vi "Elevator_with_Semaphore.vi"() -> ()   [LabVIEW 2018]
uses:
  Elevator Constants.ctl
  Elevator Command.ctl
  Elevator Cabin.ctl
  Elevator Automate.ctl
  Elevator Panel.ctl
  Floors Schematic.ctl
panel:
  out "milliseconds to wait":u32=10
  out "# available":i32
  out "# waiting":i32
  out "size":i32
  out "# elements in Elevator Floor Queue":i32
  out "Position:Top":i32
  out "Elevator Floor Queue":u8[](array[numeric])
  out "Elevator Command Queue":T1[](array[typedef])
  in  "Elevator Automate":T2={"Elevator Panel Array"=[FALSE, FALSE, FALSE, FALSE, FALSE, FALSE, FALSE, FALSE, FALSE, FALSE, FALSE, FALSE], "Floor Array"=[FALSE, FALSE, FALSE, FALSE, FALSE, FALSE, FALSE, FALSE, FALSE, FALSE, FALSE, FALSE], "Elevator Command"=enum."Open Doors", "Target Floor"=0, "Forced Stop"=FALSE, "Cancel Delay"=FALSE, "Elevator Status"=enum."Stand By", "Update\nTarget Floor"=FALSE, "Take a Call"=FALSE, "Add Floor\nto Queue"=FALSE}
  in  "Elevator Panel":T3
  in  "Floors Schematic":T4={"Call 1"=FALSE, "Call 2"=FALSE, "Call 3"=FALSE, "Call 4"=FALSE, "Call 5"=FALSE, "Call 6"=FALSE, "Call 7"=FALSE, "Call 8"=FALSE, "Call 9"=FALSE, "Call 10"=FALSE, "Call 11"=FALSE, "Call 12"=FALSE, "Floor Position"=[0, 0, 0, 0, 0, 0, 0, 0, 0, 0, 0, 0]}
  in  "STOP":bool
  out "Elevator Cabin":T5 scale=0.0..100.0
  # "Данная версия программы не является рабоей!"
  # "12"
  # "11"
  # "10"
  # "9"
  # "8"
  # "7"
  # "6"
  # "5"
  # "4"
  # "3"
  # "2"
  # "1"
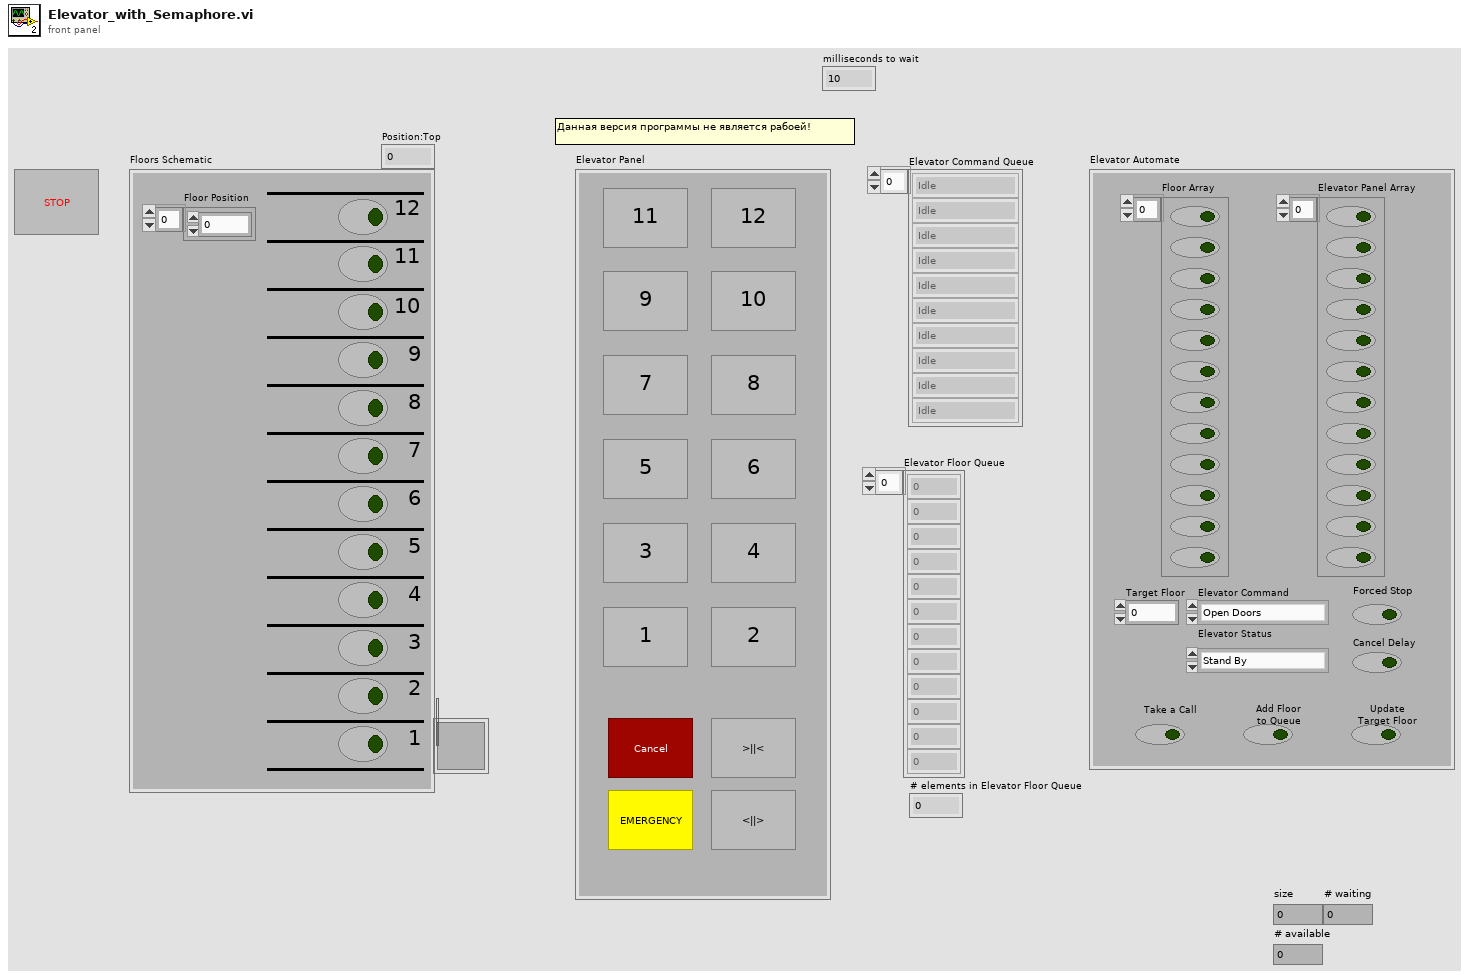
[diagram p1: front panel]
types:
  T1 = typedef "Elevator Command.ctl" = enum16{"Idle", "Short Delay", "Long Delay", "Cancel Delay", "Open Doors", "Close Doors", "Going Up", "Going Down", "Unpress Button"}
  T2 = typedef "Elevator Automate.ctl" = cluster{"Elevator Panel Array":bool[], "Floor Array":bool[], "Elevator Command":T1, "Target Floor":u8, "Forced Stop":bool, "Cancel Delay":bool, "Elevator Status":enum16{"Stand By", "Stop", "Going Up", "Going Down", "Cancel"}, "Update\nTarget Floor":bool, "Take a Call":bool, "Add Floor\nto Queue":bool}
  T3 = typedef "Elevator Panel.ctl" = cluster{"Open Doors":bool, "Close Doors":bool, "Floor 2":bool, "Floor 1":bool, "Floor 3":bool, "Floor 4":bool, "Floor 5":bool, "Floor 6":bool, "Floor 7":bool, "Floor 8":bool, "Floor 9":bool, "Floor 10":bool, "Floor 11":bool, "Floor 12":bool, "Emergency":bool, "Cancel":bool}
  T4 = typedef "Floors Schematic.ctl" = cluster{"Call 1":bool, "Call 2":bool, "Call 3":bool, "Call 4":bool, "Call 5":bool, "Call 6":bool, "Call 7":bool, "Call 8":bool, "Call 9":bool, "Call 10":bool, "Call 11":bool, "Call 12":bool, "Floor Position":i16[]}
  T5 = typedef "Elevator Cabin.ctl" = u8
  T6 = enum16{"Stand By", "Stop", "Going Up", "Going Down", "Cancel"}
  T7 = enum8{"Enabled", "Disabled", "Disabled and Grayed Out"}
  T8 = typedef "Semaphore RefNum" = refnum<k1>
  T9 = typedef "Elevator Constants.ctl" = u8
  T10 = enum16{"Stand By", "Stop", "Going Up", "Going Down"}
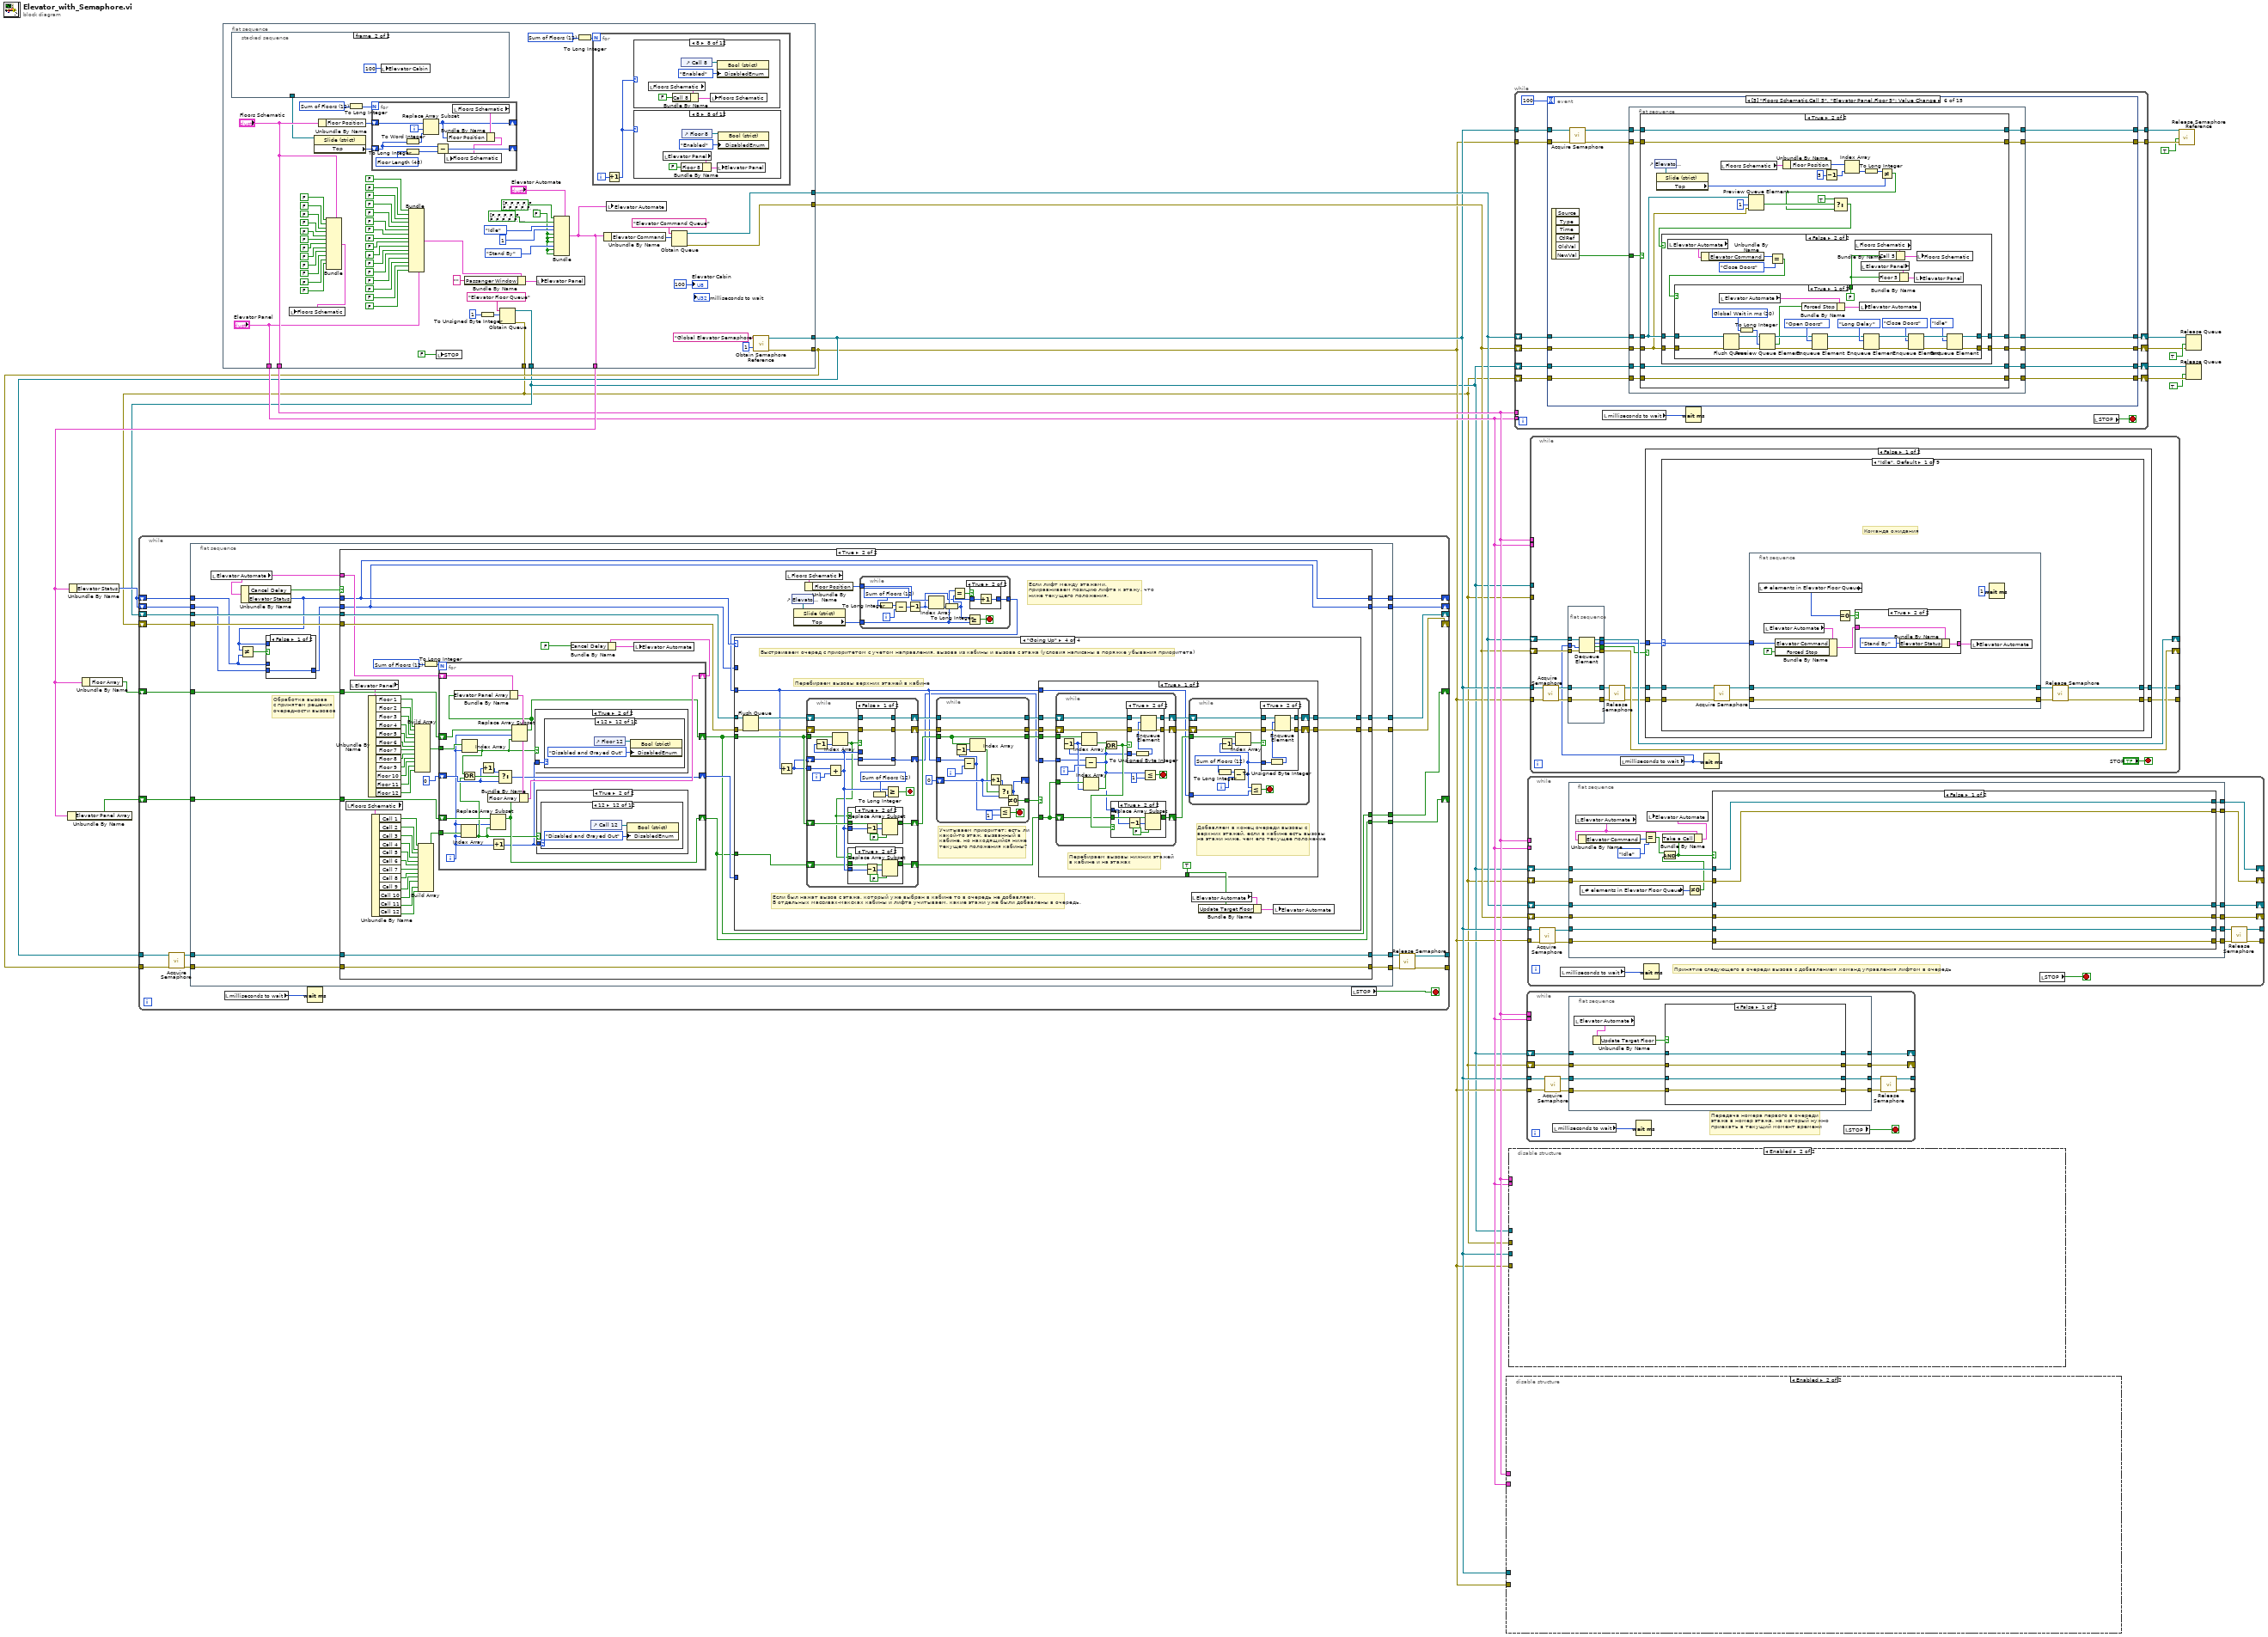
[diagram p0: block diagram]
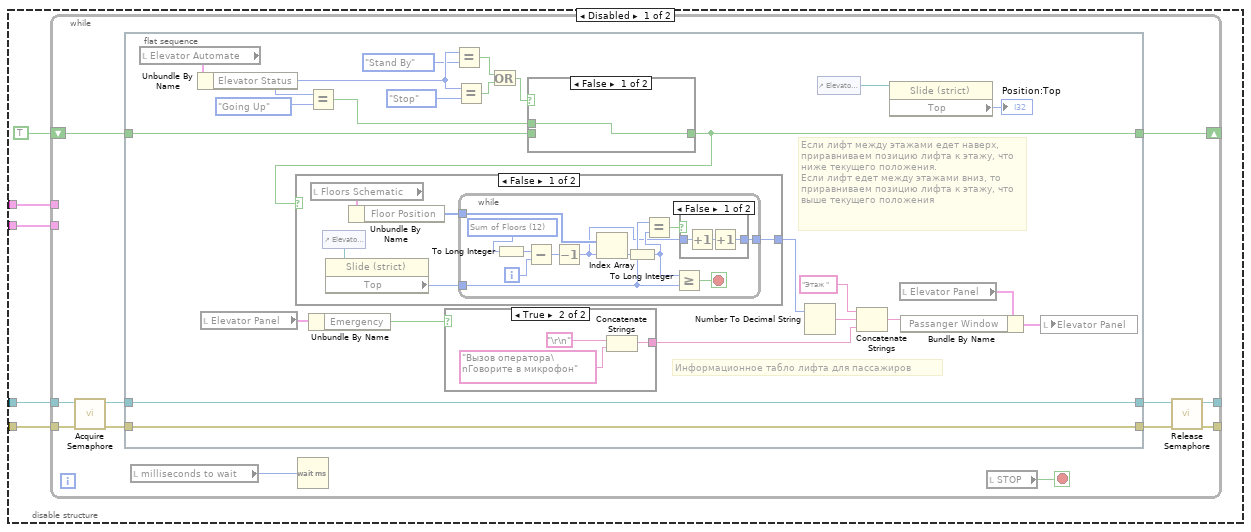
[diagram p2: hidden frame]
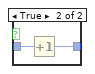
[diagram p4: hidden frame]
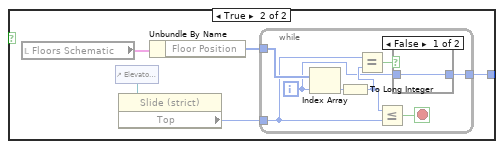
[diagram p5: hidden frame]
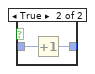
[diagram p6: hidden frame]
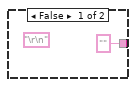
[diagram p7: hidden frame]
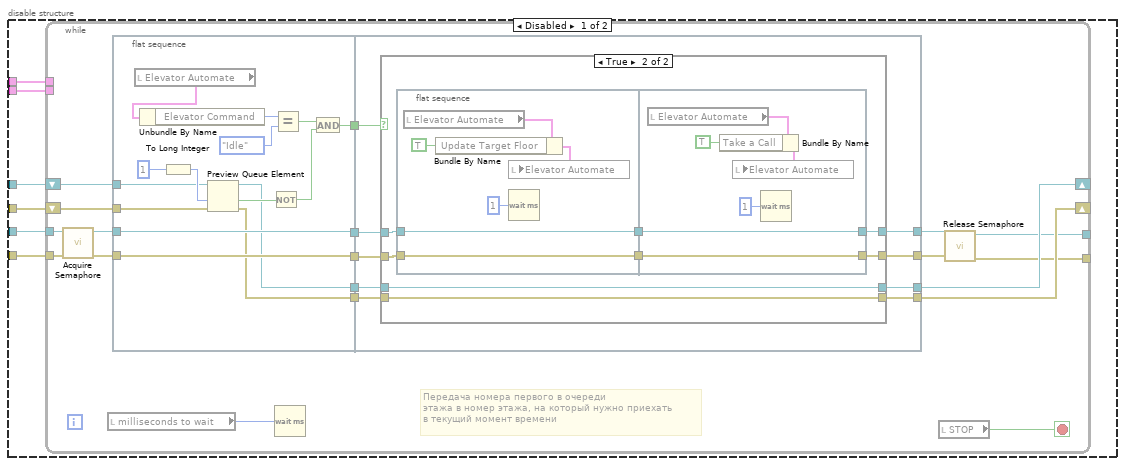
[diagram p8: hidden frame]
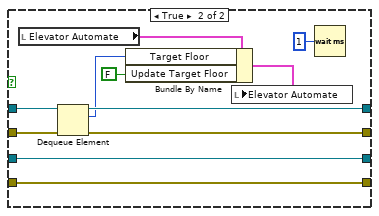
[diagram p10: hidden frame]
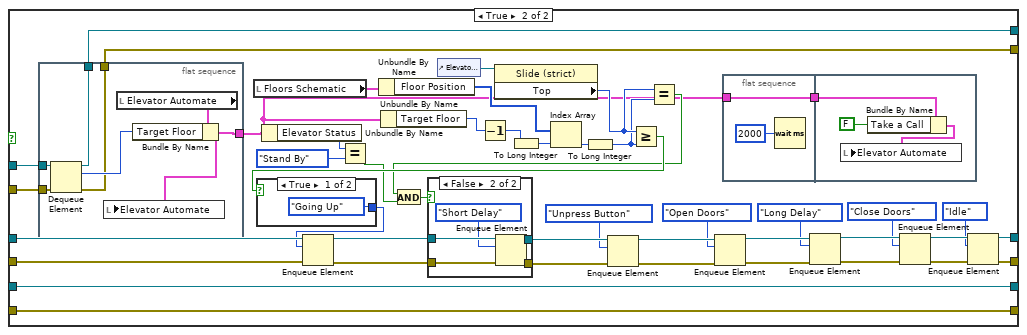
[diagram p11: hidden frame]
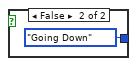
[diagram p13: hidden frame]
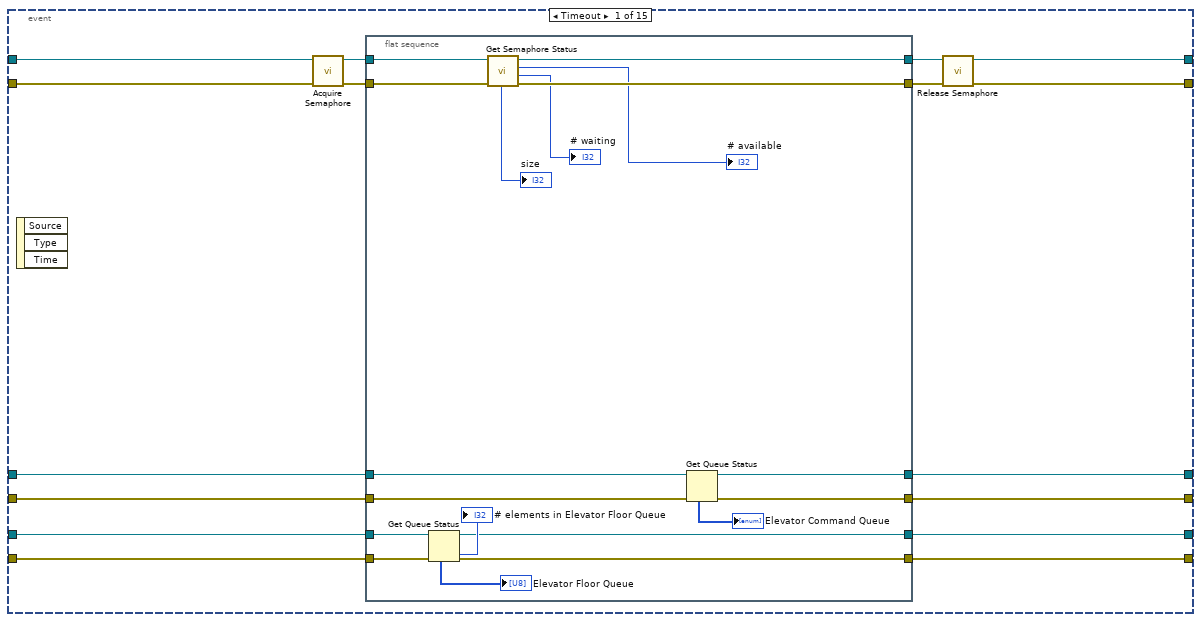
[diagram p14: hidden frame]
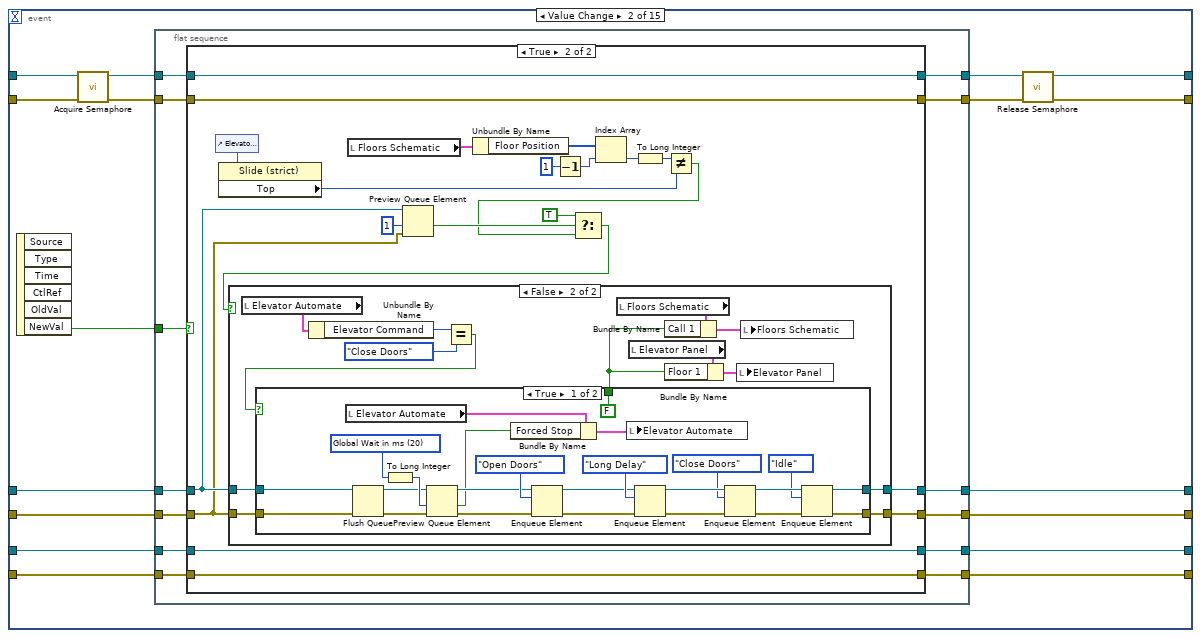
[diagram p15: hidden frame]
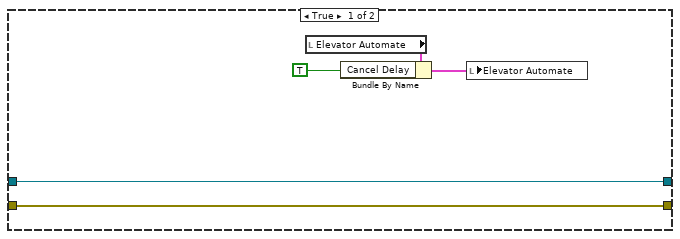
[diagram p17: hidden frame]
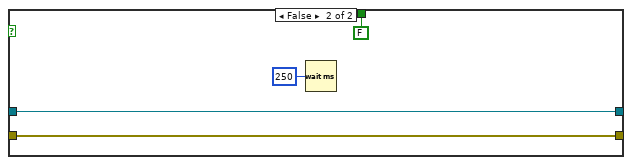
[diagram p18: hidden frame]
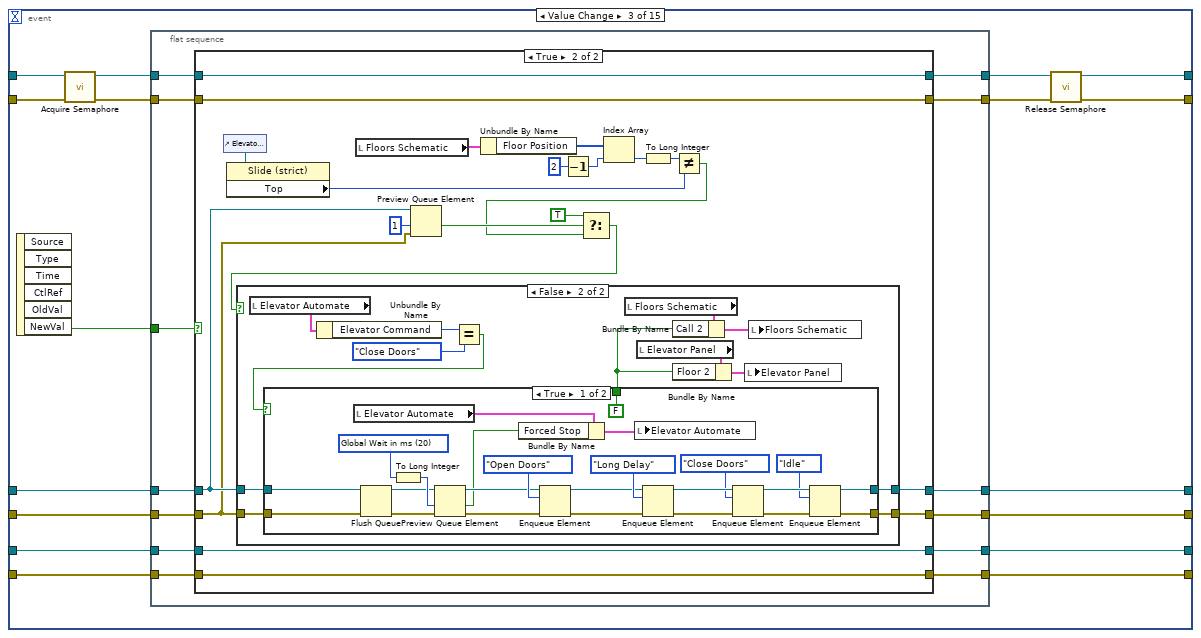
[diagram p19: hidden frame]
diagram:
  n1 = Unbundle By Name(w13) -> ("Elevator Panel Array"=w20:bool[])
  n2 = Unbundle By Name(w13) -> ("Elevator Status"=w12:T6)
  n3 = Unbundle By Name(w13) -> ("Floor Array"=w21:bool[])
  n4 = while {
    shift-right: [w38] -> _
    shift-left: w20 -> [w41]
    shift-right: [w37] -> _
    shift-left: w21 -> [w42]
    shift-right: [w35] -> _
    shift-left: w1 -> [w40]
    shift-right: [w36] -> _
    shift-left: w2 -> [w39]
    shift-right: [w34] -> _
    shift-left: w12 -> [w31]
    shift-right: [w32] -> _
    shift-left: w12 -> [w33]
    tunnel: w4 -> [w30]
    tunnel: w3 -> [w29]
    tunnel: [w24] -> _
    tunnel: [w23] -> _
    stop <- w43 stop-if-true
    n5 = call <vilib>:"Acquire Semaphore.vi"("error in (no error)"=w29, "semaphore"=w30) -> ("error out"=w28:errorcluster, "semaphore out"=w27:T8)  [unwired: 3 in, 1 out]
    n6 = flat-sequence {
      tunnel: [w59] -> w38
      tunnel: [w58] -> w37
      tunnel: [w57] -> w36
      tunnel: [w56] -> w35
      tunnel: [w55] -> w34
      tunnel: [w50] -> w32
      tunnel: w42 -> [w64]
      tunnel: w41 -> [w63]
      tunnel: w40 -> [w62]
      tunnel: w39 -> [w61]
      tunnel: w33 -> [w52]
      tunnel: w31 -> [w49]
      tunnel: w28 -> [w46]
      tunnel: w27 -> [w47]
      tunnel: [w45] -> w26
      tunnel: [w44] -> w25
      frame #0 {
        # "Обработка вызова\nс принятем решения\nочередности вызовов"
        n7 = local read "Elevator Automate"() -> (w54:T2)
        n8 = Unbundle By Name(w54) -> ("Cancel Delay"=w60:bool, "Elevator Status"=w51:T6)
        n9 = Not Equal?(x=w51, y=w52) -> (x != y?=w53:bool)
        n10 = case shown="False" w53 {
          tunnel: w51 -> [_ _]
          tunnel: w52 -> [_ w66]
          tunnel: w49 -> [w65 _]
          tunnel: [w65 w66] -> w48
          frame False {
          }
          frame True {
          }
        }
        n11 = case shown="True" w60 {
          tunnel: w64 -> [w71 w127]
          tunnel: w63 -> [w72 w126]
          tunnel: w62 -> [w73 w95]
          tunnel: w61 -> [w74 w94]
          tunnel: w51 -> [w70 w89]
          tunnel: [w74 w92] -> w57
          tunnel: [w73 w91] -> w56
          tunnel: [w72 w82] -> w59
          tunnel: [w71 w83] -> w58
          tunnel: w48 -> [w69 w81]
          tunnel: [w69 w81] -> w55
          tunnel: w54 -> [_ w90]
          tunnel: [w70 w89] -> w50
          tunnel: w47 -> [w68 w76]
          tunnel: w46 -> [w67 w75]
          tunnel: [w68 w76] -> w45
          tunnel: [w67 w75] -> w44
          frame False {
          }
          frame True {
            w97 = T9 12 items=["Floor Length"=48, "Sum of Floors"=12, "Floor Step in ms"=63, "Elevator Door Step in ms"=30, "Global Wait in ms"=20, "Event Wait in ms"=100] ("Elevator Constants")
            # "Если лифт между этажами,\nприравниваем позицию лифта к этажу, что ниже текущего положения."
            n12 = local read "Floors Schematic"() -> (w98:T4)
            n13 = local read "Elevator Panel"() -> (w99:T3)
            n14 = Unbundle By Name(w99) -> ("Floor 1"=w125:bool, "Floor 2"=w124:bool, "Floor 3"=w123:bool, "Floor 4"=w122:bool, "Floor 5"=w121:bool, "Floor 6"=w120:bool, "Floor 7"=w119:bool, "Floor 8"=w118:bool, "Floor 9"=w117:bool, "Floor 10"=w116:bool, "Floor 11"=w115:bool, "Floor 12"=w114:bool)
            n15 = Unbundle By Name(w98) -> ("Call 1"=w100:bool, "Call 2"=w112:bool, "Call 3"=w111:bool, "Call 4"=w110:bool, "Call 5"=w109:bool, "Call 6"=w108:bool, "Call 7"=w107:bool, "Call 8"=w106:bool, "Call 9"=w105:bool, "Call 10"=w104:bool, "Call 11"=w103:bool, "Call 12"=w102:bool)
            n16 = Build Array(w125, w124, w123, w122, w121, w120, w119, w118, w117, w116, w115, w114) -> (w113:bool[])
            n17 = Build Array(w100, w112, w111, w110, w109, w108, w107, w106, w105, w104, w103, w102) -> (w101:bool[])
            n18 = To Long Integer(number=w97) -> (32bit integer=w96:i32)
            n19 = for {
              N: w96 -> [_]
              tunnel: w113 -> [w998]
              tunnel: w101 -> [w997]
              shift-right: [w987] -> w82
              shift-left: w126 -> [w993]
              shift-right: [w988] -> w83
              shift-left: w127 -> [w994]
              shift-right: [w995] -> w84
              shift-left: w90 -> [w982]
              shift-right: [w990] -> w88
              shift-left: 0 -> [w989]
              i -> [w984]
              n20 = Index Array(array=w997, index=w984) -> (element=w986:bool)
              n21 = Index Array(array=w998, index=w984) -> (element=w985:bool)
              n22 = Or(x=w985, y=w986) -> (x .or. y?=w992:bool)
              n23 = Increment(x=w989) -> (x+1=w991:i32)
              n24 = Replace Array Subset(array=w993, new element=w986, index=w984) -> (w987:bool[])
              n25 = Increment(x=w984) -> (x+1=w983:i32)
              n26 = Select(t=w991, s=w992, f=w989) -> (s? t:f=w990:i32)
              n27 = Replace Array Subset(array=w994, new element=w985, index=w984) -> (w988:bool[])
              n28 = Bundle By Name(cluster=w982, "Elevator Panel Array"=w988) -> (w996:T2)
              n29 = Bundle By Name(cluster=w996, "Floor Array"=w987) -> (w995:T2)
              n30 = case shown="True" w985 {
                tunnel: w983 -> [_ w1024]
                frame False {
                }
                frame True {
                  n31 = case shown="12" w1024 {
                    frame 1, Default {
                      n32 = control-ref of="Floor 1"() -> (w1026:refnum<vi>)
                      n33 = property class="Bool (strict)"(reference=w1026, "DisabledEnum"=T7."Disabled and Grayed Out" ("Disabled")) -> ()  [unwired: 1 in, 2 out]
                    }
                    frame 2 {
                      n34 = control-ref of="Floor 2"() -> (w1028:refnum<vi>)
                      n35 = property class="Bool (strict)"(reference=w1028, "DisabledEnum"=T7."Disabled and Grayed Out" ("Disabled")) -> ()  [unwired: 1 in, 2 out]
                    }
                    frame 3 {
                      n36 = control-ref of="Floor 3"() -> (w1030:refnum<vi>)
                      n37 = property class="Bool (strict)"(reference=w1030, "DisabledEnum"=T7."Disabled and Grayed Out" ("Disabled")) -> ()  [unwired: 1 in, 2 out]
                    }
                    frame 4 {
                      n38 = control-ref of="Floor 4"() -> (w1032:refnum<vi>)
                      n39 = property class="Bool (strict)"(reference=w1032, "DisabledEnum"=T7."Disabled and Grayed Out" ("Disabled")) -> ()  [unwired: 1 in, 2 out]
                    }
                    frame 5 {
                      n40 = control-ref of="Floor 5"() -> (w1034:refnum<vi>)
                      n41 = property class="Bool (strict)"(reference=w1034, "DisabledEnum"=T7."Disabled and Grayed Out" ("Disabled")) -> ()  [unwired: 1 in, 2 out]
                    }
                    frame 6 {
                      n42 = control-ref of="Floor 6"() -> (w1036:refnum<vi>)
                      n43 = property class="Bool (strict)"(reference=w1036, "DisabledEnum"=T7."Disabled and Grayed Out" ("Disabled")) -> ()  [unwired: 1 in, 2 out]
                    }
                    frame 7 {
                      n44 = control-ref of="Floor 7"() -> (w1038:refnum<vi>)
                      n45 = property class="Bool (strict)"(reference=w1038, "DisabledEnum"=T7."Disabled and Grayed Out" ("Disabled")) -> ()  [unwired: 1 in, 2 out]
                    }
                    frame 8 {
                      n46 = control-ref of="Floor 8"() -> (w1040:refnum<vi>)
                      n47 = property class="Bool (strict)"(reference=w1040, "DisabledEnum"=T7."Disabled and Grayed Out" ("Disabled")) -> ()  [unwired: 1 in, 2 out]
                    }
                    frame 9 {
                      n48 = control-ref of="Floor 9"() -> (w1042:refnum<vi>)
                      n49 = property class="Bool (strict)"(reference=w1042, "DisabledEnum"=T7."Disabled and Grayed Out" ("Disabled")) -> ()  [unwired: 1 in, 2 out]
                    }
                    frame 10 {
                      n50 = control-ref of="Floor 10"() -> (w1044:refnum<vi>)
                      n51 = property class="Bool (strict)"(reference=w1044, "DisabledEnum"=T7."Disabled and Grayed Out" ("Disabled")) -> ()  [unwired: 1 in, 2 out]
                    }
                    frame 11 {
                      n52 = control-ref of="Floor 11"() -> (w1046:refnum<vi>)
                      n53 = property class="Bool (strict)"(reference=w1046, "DisabledEnum"=T7."Disabled and Grayed Out" ("Disabled")) -> ()  [unwired: 1 in, 2 out]
                    }
                    frame 12 {
                      n54 = control-ref of="Floor 12"() -> (w1048:refnum<vi>)
                      n55 = property class="Bool (strict)"(reference=w1048, "DisabledEnum"=T7."Disabled and Grayed Out" ("Disabled")) -> ()  [unwired: 1 in, 2 out]
                    }
                  }
                }
              }
              n56 = case shown="True" w986 {
                tunnel: w983 -> [_ w999]
                frame False {
                }
                frame True {
                  n57 = case shown="12" w999 {
                    frame 1, Default {
                      n58 = control-ref of="Call 1"() -> (w1001:refnum<vi>)
                      n59 = property class="Bool (strict)"(reference=w1001, "DisabledEnum"=T7."Disabled and Grayed Out" ("Disabled")) -> ()  [unwired: 1 in, 2 out]
                    }
                    frame 2 {
                      n60 = control-ref of="Call 2"() -> (w1003:refnum<vi>)
                      n61 = property class="Bool (strict)"(reference=w1003, "DisabledEnum"=T7."Disabled and Grayed Out" ("Disabled")) -> ()  [unwired: 1 in, 2 out]
                    }
                    frame 3 {
                      n62 = control-ref of="Call 3"() -> (w1005:refnum<vi>)
                      n63 = property class="Bool (strict)"(reference=w1005, "DisabledEnum"=T7."Disabled and Grayed Out" ("Disabled")) -> ()  [unwired: 1 in, 2 out]
                    }
                    frame 4 {
                      n64 = control-ref of="Call 4"() -> (w1007:refnum<vi>)
                      n65 = property class="Bool (strict)"(reference=w1007, "DisabledEnum"=T7."Disabled and Grayed Out" ("Disabled")) -> ()  [unwired: 1 in, 2 out]
                    }
                    frame 5 {
                      n66 = control-ref of="Call 5"() -> (w1009:refnum<vi>)
                      n67 = property class="Bool (strict)"(reference=w1009, "DisabledEnum"=T7."Disabled and Grayed Out" ("Disabled")) -> ()  [unwired: 1 in, 2 out]
                    }
                    frame 6 {
                      n68 = control-ref of="Call 6"() -> (w1011:refnum<vi>)
                      n69 = property class="Bool (strict)"(reference=w1011, "DisabledEnum"=T7."Disabled and Grayed Out" ("Disabled")) -> ()  [unwired: 1 in, 2 out]
                    }
                    frame 7 {
                      n70 = control-ref of="Call 7"() -> (w1013:refnum<vi>)
                      n71 = property class="Bool (strict)"(reference=w1013, "DisabledEnum"=T7."Disabled and Grayed Out" ("Disabled")) -> ()  [unwired: 1 in, 2 out]
                    }
                    frame 8 {
                      n72 = control-ref of="Call 8"() -> (w1015:refnum<vi>)
                      n73 = property class="Bool (strict)"(reference=w1015, "DisabledEnum"=T7."Disabled and Grayed Out" ("Disabled")) -> ()  [unwired: 1 in, 2 out]
                    }
                    frame 9 {
                      n74 = control-ref of="Call 9"() -> (w1017:refnum<vi>)
                      n75 = property class="Bool (strict)"(reference=w1017, "DisabledEnum"=T7."Disabled and Grayed Out" ("Disabled")) -> ()  [unwired: 1 in, 2 out]
                    }
                    frame 10 {
                      n76 = control-ref of="Call 10"() -> (w1019:refnum<vi>)
                      n77 = property class="Bool (strict)"(reference=w1019, "DisabledEnum"=T7."Disabled and Grayed Out" ("Disabled")) -> ()  [unwired: 1 in, 2 out]
                    }
                    frame 11 {
                      n78 = control-ref of="Call 11"() -> (w1021:refnum<vi>)
                      n79 = property class="Bool (strict)"(reference=w1021, "DisabledEnum"=T7."Disabled and Grayed Out" ("Disabled")) -> ()  [unwired: 1 in, 2 out]
                    }
                    frame 12 {
                      n80 = control-ref of="Call 12"() -> (w1023:refnum<vi>)
                      n81 = property class="Bool (strict)"(reference=w1023, "DisabledEnum"=T7."Disabled and Grayed Out" ("Disabled")) -> ()  [unwired: 1 in, 2 out]
                    }
                  }
                }
              }
            }
            n82 = Bundle By Name(cluster=w84, "Cancel Delay"=FALSE ("Add Floor to Queue")) -> (w85:T2)
            n83 = local write "Elevator Automate"(w85) -> ()
            n84 = local read "Floors Schematic"() -> (w79:T4)
            n85 = control-ref of="Elevator Cabin"() -> (w80:refnum<vi>)
            n86 = property class="Slide (strict)"(reference=w80) -> ("Top"=w77:i32)  [unwired: 1 in, 2 out]
            n87 = Unbundle By Name(w79) -> ("Floor Position"=w78:i16[])
            n88 = while {
              tunnel: w78 -> [w137]
              tunnel: w77 -> [w135]
              tunnel: [w134] -> w87
              i -> [w132]
              stop <- w133 stop-if-true
              w130 = T9 12 items=["Floor Length"=48, "Sum of Floors"=12, "Floor Step in ms"=63, "Elevator Door Step in ms"=30, "Global Wait in ms"=20, "Event Wait in ms"=100] ("Elevator Constants")
              n89 = To Long Integer(number=w130) -> (32bit integer=w131:i32)
              n90 = Subtract(x=w131, y=w132) -> (x-y=w129:i32)
              n91 = Decrement(x=w129) -> (x-1=w128:i32)
              n92 = Index Array(array=w137, index=w128) -> (element=w138:i16)
              n93 = To Long Integer(number=w138) -> (32bit integer=w136:i32)
              n94 = Equal?(x=w135, y=w136) -> (x = y?=w139:bool)
              n95 = Greater Or Equal?(x=w136, y=w135) -> (x >= y?=w133:bool)
              n96 = case shown="True" w139 {
                tunnel: w128 -> [w140 w142]
                tunnel: [w140 w141] -> w134
                frame False {
                }
                frame True {
                  n97 = Increment(x=w142) -> (x+1=w141:i32)
                }
              }
            }
            n98 = case shown="\"Going Up\"" w89 {
              tunnel: w94 -> [w161 w281 w651 w827]
              tunnel: w95 -> [w160 w282 w652 w828]
              tunnel: w83 -> [w148 w286 w638 w830]
              tunnel: w82 -> [w146 w284 w639 w829]
              tunnel: w87 -> [w147 w285 w637 w811]
              tunnel: [w150 w288 w654 w832] -> w92
              tunnel: [w149 w287 w653 w831] -> w91
              tunnel: w81 -> [_ w283 _ _]
              tunnel: w88 -> [w143 _ _ _]
              frame "Stand By", Default {
                # "Если было одновременно несколько\nвызовов, то повторно обрабатываем\nочередь с учетом направления\nдвижения лифта"
                # "Перебираем вызовы верхних этажей в кабине"
                # "Перебираем вызовы на нижних этажах"
                # "Перебираем вызовы на верхних этажах"
                # "Перебираем вызовы нижних этажей в кабине"
                # "Выбираем приоритетный вызов"
                n99 = while {
                  tunnel: w148 -> [w177]
                  shift-right: [w174] -> w155
                  shift-left: w161 -> [w176]
                  shift-right: [w175] -> w154
                  shift-left: w160 -> [w178]
                  tunnel: w147 -> [w166]
                  tunnel: [w169] -> w153
                  i -> [w165]
                  stop <- w173 stop-if-true
                  w171 = T9 12 items=["Floor Length"=48, "Sum of Floors"=12, "Floor Step in ms"=63, "Elevator Door Step in ms"=30, "Global Wait in ms"=20, "Event Wait in ms"=100] ("Elevator Constants")
                  n100 = Add(x=w166, y=w165) -> (x+y=w167:i32)
                  n101 = Decrement(x=w167) -> (x-1=w168:i32)
                  n102 = Index Array(array=w177, index=w168) -> (element=w169:bool)
                  n103 = To Long Integer(number=w171) -> (32bit integer=w172:i32)
                  n104 = case shown="True" w169 {
                    tunnel: w176 -> [w180 w186]
                    tunnel: w178 -> [w179 w185]
                    tunnel: [w179 w184] -> w175
                    tunnel: [w180 w183] -> w174
                    tunnel: w167 -> [_ w182]
                    frame False {
                    }
                    frame True {
                      n105 = To Unsigned Byte Integer(number=w182) -> (unsigned 8bit integer=w181:u8)
                      n106 = Enqueue Element(queue=w186, element=w181, error in (no error)=w185) -> (queue out=w183:refnum<queue>, error out=w184:errorcluster)  [unwired: 1 in, 1 out]
                    }
                  }
                  n107 = Greater Or Equal?(x=w167, y=w172) -> (x >= y?=w170:bool)
                  n108 = Or(x=w169, y=w170) -> (x .or. y?=w173:bool)
                }
                n109 = Greater?(x=w143, y=1) -> (0:w145:bool)
                n110 = case shown="True" w145 {
                  frame True {
                    n111 = local read "Elevator Automate"() -> (w164:T2)
                    n112 = Bundle By Name(cluster=w164, "Cancel Delay"=TRUE ("Add Floor to Queue")) -> (w162:T2)
                    n113 = local write "Elevator Automate"(w162) -> ()
                  }
                  frame False {
                  }
                }
                n114 = case shown="False" w153 {
                  selector: w153 -> [w250 _]
                  tunnel: w154 -> [w248 w257]
                  tunnel: w155 -> [w249 w256]
                  tunnel: w147 -> [_ w255]
                  tunnel: w148 -> [_ w254]
                  tunnel: [w250 w253] -> w152
                  tunnel: [w249 w252] -> w157
                  tunnel: [w248 w251] -> w156
                  frame True {
                  }
                  frame False {
                    n115 = while {
                      tunnel: w254 -> [w269]
                      shift-right: [w266] -> w252
                      shift-left: w256 -> [w268]
                      shift-right: [w267] -> w251
                      shift-left: w257 -> [w270]
                      tunnel: w255 -> [w261]
                      tunnel: [w263] -> w253
                      i -> [w260]
                      stop <- w265 stop-if-true
                      n116 = Subtract(x=w261, y=w260) -> (x-y=w258:i32)
                      n117 = Decrement(x=w258) -> (x-1=w259:i32)
                      n118 = Index Array(array=w269, index=w259) -> (element=w263:bool)
                      n119 = case shown="True" w263 {
                        tunnel: w268 -> [w272 w278]
                        tunnel: w270 -> [w271 w277]
                        tunnel: [w271 w276] -> w267
                        tunnel: [w272 w275] -> w266
                        tunnel: w258 -> [_ w274]
                        frame False {
                        }
                        frame True {
                          n120 = To Unsigned Byte Integer(number=w274) -> (unsigned 8bit integer=w273:u8)
                          n121 = Enqueue Element(queue=w278, element=w273, error in (no error)=w277) -> (queue out=w275:refnum<queue>, error out=w276:errorcluster)  [unwired: 1 in, 1 out]
                        }
                      }
                      n122 = Less Or Equal?(x=w258, y=1) -> (x <= y?=w264:bool)
                      n123 = Or(x=w263, y=w264) -> (x .or. y?=w265:bool)
                    }
                  }
                }
                n124 = case shown="False" w152 {
                  selector: w152 -> [w218 _]
                  tunnel: w156 -> [w216 w225]
                  tunnel: w157 -> [w217 w224]
                  tunnel: w147 -> [_ w223]
                  tunnel: w146 -> [_ w222]
                  tunnel: [w218 w221] -> w151
                  tunnel: [w217 w220] -> w159
                  tunnel: [w216 w219] -> w158
                  frame True {
                  }
                  frame False {
                    n125 = while {
                      tunnel: w222 -> [w238]
                      shift-right: [w235] -> w220
                      shift-left: w224 -> [w237]
                      shift-right: [w236] -> w219
                      shift-left: w225 -> [w239]
                      tunnel: w223 -> [w229]
                      tunnel: [w230] -> w221
                      i -> [w228]
                      stop <- w234 stop-if-true
                      w232 = T9 12 items=["Floor Length"=48, "Sum of Floors"=12, "Floor Step in ms"=63, "Elevator Door Step in ms"=30, "Global Wait in ms"=20, "Event Wait in ms"=100] ("Elevator Constants")
                      n126 = Add(x=w229, y=w228) -> (x+y=w227:i32)
                      n127 = Decrement(x=w227) -> (x-1=w226:i32)
                      n128 = Index Array(array=w238, index=w226) -> (element=w230:bool)
                      n129 = To Long Integer(number=w232) -> (32bit integer=w233:i32)
                      n130 = case shown="True" w230 {
                        tunnel: w237 -> [w241 w247]
                        tunnel: w239 -> [w240 w246]
                        tunnel: [w240 w245] -> w236
                        tunnel: [w241 w244] -> w235
                        tunnel: w227 -> [_ w243]
                        frame False {
                        }
                        frame True {
                          n131 = To Unsigned Byte Integer(number=w243) -> (unsigned 8bit integer=w242:u8)
                          n132 = Enqueue Element(queue=w247, element=w242, error in (no error)=w246) -> (queue out=w244:refnum<queue>, error out=w245:errorcluster)  [unwired: 1 in, 1 out]
                        }
                      }
                      n133 = Greater Or Equal?(x=w227, y=w233) -> (x >= y?=w231:bool)
                      n134 = Or(x=w230, y=w231) -> (x .or. y?=w234:bool)
                    }
                  }
                }
                n135 = case shown="False" w151 {
                  tunnel: w158 -> [w187 w194]
                  tunnel: w159 -> [w188 w193]
                  tunnel: w146 -> [_ w192]
                  tunnel: [w188 w191] -> w150
                  tunnel: [w187 w190] -> w149
                  tunnel: w147 -> [_ w189]
                  frame True {
                  }
                  frame False {
                    n136 = while {
                      tunnel: w192 -> [w206]
                      shift-right: [w203] -> w191
                      shift-left: w193 -> [w205]
                      shift-right: [w204] -> w190
                      shift-left: w194 -> [w207]
                      tunnel: [w200] -> _
                      tunnel: w189 -> [w196]
                      i -> [w197]
                      stop <- w202 stop-if-true
                      n137 = Subtract(x=w196, y=w197) -> (x-y=w195:i32)
                      n138 = Decrement(x=w195) -> (x-1=w198:i32)
                      n139 = Index Array(array=w206, index=w198) -> (element=w200:bool)
                      n140 = case shown="True" w200 {
                        tunnel: w205 -> [w209 w215]
                        tunnel: w207 -> [w208 w214]
                        tunnel: [w208 w213] -> w204
                        tunnel: [w209 w212] -> w203
                        tunnel: w195 -> [_ w211]
                        frame False {
                        }
                        frame True {
                          n141 = To Unsigned Byte Integer(number=w211) -> (unsigned 8bit integer=w210:u8)
                          n142 = Enqueue Element(queue=w215, element=w210, error in (no error)=w214) -> (queue out=w212:refnum<queue>, error out=w213:errorcluster)  [unwired: 1 in, 1 out]
                        }
                      }
                      n143 = Less Or Equal?(x=w195, y=1) -> (x <= y?=w201:bool)
                      n144 = Or(x=w200, y=w201) -> (x .or. y?=w202:bool)
                    }
                  }
                }
              }
              frame "Stop" {
                # "Выстраиваем очеред с приоритетом с учетом направления, вызова из кабины и вызова с этажа (условия написаны в поряжке убывания приоритета)"
                n145 = Flush Queue(queue=w281, error in (no error)=w282) -> (queue out=w280:refnum<queue>, error out=w279:errorcluster)  [unwired: 1 out]
                n146 = case shown="\"Going Down\"" w283 {
                  tunnel: w280 -> [w311 w481]
                  tunnel: w279 -> [w310 w480]
                  tunnel: [w309 w479] -> w288
                  tunnel: [w308 w478] -> w287
                  tunnel: w286 -> [w306 w476]
                  tunnel: w285 -> [w290 w461]
                  tunnel: w284 -> [w302 w473]
                  frame "Going Up", Default {
                    # "Учитываем приоритет: есть ли\nкакой-то этаж, вызванный в кабине, но находящийся ниже\nтекущего положения кабины?"
                    # "Учитываем, на каком этаже\nсейчас находится лифт и убираем его из массивов-масок кабины и лифта"
                    # "Если был нажат вызов с этажа дома, который уже выбран в кабине то в очередь не добавляем.\nВ отдельных массивах-максках кабины и лифта учитываем, какие этажи уже были добавлены в очередь."
                    # "Перебираем вызовы верхних этажей в кабине"
                    n147 = Decrement(x=w290) -> (x-1=w301:i32)
                    n148 = Increment(x=w290) -> (x+1=w291:i32)
                    n149 = Replace Array Subset(array=w306, new element=FALSE ("new element/subarray"), index=w301) -> (w305:bool[])
                    n150 = Replace Array Subset(array=w302, new element=FALSE ("new element/subarray"), index=w301) -> (w303:bool[])
                    n151 = while {
                      tunnel: w305 -> [w429]
                      shift-right: [w436] -> w294
                      shift-left: w311 -> [w438]
                      shift-right: [w437] -> w297
                      shift-left: w310 -> [w439]
                      tunnel: w291 -> [w431]
                      shift-right: [w428] -> w299
                      shift-left: w305 -> [w427]
                      shift-right: [w425] -> w300
                      shift-left: w303 -> [w423]
                      shift-right: [w422] -> w289
                      shift-left: w291 -> [w421]
                      i -> [w433]
                      stop <- w432 stop-if-true
                      w430 = T9 12 items=["Floor Length"=48, "Sum of Floors"=12, "Floor Step in ms"=63, "Elevator Door Step in ms"=30, "Global Wait in ms"=20, "Event Wait in ms"=100] ("Elevator Constants")
                      n152 = Add(x=w431, y=w433) -> (x+y=w426:i32)
                      n153 = Decrement(x=w426) -> (x-1=w434:i32)
                      n154 = Index Array(array=w429, index=w434) -> (element=w424:bool)
                      n155 = case shown="True" w424 {
                        tunnel: w426 -> [_ w447]
                        tunnel: [w446 w449] -> w428
                        tunnel: w427 -> [w446 w448]
                        frame False {
                        }
                        frame True {
                          n156 = Decrement(x=w447) -> (x-1=w451:i32)
                          n157 = Replace Array Subset(array=w448, new element=FALSE ("new element/subarray"), index=w451) -> (w449:bool[])
                        }
                      }
                      n158 = case shown="True" w424 {
                        tunnel: [w440 w443] -> w425
                        tunnel: w423 -> [w440 w442]
                        tunnel: w426 -> [_ w441]
                        frame False {
                        }
                        frame True {
                          n159 = Decrement(x=w441) -> (x-1=w445:i32)
                          n160 = Replace Array Subset(array=w442, new element=FALSE ("new element/subarray"), index=w445) -> (w443:bool[])
                        }
                      }
                      n161 = case shown="True" w424 {
                        tunnel: w438 -> [w454 w460]
                        tunnel: w439 -> [w453 w459]
                        tunnel: [w453 w458] -> w437
                        tunnel: [w454 w457] -> w436
                        tunnel: w426 -> [_ w455]
                        tunnel: [w452 w455] -> w422
                        tunnel: w421 -> [w452 _]
                        frame False {
                        }
                        frame True {
                          n162 = To Unsigned Byte Integer(number=w455) -> (unsigned 8bit integer=w456:u8)
                          n163 = Enqueue Element(queue=w460, element=w456, error in (no error)=w459) -> (queue out=w457:refnum<queue>, error out=w458:errorcluster)  [unwired: 1 in, 1 out]
                        }
                      }
                      n164 = To Long Integer(number=w430) -> (32bit integer=w435:i32)
                      n165 = Greater Or Equal?(x=w426, y=w435) -> (x >= y?=w432:bool)
                    }
                    n166 = while {
                      tunnel: w299 -> [w415]
                      tunnel: [w415] -> w298
                      tunnel: w297 -> [w420]
                      tunnel: [w420] -> w296
                      tunnel: [w419] -> w295
                      tunnel: w294 -> [w419]
                      tunnel: w290 -> [w417]
                      shift-right: [w411] -> _
                      shift-left: 0 -> [w412]
                      tunnel: [w410] -> w292
                      i -> [w416]
                      stop <- w408 stop-if-true
                      n167 = Decrement(x=w417) -> (x-1=w418:i32)
                      n168 = Subtract(x=w418, y=w416) -> (x-y=w407:i32)
                      n169 = Decrement(x=w407) -> (x-1=w414:i32)
                      n170 = Index Array(array=w415, index=w414) -> (element=w406:bool)
                      n171 = Increment(x=w412) -> (x+1=w413:i32)
                      n172 = Less Or Equal?(x=w407, y=1) -> (x <= y?=w408:bool)
                      n173 = Select(t=w413, s=w406, f=w412) -> (s? t:f=w411:i32)
                      n174 = Not Equal To 0?(x=w411) -> (x != 0?=w410:bool)
                    }
                    n175 = case shown="False" w292 {
                      tunnel: [w320 w377] -> w309
                      tunnel: [w319 w376] -> w308
                      tunnel: w300 -> [w317 w381]
                      tunnel: w298 -> [w316 w380]
                      tunnel: w296 -> [w315 w379]
                      tunnel: w295 -> [w314 w378]
                      tunnel: w289 -> [w312 _]
                      tunnel: w290 -> [w313 _]
                      frame True {
                        # "Перебираем вызовы нижних этажей, начиная с самого высокого этажа, вызванного в кабине"
                        # "Если есть такой этаж, то добавляем в конец очереди вызовы верхних этажей дома"
                        n176 = while {
                          tunnel: w316 -> [w360]
                          shift-right: [w357] -> w322
                          shift-left: w314 -> [w359]
                          shift-right: [w358] -> w321
                          shift-left: w315 -> [w361]
                          tunnel: w312 -> [w350]
                          tunnel: w317 -> [w354]
                          shift-right: [w347] -> w318
                          shift-left: w317 -> [w348]
                          i -> [w352]
                          stop <- w355 stop-if-true
                          n177 = Decrement(x=w350) -> (x-1=w345:i32)
                          n178 = Subtract(x=w345, y=w352) -> (x-y=w344:i32)
                          n179 = Decrement(x=w344) -> (x-1=w351:i32)
                          n180 = Index Array(array=w360, index=w351) -> (element=w346:bool)
                          n181 = Index Array(array=w354, index=w351) -> (element=w353:bool)
                          n182 = Or(x=w346, y=w353) -> (x .or. y?=w349:bool)
                          n183 = case shown="True" w349 {
                            tunnel: w344 -> [_ w366]
                            tunnel: [w362 w364] -> w347
                            tunnel: w348 -> [w362 w363]
                            frame False {
                            }
                            frame True {
                              n184 = Decrement(x=w366) -> (x-1=w367:i32)
                              n185 = Replace Array Subset(array=w363, new element=FALSE ("new element/subarray"), index=w367) -> (w364:bool[])
                            }
                          }
                          n186 = case shown="True" w349 {
                            tunnel: w359 -> [w369 w375]
                            tunnel: w361 -> [w368 w374]
                            tunnel: [w368 w373] -> w358
                            tunnel: [w369 w372] -> w357
                            tunnel: w344 -> [_ w370]
                            frame False {
                            }
                            frame True {
                              n187 = To Unsigned Byte Integer(number=w370) -> (unsigned 8bit integer=w371:u8)
                              n188 = Enqueue Element(queue=w375, element=w371, error in (no error)=w374) -> (queue out=w372:refnum<queue>, error out=w373:errorcluster)  [unwired: 1 in, 1 out]
                            }
                          }
                          n189 = Less Or Equal?(x=w344, y=1) -> (x <= y?=w355:bool)
                        }
                        n190 = while {
                          tunnel: w318 -> [w334]
                          shift-right: [w331] -> w320
                          shift-left: w322 -> [w333]
                          shift-right: [w332] -> w319
                          shift-left: w321 -> [w335]
                          tunnel: w313 -> [w324]
                          i -> [w329]
                          stop <- w323 stop-if-true
                          w326 = T9 12 items=["Floor Length"=48, "Sum of Floors"=12, "Floor Step in ms"=63, "Elevator Door Step in ms"=30, "Global Wait in ms"=20, "Event Wait in ms"=100] ("Elevator Constants")
                          n191 = To Long Integer(number=w326) -> (32bit integer=w325:i32)
                          n192 = Subtract(x=w325, y=w329) -> (x-y=w328:i32)
                          n193 = Decrement(x=w328) -> (x-1=w327:i32)
                          n194 = Index Array(array=w334, index=w327) -> (element=w330:bool)
                          n195 = Less Or Equal?(x=w328, y=w324) -> (x <= y?=w323:bool)
                          n196 = case shown="True" w330 {
                            tunnel: w333 -> [w337 w343]
                            tunnel: w335 -> [w336 w342]
                            tunnel: [w336 w341] -> w332
                            tunnel: [w337 w340] -> w331
                            tunnel: w328 -> [_ w339]
                            frame False {
                            }
                            frame True {
                              n197 = To Unsigned Byte Integer(number=w339) -> (unsigned 8bit integer=w338:u8)
                              n198 = Enqueue Element(queue=w343, element=w338, error in (no error)=w342) -> (queue out=w340:refnum<queue>, error out=w341:errorcluster)  [unwired: 1 in, 1 out]
                            }
                          }
                        }
                      }
                      frame False {
                        # "Перебираем вызовы на нижних этажа дома, начиная с самого верхнего"
                        n199 = while {
                          tunnel: w380 -> [w396]
                          shift-right: [w393] -> w377
                          shift-left: w378 -> [w395]
                          shift-right: [w394] -> w376
                          shift-left: w379 -> [w397]
                          tunnel: w381 -> [w390]
                          i -> [w388]
                          stop <- w391 stop-if-true
                          w383 = T9 12 items=["Floor Length"=48, "Sum of Floors"=12, "Floor Step in ms"=63, "Elevator Door Step in ms"=30, "Global Wait in ms"=20, "Event Wait in ms"=100] ("Elevator Constants")
                          n200 = To Long Integer(number=w383) -> (32bit integer=w382:i32)
                          n201 = Subtract(x=w382, y=w388) -> (x-y=w384:i32)
                          n202 = Decrement(x=w384) -> (x-1=w387:i32)
                          n203 = Index Array(array=w396, index=w387) -> (element=w385:bool)
                          n204 = Index Array(array=w390, index=w387) -> (element=w389:bool)
                          n205 = Or(x=w385, y=w389) -> (x .or. y?=w386:bool)
                          n206 = case shown="True" w386 {
                            tunnel: w395 -> [w399 w405]
                            tunnel: w397 -> [w398 w404]
                            tunnel: [w398 w403] -> w394
                            tunnel: [w399 w402] -> w393
                            tunnel: w384 -> [_ w400]
                            frame False {
                            }
                            frame True {
                              n207 = To Unsigned Byte Integer(number=w400) -> (unsigned 8bit integer=w401:u8)
                              n208 = Enqueue Element(queue=w405, element=w401, error in (no error)=w404) -> (queue out=w402:refnum<queue>, error out=w403:errorcluster)  [unwired: 1 in, 1 out]
                            }
                          }
                          n209 = Less Or Equal?(x=w384, y=1) -> (x <= y?=w391:bool)
                        }
                      }
                    }
                  }
                  frame "Going Down" {
                    # "Учитываем приоритет: есть ли\nкакой-то этаж, вызванный в кабине, но находящийся выше\nтекущего положения кабины?"
                    # "Учитываем, на каком этаже\nсейчас находится лифт и убираем его из массивов-масок кабины и лифта"
                    # "Если был нажат вызов с этажа дома, который уже выбран в кабине то в очередь не добавляем.\nВ отдельных массивах-максках кабины и лифта учитываем, какие этажи уже были добавлены в очередь."
                    # "Перебираем вызовы нижних этажей в кабине"
                    n210 = Decrement(x=w461) -> (x-1=w472:i32)
                    n211 = Replace Array Subset(array=w476, new element=FALSE ("new element/subarray"), index=w472) -> (w475:bool[])
                    n212 = Replace Array Subset(array=w473, new element=FALSE ("new element/subarray"), index=w472) -> (w464:bool[])
                    n213 = while {
                      tunnel: w475 -> [w609]
                      shift-right: [w613] -> w467
                      shift-left: w481 -> [w615]
                      shift-right: [w614] -> w470
                      shift-left: w480 -> [w616]
                      tunnel: w461 -> [w610]
                      shift-right: [w608] -> w463
                      shift-left: w475 -> [w607]
                      shift-right: [w606] -> w462
                      shift-left: w464 -> [w605]
                      tunnel: w464 -> [w601]
                      i -> [w612]
                      stop <- w611 stop-if-true
                      n214 = Subtract(x=w610, y=w612) -> (x-y=w600:i32)
                      n215 = Decrement(x=w600) -> (x-1=w598:i32)
                      n216 = Index Array(array=w601, index=w598) -> (element=w599:bool)
                      n217 = Index Array(array=w609, index=w598) -> (element=w603:bool)
                      n218 = case shown="True" w603 {
                        tunnel: w600 -> [_ w624]
                        tunnel: [w623 w626] -> w608
                        tunnel: w607 -> [w623 w625]
                        frame False {
                        }
                        frame True {
                          n219 = Decrement(x=w624) -> (x-1=w628:i32)
                          n220 = Replace Array Subset(array=w625, new element=FALSE ("new element/subarray"), index=w628) -> (w626:bool[])
                        }
                      }
                      n221 = case shown="True" w603 {
                        tunnel: [w617 w620] -> w606
                        tunnel: w605 -> [w617 w619]
                        tunnel: w600 -> [_ w618]
                        frame False {
                        }
                        frame True {
                          n222 = Decrement(x=w618) -> (x-1=w622:i32)
                          n223 = Replace Array Subset(array=w619, new element=FALSE ("new element/subarray"), index=w622) -> (w620:bool[])
                        }
                      }
                      n224 = Or(x=w603, y=w599) -> (x .or. y?=w602:bool)
                      n225 = case shown="False" w602 {
                        tunnel: w615 -> [w630 w636]
                        tunnel: w616 -> [w629 w635]
                        tunnel: [w629 w634] -> w614
                        tunnel: [w630 w633] -> w613
                        tunnel: w600 -> [_ w631]
                        frame False {
                        }
                        frame True {
                          n226 = To Unsigned Byte Integer(number=w631) -> (unsigned 8bit integer=w632:u8)
                          n227 = Enqueue Element(queue=w636, element=w632, error in (no error)=w635) -> (queue out=w633:refnum<queue>, error out=w634:errorcluster)  [unwired: 1 in, 1 out]
                        }
                      }
                      n228 = Less Or Equal?(x=w600, y=1) -> (x <= y?=w611:bool)
                    }
                    n229 = while {
                      tunnel: w463 -> [w592]
                      tunnel: [w592] -> w471
                      tunnel: w470 -> [w597]
                      tunnel: [w597] -> w469
                      tunnel: [w596] -> w468
                      tunnel: w467 -> [w596]
                      tunnel: w461 -> [w594]
                      shift-right: [w588] -> _
                      shift-left: 0 -> [w589]
                      tunnel: [w587] -> w465
                      i -> [w593]
                      stop <- w586 stop-if-true
                      w584 = T9 12 items=["Floor Length"=48, "Sum of Floors"=12, "Floor Step in ms"=63, "Elevator Door Step in ms"=30, "Global Wait in ms"=20, "Event Wait in ms"=100] ("Elevator Constants")
                      n230 = Increment(x=w594) -> (x+1=w595:i32)
                      n231 = Add(x=w595, y=w593) -> (x+y=w585:i32)
                      n232 = Decrement(x=w585) -> (x-1=w591:i32)
                      n233 = Index Array(array=w592, index=w591) -> (element=w582:bool)
                      n234 = To Long Integer(number=w584) -> (32bit integer=w583:i32)
                      n235 = Increment(x=w589) -> (x+1=w590:i32)
                      n236 = Select(t=w590, s=w582, f=w589) -> (s? t:f=w588:i32)
                      n237 = Greater Or Equal?(x=w585, y=w583) -> (x >= y?=w586:bool)
                      n238 = Not Equal To 0?(x=w588) -> (x != 0?=w587:bool)
                    }
                    n239 = case shown="True" w465 {
                      tunnel: [w490 w554] -> w479
                      tunnel: [w489 w553] -> w478
                      tunnel: w463 -> [w482 _]
                      tunnel: w471 -> [w488 w557]
                      tunnel: w469 -> [w487 w556]
                      tunnel: w468 -> [w486 w555]
                      tunnel: w461 -> [w485 _]
                      tunnel: w462 -> [w484 w552]
                      frame True {
                        # "Если есть такой этаж, то добавляем в конец очереди сначала вызовы верхних этажей кабины, потом вызовы верхних этажей дома"
                        n240 = while {
                          tunnel: w488 -> [w530]
                          shift-right: [w527] -> w492
                          shift-left: w486 -> [w529]
                          shift-right: [w528] -> w491
                          shift-left: w487 -> [w531]
                          tunnel: w485 -> [w523]
                          shift-right: [w521] -> _
                          shift-left: w482 -> [w522]
                          shift-right: [w517] -> w483
                          shift-left: w484 -> [w518]
                          i -> [w525]
                          stop <- w526 stop-if-true
                          w516 = T9 12 items=["Floor Length"=48, "Sum of Floors"=12, "Floor Step in ms"=63, "Elevator Door Step in ms"=30, "Global Wait in ms"=20, "Event Wait in ms"=100] ("Elevator Constants")
                          n241 = Increment(x=w523) -> (x+1=w520:i32)
                          n242 = Add(x=w520, y=w525) -> (x+y=w519:i32)
                          n243 = Decrement(x=w519) -> (x-1=w524:i32)
                          n244 = Index Array(array=w530, index=w524) -> (element=w514:bool)
                          n245 = case shown="True" w514 {
                            tunnel: w519 -> [_ w542]
                            tunnel: [w538 w540] -> w521
                            tunnel: w522 -> [w538 w539]
                            frame False {
                            }
                            frame True {
                              n246 = Decrement(x=w542) -> (x-1=w543:i32)
                              n247 = Replace Array Subset(array=w539, new element=FALSE ("new element/subarray"), index=w543) -> (w540:bool[])
                            }
                          }
                          n248 = case shown="True" w514 {
                            tunnel: [w532 w535] -> w517
                            tunnel: w518 -> [w532 w534]
                            tunnel: w519 -> [_ w533]
                            frame False {
                            }
                            frame True {
                              n249 = Decrement(x=w533) -> (x-1=w537:i32)
                              n250 = Replace Array Subset(array=w534, new element=FALSE ("new element/subarray"), index=w537) -> (w535:bool[])
                            }
                          }
                          n251 = To Long Integer(number=w516) -> (32bit integer=w515:i32)
                          n252 = case shown="True" w514 {
                            tunnel: w529 -> [w545 w551]
                            tunnel: w531 -> [w544 w550]
                            tunnel: [w544 w549] -> w528
                            tunnel: [w545 w548] -> w527
                            tunnel: w519 -> [_ w546]
                            frame False {
                            }
                            frame True {
                              n253 = To Unsigned Byte Integer(number=w546) -> (unsigned 8bit integer=w547:u8)
                              n254 = Enqueue Element(queue=w551, element=w547, error in (no error)=w550) -> (queue out=w548:refnum<queue>, error out=w549:errorcluster)  [unwired: 1 in, 1 out]
                            }
                          }
                          n255 = Greater Or Equal?(x=w519, y=w515) -> (x >= y?=w526:bool)
                        }
                        n256 = while {
                          tunnel: w483 -> [w504]
                          shift-right: [w501] -> w490
                          shift-left: w492 -> [w503]
                          shift-right: [w502] -> w489
                          shift-left: w491 -> [w505]
                          tunnel: w485 -> [w494]
                          i -> [w499]
                          stop <- w493 stop-if-true
                          w496 = T9 12 items=["Floor Length"=48, "Sum of Floors"=12, "Floor Step in ms"=63, "Elevator Door Step in ms"=30, "Global Wait in ms"=20, "Event Wait in ms"=100] ("Elevator Constants")
                          n257 = To Long Integer(number=w496) -> (32bit integer=w495:i32)
                          n258 = Subtract(x=w495, y=w499) -> (x-y=w498:i32)
                          n259 = Decrement(x=w498) -> (x-1=w497:i32)
                          n260 = Index Array(array=w504, index=w497) -> (element=w500:bool)
                          n261 = Less Or Equal?(x=w498, y=w494) -> (x <= y?=w493:bool)
                          n262 = case shown="True" w500 {
                            tunnel: w503 -> [w507 w513]
                            tunnel: w505 -> [w506 w512]
                            tunnel: [w506 w511] -> w502
                            tunnel: [w507 w510] -> w501
                            tunnel: w498 -> [_ w509]
                            frame False {
                            }
                            frame True {
                              n263 = To Unsigned Byte Integer(number=w509) -> (unsigned 8bit integer=w508:u8)
                              n264 = Enqueue Element(queue=w513, element=w508, error in (no error)=w512) -> (queue out=w510:refnum<queue>, error out=w511:errorcluster)  [unwired: 1 in, 1 out]
                            }
                          }
                        }
                      }
                      frame False {
                        n265 = while {
                          tunnel: w557 -> [w572]
                          shift-right: [w569] -> w554
                          shift-left: w555 -> [w571]
                          shift-right: [w570] -> w553
                          shift-left: w556 -> [w573]
                          tunnel: w552 -> [w566]
                          i -> [w564]
                          stop <- w567 stop-if-true
                          w559 = T9 12 items=["Floor Length"=48, "Sum of Floors"=12, "Floor Step in ms"=63, "Elevator Door Step in ms"=30, "Global Wait in ms"=20, "Event Wait in ms"=100] ("Elevator Constants")
                          n266 = To Long Integer(number=w559) -> (32bit integer=w558:i32)
                          n267 = Subtract(x=w558, y=w564) -> (x-y=w560:i32)
                          n268 = Decrement(x=w560) -> (x-1=w563:i32)
                          n269 = Index Array(array=w572, index=w563) -> (element=w561:bool)
                          n270 = Index Array(array=w566, index=w563) -> (element=w565:bool)
                          n271 = Or(x=w561, y=w565) -> (x .or. y?=w562:bool)
                          n272 = case shown="True" w562 {
                            tunnel: w571 -> [w575 w581]
                            tunnel: w573 -> [w574 w580]
                            tunnel: [w574 w579] -> w570
                            tunnel: [w575 w578] -> w569
                            tunnel: w560 -> [_ w576]
                            frame False {
                            }
                            frame True {
                              n273 = To Unsigned Byte Integer(number=w576) -> (unsigned 8bit integer=w577:u8)
                              n274 = Enqueue Element(queue=w581, element=w577, error in (no error)=w580) -> (queue out=w578:refnum<queue>, error out=w579:errorcluster)  [unwired: 1 in, 1 out]
                            }
                          }
                          n275 = Less Or Equal?(x=w560, y=1) -> (x <= y?=w567:bool)
                        }
                      }
                    }
                  }
                }
              }
              frame "Going Down" {
                # "Учитываем приоритет: есть ли\nкакой-то этаж, вызванный в кабине, но находящийся выше\nтекущего положения кабины?"
                # "Если был нажат вызов с этажа дома, который уже выбран в кабине то в очередь не добавляем.\nВ отдельных массивах-максках кабины и лифта учитываем, какие этажи уже были добавлены в очередь."
                # "Перебираем вызовы нижних этажей в кабине"
                # "Выстраиваем очеред с приоритетом с учетом направления, вызова из кабины и вызова с этажа (условия написаны в поряжке убывания приоритета)"
                n276 = Flush Queue(queue=w651, error in (no error)=w652) -> (queue out=w650:refnum<queue>, error out=w649:errorcluster)  [unwired: 1 out]
                n277 = while {
                  tunnel: w638 -> [w782]
                  shift-right: [w786] -> w644
                  shift-left: w650 -> [w788]
                  shift-right: [w787] -> w647
                  shift-left: w649 -> [w789]
                  tunnel: w637 -> [w783]
                  shift-right: [w781] -> w641
                  shift-left: w638 -> [w780]
                  shift-right: [w779] -> w640
                  shift-left: w639 -> [w778]
                  tunnel: w639 -> [w775]
                  i -> [w785]
                  stop <- w784 stop-if-true
                  n278 = Subtract(x=w783, y=w785) -> (x-y=w774:i32)
                  n279 = Decrement(x=w774) -> (x-1=w772:i32)
                  n280 = Index Array(array=w775, index=w772) -> (element=w773:bool)
                  n281 = Index Array(array=w782, index=w772) -> (element=w776:bool)
                  n282 = Or(x=w776, y=w773) -> (x .or. y?=w771:bool)
                  n283 = case shown="True" w771 {
                    tunnel: w774 -> [_ w797]
                    tunnel: [w796 w799] -> w781
                    tunnel: w780 -> [w796 w798]
                    frame False {
                    }
                    frame True {
                      n284 = Decrement(x=w797) -> (x-1=w801:i32)
                      n285 = Replace Array Subset(array=w798, new element=FALSE ("new element/subarray"), index=w801) -> (w799:bool[])
                    }
                  }
                  n286 = case shown="True" w771 {
                    tunnel: [w790 w793] -> w779
                    tunnel: w778 -> [w790 w792]
                    tunnel: w774 -> [_ w791]
                    frame False {
                    }
                    frame True {
                      n287 = Decrement(x=w791) -> (x-1=w795:i32)
                      n288 = Replace Array Subset(array=w792, new element=FALSE ("new element/subarray"), index=w795) -> (w793:bool[])
                    }
                  }
                  n289 = case shown="False" w771 {
                    tunnel: w788 -> [w803 w809]
                    tunnel: w789 -> [w802 w808]
                    tunnel: [w802 w807] -> w787
                    tunnel: [w803 w806] -> w786
                    tunnel: w774 -> [_ w804]
                    frame False {
                    }
                    frame True {
                      n290 = To Unsigned Byte Integer(number=w804) -> (unsigned 8bit integer=w805:u8)
                      n291 = Enqueue Element(queue=w809, element=w805, error in (no error)=w808) -> (queue out=w806:refnum<queue>, error out=w807:errorcluster)  [unwired: 1 in, 1 out]
                    }
                  }
                  n292 = Less Or Equal?(x=w774, y=1) -> (x <= y?=w784:bool)
                }
                n293 = while {
                  tunnel: w641 -> [w765]
                  tunnel: [w765] -> w648
                  tunnel: w647 -> [w770]
                  tunnel: [w770] -> w646
                  tunnel: [w769] -> w645
                  tunnel: w644 -> [w769]
                  tunnel: w637 -> [w767]
                  shift-right: [w761] -> _
                  shift-left: 0 -> [w762]
                  tunnel: [w760] -> w642
                  i -> [w766]
                  stop <- w759 stop-if-true
                  w757 = T9 12 items=["Floor Length"=48, "Sum of Floors"=12, "Floor Step in ms"=63, "Elevator Door Step in ms"=30, "Global Wait in ms"=20, "Event Wait in ms"=100] ("Elevator Constants")
                  n294 = Increment(x=w767) -> (x+1=w768:i32)
                  n295 = Add(x=w768, y=w766) -> (x+y=w758:i32)
                  n296 = Decrement(x=w758) -> (x-1=w764:i32)
                  n297 = Index Array(array=w765, index=w764) -> (element=w755:bool)
                  n298 = To Long Integer(number=w757) -> (32bit integer=w756:i32)
                  n299 = Increment(x=w762) -> (x+1=w763:i32)
                  n300 = Select(t=w763, s=w755, f=w762) -> (s? t:f=w761:i32)
                  n301 = Greater Or Equal?(x=w758, y=w756) -> (x >= y?=w759:bool)
                  n302 = Not Equal To 0?(x=w761) -> (x != 0?=w760:bool)
                }
                n303 = case shown="True" w642 {
                  tunnel: [w663 w727] -> w654
                  tunnel: [w662 w726] -> w653
                  tunnel: w641 -> [w655 _]
                  tunnel: w648 -> [w661 w730]
                  tunnel: w646 -> [w660 w729]
                  tunnel: w645 -> [w659 w728]
                  tunnel: w637 -> [w658 _]
                  tunnel: w640 -> [w657 w725]
                  frame True {
                    # "Если есть такой этаж, то добавляем в конец очереди сначала вызовы верхних этажей кабины от меньшего к большему, потом вызовы верхних этажей дома"
                    n304 = while {
                      tunnel: w661 -> [w703]
                      shift-right: [w700] -> w665
                      shift-left: w659 -> [w702]
                      shift-right: [w701] -> w664
                      shift-left: w660 -> [w704]
                      tunnel: w658 -> [w696]
                      shift-right: [w694] -> _
                      shift-left: w655 -> [w695]
                      shift-right: [w690] -> w656
                      shift-left: w657 -> [w691]
                      i -> [w698]
                      stop <- w699 stop-if-true
                      w689 = T9 12 items=["Floor Length"=48, "Sum of Floors"=12, "Floor Step in ms"=63, "Elevator Door Step in ms"=30, "Global Wait in ms"=20, "Event Wait in ms"=100] ("Elevator Constants")
                      n305 = Increment(x=w696) -> (x+1=w693:i32)
                      n306 = Add(x=w693, y=w698) -> (x+y=w692:i32)
                      n307 = Decrement(x=w692) -> (x-1=w697:i32)
                      n308 = Index Array(array=w703, index=w697) -> (element=w687:bool)
                      n309 = case shown="True" w687 {
                        tunnel: w692 -> [_ w715]
                        tunnel: [w711 w713] -> w694
                        tunnel: w695 -> [w711 w712]
                        frame False {
                        }
                        frame True {
                          n310 = Decrement(x=w715) -> (x-1=w716:i32)
                          n311 = Replace Array Subset(array=w712, new element=FALSE ("new element/subarray"), index=w716) -> (w713:bool[])
                        }
                      }
                      n312 = case shown="True" w687 {
                        tunnel: [w705 w708] -> w690
                        tunnel: w691 -> [w705 w707]
                        tunnel: w692 -> [_ w706]
                        frame False {
                        }
                        frame True {
                          n313 = Decrement(x=w706) -> (x-1=w710:i32)
                          n314 = Replace Array Subset(array=w707, new element=FALSE ("new element/subarray"), index=w710) -> (w708:bool[])
                        }
                      }
                      n315 = To Long Integer(number=w689) -> (32bit integer=w688:i32)
                      n316 = case shown="True" w687 {
                        tunnel: w702 -> [w718 w724]
                        tunnel: w704 -> [w717 w723]
                        tunnel: [w717 w722] -> w701
                        tunnel: [w718 w721] -> w700
                        tunnel: w692 -> [_ w719]
                        frame False {
                        }
                        frame True {
                          n317 = To Unsigned Byte Integer(number=w719) -> (unsigned 8bit integer=w720:u8)
                          n318 = Enqueue Element(queue=w724, element=w720, error in (no error)=w723) -> (queue out=w721:refnum<queue>, error out=w722:errorcluster)  [unwired: 1 in, 1 out]
                        }
                      }
                      n319 = Greater Or Equal?(x=w692, y=w688) -> (x >= y?=w699:bool)
                    }
                    n320 = while {
                      tunnel: w656 -> [w677]
                      shift-right: [w674] -> w663
                      shift-left: w665 -> [w676]
                      shift-right: [w675] -> w662
                      shift-left: w664 -> [w678]
                      tunnel: w658 -> [w667]
                      i -> [w672]
                      stop <- w666 stop-if-true
                      w669 = T9 12 items=["Floor Length"=48, "Sum of Floors"=12, "Floor Step in ms"=63, "Elevator Door Step in ms"=30, "Global Wait in ms"=20, "Event Wait in ms"=100] ("Elevator Constants")
                      n321 = To Long Integer(number=w669) -> (32bit integer=w668:i32)
                      n322 = Subtract(x=w668, y=w672) -> (x-y=w671:i32)
                      n323 = Decrement(x=w671) -> (x-1=w670:i32)
                      n324 = Index Array(array=w677, index=w670) -> (element=w673:bool)
                      n325 = Less Or Equal?(x=w671, y=w667) -> (x <= y?=w666:bool)
                      n326 = case shown="True" w673 {
                        tunnel: w676 -> [w680 w686]
                        tunnel: w678 -> [w679 w685]
                        tunnel: [w679 w684] -> w675
                        tunnel: [w680 w683] -> w674
                        tunnel: w671 -> [_ w682]
                        frame False {
                        }
                        frame True {
                          n327 = To Unsigned Byte Integer(number=w682) -> (unsigned 8bit integer=w681:u8)
                          n328 = Enqueue Element(queue=w686, element=w681, error in (no error)=w685) -> (queue out=w683:refnum<queue>, error out=w684:errorcluster)  [unwired: 1 in, 1 out]
                        }
                      }
                    }
                  }
                  frame False {
                    n329 = while {
                      tunnel: w730 -> [w745]
                      shift-right: [w742] -> w727
                      shift-left: w728 -> [w744]
                      shift-right: [w743] -> w726
                      shift-left: w729 -> [w746]
                      tunnel: w725 -> [w739]
                      i -> [w737]
                      stop <- w740 stop-if-true
                      w732 = T9 12 items=["Floor Length"=48, "Sum of Floors"=12, "Floor Step in ms"=63, "Elevator Door Step in ms"=30, "Global Wait in ms"=20, "Event Wait in ms"=100] ("Elevator Constants")
                      n330 = To Long Integer(number=w732) -> (32bit integer=w731:i32)
                      n331 = Subtract(x=w731, y=w737) -> (x-y=w733:i32)
                      n332 = Decrement(x=w733) -> (x-1=w736:i32)
                      n333 = Index Array(array=w745, index=w736) -> (element=w734:bool)
                      n334 = Index Array(array=w739, index=w736) -> (element=w738:bool)
                      n335 = Or(x=w734, y=w738) -> (x .or. y?=w735:bool)
                      n336 = case shown="True" w735 {
                        tunnel: w744 -> [w748 w754]
                        tunnel: w746 -> [w747 w753]
                        tunnel: [w747 w752] -> w743
                        tunnel: [w748 w751] -> w742
                        tunnel: w733 -> [_ w749]
                        frame False {
                        }
                        frame True {
                          n337 = To Unsigned Byte Integer(number=w749) -> (unsigned 8bit integer=w750:u8)
                          n338 = Enqueue Element(queue=w754, element=w750, error in (no error)=w753) -> (queue out=w751:refnum<queue>, error out=w752:errorcluster)  [unwired: 1 in, 1 out]
                        }
                      }
                      n339 = Less Or Equal?(x=w733, y=1) -> (x <= y?=w740:bool)
                    }
                  }
                }
              }
              frame "Going Up" {
                # "Учитываем приоритет: есть ли\nкакой-то этаж, вызванный в кабине, но находящийся ниже\nтекущего положения кабины?"
                # "Если был нажат вызов с этажа, который уже выбран в кабине то в очередь не добавляем.\nВ отдельных массивах-максках кабины и лифта учитываем, какие этажи уже были добавлены в очередь."
                # "Перебираем вызовы верхних этажей в кабине"
                # "Выстраиваем очеред с приоритетом с учетом направления, вызова из кабины и вызова с этажа (условия написаны в поряжке убывания приоритета)"
                n340 = Flush Queue(queue=w827, error in (no error)=w828) -> (queue out=w826:refnum<queue>, error out=w825:errorcluster)  [unwired: 1 out]
                n341 = Increment(x=w811) -> (x+1=w812:i32)
                n342 = while {
                  tunnel: w830 -> [w950]
                  shift-right: [w957] -> w818
                  shift-left: w826 -> [w959]
                  shift-right: [w958] -> w821
                  shift-left: w825 -> [w960]
                  tunnel: w812 -> [w952]
                  shift-right: [w949] -> w823
                  shift-left: w830 -> [w948]
                  shift-right: [w946] -> w824
                  shift-left: w829 -> [w944]
                  shift-right: [w943] -> w810
                  shift-left: w812 -> [w942]
                  i -> [w954]
                  stop <- w953 stop-if-true
                  w951 = T9 12 items=["Floor Length"=48, "Sum of Floors"=12, "Floor Step in ms"=63, "Elevator Door Step in ms"=30, "Global Wait in ms"=20, "Event Wait in ms"=100] ("Elevator Constants")
                  n343 = Add(x=w952, y=w954) -> (x+y=w947:i32)
                  n344 = Decrement(x=w947) -> (x-1=w955:i32)
                  n345 = Index Array(array=w950, index=w955) -> (element=w945:bool)
                  n346 = case shown="True" w945 {
                    tunnel: w947 -> [_ w968]
                    tunnel: [w967 w970] -> w949
                    tunnel: w948 -> [w967 w969]
                    frame False {
                    }
                    frame True {
                      n347 = Decrement(x=w968) -> (x-1=w972:i32)
                      n348 = Replace Array Subset(array=w969, new element=FALSE ("new element/subarray"), index=w972) -> (w970:bool[])
                    }
                  }
                  n349 = case shown="True" w945 {
                    tunnel: [w961 w964] -> w946
                    tunnel: w944 -> [w961 w963]
                    tunnel: w947 -> [_ w962]
                    frame False {
                    }
                    frame True {
                      n350 = Decrement(x=w962) -> (x-1=w966:i32)
                      n351 = Replace Array Subset(array=w963, new element=FALSE ("new element/subarray"), index=w966) -> (w964:bool[])
                    }
                  }
                  n352 = case shown="False" w945 {
                    tunnel: w959 -> [w975 w981]
                    tunnel: w960 -> [w974 w980]
                    tunnel: [w974 w979] -> w958
                    tunnel: [w975 w978] -> w957
                    tunnel: w947 -> [_ w976]
                    tunnel: [w973 w976] -> w943
                    tunnel: w942 -> [w973 _]
                    frame False {
                    }
                    frame True {
                      n353 = To Unsigned Byte Integer(number=w976) -> (unsigned 8bit integer=w977:u8)
                      n354 = Enqueue Element(queue=w981, element=w977, error in (no error)=w980) -> (queue out=w978:refnum<queue>, error out=w979:errorcluster)  [unwired: 1 in, 1 out]
                    }
                  }
                  n355 = To Long Integer(number=w951) -> (32bit integer=w956:i32)
                  n356 = Greater Or Equal?(x=w947, y=w956) -> (x >= y?=w953:bool)
                }
                n357 = while {
                  tunnel: w823 -> [w938]
                  tunnel: [w938] -> w822
                  tunnel: w821 -> [w941]
                  tunnel: [w941] -> w820
                  tunnel: [w940] -> w819
                  tunnel: w818 -> [w940]
                  tunnel: w811 -> [w928]
                  shift-right: [w934] -> _
                  shift-left: 0 -> [w935]
                  tunnel: [w933] -> w816
                  i -> [w939]
                  stop <- w931 stop-if-true
                  n358 = Subtract(x=w928, y=w939) -> (x-y=w930:i32)
                  n359 = Decrement(x=w930) -> (x-1=w937:i32)
                  n360 = Index Array(array=w938, index=w937) -> (element=w929:bool)
                  n361 = Increment(x=w935) -> (x+1=w936:i32)
                  n362 = Less Or Equal?(x=w930, y=1) -> (x <= y?=w931:bool)
                  n363 = Select(t=w936, s=w929, f=w935) -> (s? t:f=w934:i32)
                  n364 = Not Equal To 0?(x=w934) -> (x != 0?=w933:bool)
                }
                n365 = case shown="True" w816 {
                  tunnel: [w842 w899] -> w832
                  tunnel: [w841 w898] -> w831
                  tunnel: w824 -> [w839 w903]
                  tunnel: w822 -> [w838 w902]
                  tunnel: w820 -> [w837 w901]
                  tunnel: w819 -> [w836 w900]
                  tunnel: w810 -> [w835 _]
                  tunnel: [TRUE ("Update Target Floor") TRUE ("Update Target Floor")] -> w813
                  tunnel: w811 -> [w833 _]
                  frame True {
                    # "Перебираем вызовы нижних этажей в кабине и на этажах"
                    # "Добавляем в конец очереди вызовы с верхних этажей, если в кабине есть вызовы на этажи ниже, чем его текущее положение"
                    n366 = while {
                      tunnel: w838 -> [w881]
                      shift-right: [w878] -> w844
                      shift-left: w836 -> [w880]
                      shift-right: [w879] -> w843
                      shift-left: w837 -> [w882]
                      tunnel: w835 -> [w866]
                      tunnel: w839 -> [w875]
                      shift-right: [w869] -> w840
                      shift-left: w839 -> [w870]
                      i -> [w873]
                      stop <- w876 stop-if-true
                      n367 = Subtract(x=w866, y=w873) -> (x-y=w867:i32)
                      n368 = Decrement(x=w867) -> (x-1=w872:i32)
                      n369 = Index Array(array=w881, index=w872) -> (element=w868:bool)
                      n370 = Index Array(array=w875, index=w872) -> (element=w874:bool)
                      n371 = Or(x=w868, y=w874) -> (x .or. y?=w871:bool)
                      n372 = case shown="True" w871 {
                        tunnel: w867 -> [_ w884]
                        tunnel: [w883 w886] -> w869
                        tunnel: w870 -> [w883 w885]
                        frame False {
                        }
                        frame True {
                          n373 = Decrement(x=w884) -> (x-1=w888:i32)
                          n374 = Replace Array Subset(array=w885, new element=FALSE ("new element/subarray"), index=w888) -> (w886:bool[])
                        }
                      }
                      n375 = case shown="True" w871 {
                        tunnel: w880 -> [w890 w896]
                        tunnel: w882 -> [w889 w895]
                        tunnel: [w889 w894] -> w879
                        tunnel: [w890 w893] -> w878
                        tunnel: w867 -> [_ w891]
                        frame False {
                        }
                        frame True {
                          n376 = To Unsigned Byte Integer(number=w891) -> (unsigned 8bit integer=w892:u8)
                          n377 = Enqueue Element(queue=w896, element=w892, error in (no error)=w895) -> (queue out=w893:refnum<queue>, error out=w894:errorcluster)  [unwired: 1 in, 1 out]
                        }
                      }
                      n378 = Less Or Equal?(x=w867, y=1) -> (x <= y?=w876:bool)
                    }
                    n379 = while {
                      tunnel: w840 -> [w856]
                      shift-right: [w853] -> w842
                      shift-left: w844 -> [w855]
                      shift-right: [w854] -> w841
                      shift-left: w843 -> [w857]
                      tunnel: w833 -> [w846]
                      i -> [w851]
                      stop <- w845 stop-if-true
                      w848 = T9 12 items=["Floor Length"=48, "Sum of Floors"=12, "Floor Step in ms"=63, "Elevator Door Step in ms"=30, "Global Wait in ms"=20, "Event Wait in ms"=100] ("Elevator Constants")
                      n380 = To Long Integer(number=w848) -> (32bit integer=w847:i32)
                      n381 = Subtract(x=w847, y=w851) -> (x-y=w850:i32)
                      n382 = Decrement(x=w850) -> (x-1=w849:i32)
                      n383 = Index Array(array=w856, index=w849) -> (element=w852:bool)
                      n384 = Less Or Equal?(x=w850, y=w846) -> (x <= y?=w845:bool)
                      n385 = case shown="True" w852 {
                        tunnel: w855 -> [w859 w865]
                        tunnel: w857 -> [w858 w864]
                        tunnel: [w858 w863] -> w854
                        tunnel: [w859 w862] -> w853
                        tunnel: w850 -> [_ w861]
                        frame False {
                        }
                        frame True {
                          n386 = To Unsigned Byte Integer(number=w861) -> (unsigned 8bit integer=w860:u8)
                          n387 = Enqueue Element(queue=w865, element=w860, error in (no error)=w864) -> (queue out=w862:refnum<queue>, error out=w863:errorcluster)  [unwired: 1 in, 1 out]
                        }
                      }
                    }
                  }
                  frame False {
                    # "Перебираем вызовы  на этажах"
                    n388 = while {
                      tunnel: w902 -> [w918]
                      shift-right: [w915] -> w899
                      shift-left: w900 -> [w917]
                      shift-right: [w916] -> w898
                      shift-left: w901 -> [w919]
                      tunnel: w903 -> [w912]
                      i -> [w910]
                      stop <- w913 stop-if-true
                      w905 = T9 12 items=["Floor Length"=48, "Sum of Floors"=12, "Floor Step in ms"=63, "Elevator Door Step in ms"=30, "Global Wait in ms"=20, "Event Wait in ms"=100] ("Elevator Constants")
                      n389 = To Long Integer(number=w905) -> (32bit integer=w904:i32)
                      n390 = Subtract(x=w904, y=w910) -> (x-y=w906:i32)
                      n391 = Decrement(x=w906) -> (x-1=w909:i32)
                      n392 = Index Array(array=w918, index=w909) -> (element=w907:bool)
                      n393 = Index Array(array=w912, index=w909) -> (element=w911:bool)
                      n394 = Or(x=w907, y=w911) -> (x .or. y?=w908:bool)
                      n395 = case shown="True" w908 {
                        tunnel: w917 -> [w921 w927]
                        tunnel: w919 -> [w920 w926]
                        tunnel: [w920 w925] -> w916
                        tunnel: [w921 w924] -> w915
                        tunnel: w906 -> [_ w922]
                        frame False {
                        }
                        frame True {
                          n396 = To Unsigned Byte Integer(number=w922) -> (unsigned 8bit integer=w923:u8)
                          n397 = Enqueue Element(queue=w927, element=w923, error in (no error)=w926) -> (queue out=w924:refnum<queue>, error out=w925:errorcluster)  [unwired: 1 in, 1 out]
                        }
                      }
                      n398 = Less Or Equal?(x=w906, y=1) -> (x <= y?=w913:bool)
                    }
                  }
                }
                n399 = local read "Elevator Automate"() -> (w815:T2)
                n400 = Bundle By Name(cluster=w815, "Update Target Floor"=w813) -> (w814:T2)
                n401 = local write "Elevator Automate"(w814) -> ()
              }
            }
          }
        }
      }
    }
    n402 = local read "milliseconds to wait"() -> (w22:u32)
    n403 = Wait (ms)(milliseconds to wait=w22) -> ()  [unwired: 1 out]
    n404 = local read "STOP"() -> (w43:bool)
    n405 = call <vilib>:"Release Semaphore.vi"("error in (no error)"=w25, "semaphore"=w26) -> ("error out"=w23:errorcluster, "semaphore out"=w24:T8)  [unwired: 4 in]
  }
  n406 = flat-sequence {
    tunnel: ["Floors Schematic"] -> w11
    tunnel: ["Elevator Panel"] -> w10
    tunnel: [w1066] -> w9
    tunnel: [w1065] -> w8
    tunnel: [w1062] -> w13
    tunnel: [w1069] -> w2
    tunnel: [w1068] -> w1
    tunnel: [w1052] -> w4
    tunnel: [w1051] -> w3
    frame #0 {
      w1059 = T9 12 items=["Floor Length"=48, "Sum of Floors"=12, "Floor Step in ms"=63, "Elevator Door Step in ms"=30, "Global Wait in ms"=20, "Event Wait in ms"=100] ("Elevator Constants")
      w1061 = T9 12 items=["Floor Length"=48, "Sum of Floors"=12, "Floor Step in ms"=63, "Elevator Door Step in ms"=30, "Global Wait in ms"=20, "Event Wait in ms"=100] ("Elevator Constants")
      w1056 = FALSE ("GoTo Idle")
      n407 = stacked-sequence {
        tunnel: [w1242 _] -> w1081
        frame #0 {
          n408 = control-ref of="Call 1"() -> (w1237:refnum<vi>)
          n409 = property class="Bool (strict)"(reference=w1237) -> ("Left"=w1239:i32, "Top"=w1241:i32)  [unwired: 1 in, 2 out]
          n410 = control-ref of="Elevator Cabin"() -> (w1243:refnum<vi>)
          n411 = Add(x=w1241, y=1) -> (x+y=w1236:i32)
          n412 = Add(x=w1239, y=100) -> (x+y=w1235:i32)
          n413 = property class="Slide (strict)"(reference=w1243, "Left"=w1235, "Top"=w1236) -> (reference out=w1242:refnum<vi>)  [unwired: 1 in, 1 out]
        }
        frame #1 {
          n414 = local write "Elevator Cabin"(T5 100 ("Elevator Cabin")) -> ()
        }
      }
      n415 = property class="Slide (strict)"(reference=w1081) -> ("Top"=w1080:i32)  [unwired: 1 in, 2 out]
      n416 = Unbundle By Name("Floors Schematic") -> ("Floor Position"=w1098:i16[])
      n417 = Bundle(cluster="Floors Schematic", "Call 1"=FALSE, "Call 2"=FALSE, "Call 3"=FALSE, "Call 4"=FALSE, "Call 5"=FALSE, "Call 6"=FALSE, "Call 7"=FALSE, "Call 8"=FALSE, "Call 9"=FALSE, "Call 10"=FALSE, "Call 11"=FALSE, "Call 12"=FALSE) -> (w1070:T4)  [unwired: 1 in]
      n418 = local write "Floors Schematic"(w1070) -> ()
      n419 = To Long Integer(number=w1059) -> (32bit integer=w1058:i32)
      n420 = for {
        N: w1058 -> [_]
        shift-right: [w1252] -> _
        shift-left: w1080 -> [w1247]
        shift-right: [w1249] -> _
        shift-left: w1098 -> [w1251]
        i -> [w1254]
        w1245 = T9 48 items=["Floor Length"=48, "Sum of Floors"=12, "Milliseconds Per Step"=63] ("Elevator Constants")
        n421 = To Long Integer(number=w1245) -> (32bit integer=w1246:i32)
        n422 = To Word Integer(number=w1247) -> (16bit integer=w1253:i16)
        n423 = Replace Array Subset(array=w1251, new element=w1253, index=w1254) -> (w1249:i16[])
        n424 = Subtract(x=w1247, y=w1246) -> (x-y=w1252:i32)
        n425 = local read "Floors Schematic"() -> (w1250:T4)
        n426 = Bundle By Name(cluster=w1250, "Floor Position"=w1249) -> (w1248:T4)
        n427 = local write "Floors Schematic"(w1248) -> ()
      }
      n428 = Bundle(cluster="Elevator Panel", "Open Doors"=FALSE, "Close Doors"=FALSE, "Floor 2"=FALSE, "Floor 1"=FALSE, "Floor 3"=FALSE, "Floor 4"=FALSE, "Floor 5"=FALSE, "Floor 6"=FALSE, "Floor 7"=FALSE, "Floor 8"=FALSE, "Floor 9"=FALSE, "Floor 10"=FALSE, "Floor 11"=FALSE, "Floor 12"=FALSE, "Emergency"=FALSE, "Cancel"=FALSE) -> (w1055:T3)
      n429 = local write "STOP"(FALSE ("STOP")) -> ()
      n430 = Bundle By Name(cluster=w1055, "Passanger Window"="") -> (w1053:T3)
      n431 = To Unsigned Byte Integer(number=1) -> (unsigned 8bit integer=w1064:u8)
      n432 = Obtain Queue(name (unnamed)="Elevator Floor Queue", element data type=w1064) -> (queue out=w1069:refnum<queue>, error out=w1068:errorcluster)  [unwired: 3 in, 1 out]
      n433 = local write "Elevator Panel"(w1053) -> ()
      n434 = Bundle(cluster="Elevator Automate", "Elevator Panel Array"=bool[] [FALSE, FALSE, FALSE, FALSE, FALSE, FALSE, FALSE, FALSE, FALSE, FALSE, FALSE, FALSE], "Floor Array"=bool[] [FALSE, FALSE, FALSE, FALSE, FALSE, FALSE, FALSE, FALSE, FALSE, FALSE, FALSE, FALSE], "Elevator Command"=Elevator_Command."Idle", "Target Floor"=u8 1, "Forced Stop"=w1056, "Cancel Delay"=w1056, "Elevator Status"=w1056, "Update\nTarget Floor"=T10."Stand By" ("Elevator Status"), "Take a Call"=w1056, "Add Floor\nto Queue"=w1056) -> (w1062:T2)
      n435 = To Long Integer(number=w1061) -> (32bit integer=w1060:i32)
      n436 = for {
        N: w1060 -> [_]
        i -> [w1114]
        n437 = Increment(x=w1114) -> (x+1=w1113:i32)
        n438 = case shown="8" w1113 {
          frame 1, Default {
            n439 = local read "Floors Schematic"() -> (w1177:T4)
            n440 = Bundle By Name(cluster=w1177, "Call 1"=FALSE ("Call 12")) -> (w1175:T4)
            n441 = control-ref of="Call 1"() -> (w1179:refnum<vi>)
            n442 = local write "Floors Schematic"(w1175) -> ()
            n443 = property class="Bool (strict)"(reference=w1179, "DisabledEnum"=T7."Enabled" ("Disabled")) -> ()  [unwired: 1 in, 2 out]
          }
          frame 2 {
            n444 = local read "Floors Schematic"() -> (w1182:T4)
            n445 = Bundle By Name(cluster=w1182, "Call 2"=FALSE ("Call 12")) -> (w1180:T4)
            n446 = control-ref of="Call 2"() -> (w1184:refnum<vi>)
            n447 = local write "Floors Schematic"(w1180) -> ()
            n448 = property class="Bool (strict)"(reference=w1184, "DisabledEnum"=T7."Enabled" ("Disabled")) -> ()  [unwired: 1 in, 2 out]
          }
          frame 3 {
            n449 = local read "Floors Schematic"() -> (w1187:T4)
            n450 = Bundle By Name(cluster=w1187, "Call 3"=FALSE ("Call 12")) -> (w1185:T4)
            n451 = control-ref of="Call 3"() -> (w1189:refnum<vi>)
            n452 = local write "Floors Schematic"(w1185) -> ()
            n453 = property class="Bool (strict)"(reference=w1189, "DisabledEnum"=T7."Enabled" ("Disabled")) -> ()  [unwired: 1 in, 2 out]
          }
          frame 4 {
            n454 = local read "Floors Schematic"() -> (w1192:T4)
            n455 = Bundle By Name(cluster=w1192, "Call 4"=FALSE ("Call 12")) -> (w1190:T4)
            n456 = control-ref of="Call 4"() -> (w1194:refnum<vi>)
            n457 = local write "Floors Schematic"(w1190) -> ()
            n458 = property class="Bool (strict)"(reference=w1194, "DisabledEnum"=T7."Enabled" ("Disabled")) -> ()  [unwired: 1 in, 2 out]
          }
          frame 5 {
            n459 = local read "Floors Schematic"() -> (w1197:T4)
            n460 = Bundle By Name(cluster=w1197, "Call 5"=FALSE ("Call 12")) -> (w1195:T4)
            n461 = control-ref of="Call 5"() -> (w1199:refnum<vi>)
            n462 = local write "Floors Schematic"(w1195) -> ()
            n463 = property class="Bool (strict)"(reference=w1199, "DisabledEnum"=T7."Enabled" ("Disabled")) -> ()  [unwired: 1 in, 2 out]
          }
          frame 6 {
            n464 = local read "Floors Schematic"() -> (w1202:T4)
            n465 = Bundle By Name(cluster=w1202, "Call 6"=FALSE ("Call 12")) -> (w1200:T4)
            n466 = control-ref of="Call 6"() -> (w1204:refnum<vi>)
            n467 = local write "Floors Schematic"(w1200) -> ()
            n468 = property class="Bool (strict)"(reference=w1204, "DisabledEnum"=T7."Enabled" ("Disabled")) -> ()  [unwired: 1 in, 2 out]
          }
          frame 7 {
            n469 = local read "Floors Schematic"() -> (w1207:T4)
            n470 = Bundle By Name(cluster=w1207, "Call 7"=FALSE ("Call 12")) -> (w1205:T4)
            n471 = control-ref of="Call 7"() -> (w1209:refnum<vi>)
            n472 = local write "Floors Schematic"(w1205) -> ()
            n473 = property class="Bool (strict)"(reference=w1209, "DisabledEnum"=T7."Enabled" ("Disabled")) -> ()  [unwired: 1 in, 2 out]
          }
          frame 8 {
            n474 = local read "Floors Schematic"() -> (w1212:T4)
            n475 = Bundle By Name(cluster=w1212, "Call 8"=FALSE ("Call 12")) -> (w1210:T4)
            n476 = control-ref of="Call 8"() -> (w1214:refnum<vi>)
            n477 = local write "Floors Schematic"(w1210) -> ()
            n478 = property class="Bool (strict)"(reference=w1214, "DisabledEnum"=T7."Enabled" ("Disabled")) -> ()  [unwired: 1 in, 2 out]
          }
          frame 9 {
            n479 = local read "Floors Schematic"() -> (w1217:T4)
            n480 = Bundle By Name(cluster=w1217, "Call 9"=FALSE ("Call 12")) -> (w1215:T4)
            n481 = control-ref of="Call 9"() -> (w1219:refnum<vi>)
            n482 = local write "Floors Schematic"(w1215) -> ()
            n483 = property class="Bool (strict)"(reference=w1219, "DisabledEnum"=T7."Enabled" ("Disabled")) -> ()  [unwired: 1 in, 2 out]
          }
          frame 10 {
            n484 = local read "Floors Schematic"() -> (w1222:T4)
            n485 = Bundle By Name(cluster=w1222, "Call 10"=FALSE ("Call 12")) -> (w1220:T4)
            n486 = control-ref of="Call 10"() -> (w1224:refnum<vi>)
            n487 = local write "Floors Schematic"(w1220) -> ()
            n488 = property class="Bool (strict)"(reference=w1224, "DisabledEnum"=T7."Enabled" ("Disabled")) -> ()  [unwired: 1 in, 2 out]
          }
          frame 11 {
            n489 = local read "Floors Schematic"() -> (w1227:T4)
            n490 = Bundle By Name(cluster=w1227, "Call 11"=FALSE ("Call 12")) -> (w1225:T4)
            n491 = control-ref of="Call 11"() -> (w1229:refnum<vi>)
            n492 = local write "Floors Schematic"(w1225) -> ()
            n493 = property class="Bool (strict)"(reference=w1229, "DisabledEnum"=T7."Enabled" ("Disabled")) -> ()  [unwired: 1 in, 2 out]
          }
          frame 12 {
            n494 = local read "Floors Schematic"() -> (w1232:T4)
            n495 = Bundle By Name(cluster=w1232, "Call 12"=FALSE) -> (w1230:T4)
            n496 = control-ref of="Call 12"() -> (w1234:refnum<vi>)
            n497 = local write "Floors Schematic"(w1230) -> ()
            n498 = property class="Bool (strict)"(reference=w1234, "DisabledEnum"=T7."Enabled" ("Disabled")) -> ()  [unwired: 1 in, 2 out]
          }
        }
        n499 = case shown="8" w1113 {
          frame 1, Default {
            n500 = local read "Elevator Panel"() -> (w1117:T3)
            n501 = Bundle By Name(cluster=w1117, "Floor 1"=FALSE ("Call 12")) -> (w1115:T3)
            n502 = control-ref of="Floor 1"() -> (w1119:refnum<vi>)
            n503 = local write "Elevator Panel"(w1115) -> ()
            n504 = property class="Bool (strict)"(reference=w1119, "DisabledEnum"=T7."Enabled" ("Disabled")) -> ()  [unwired: 1 in, 2 out]
          }
          frame 2 {
            n505 = local read "Elevator Panel"() -> (w1122:T3)
            n506 = Bundle By Name(cluster=w1122, "Floor 2"=FALSE ("Call 12")) -> (w1120:T3)
            n507 = control-ref of="Floor 2"() -> (w1124:refnum<vi>)
            n508 = local write "Elevator Panel"(w1120) -> ()
            n509 = property class="Bool (strict)"(reference=w1124, "DisabledEnum"=T7."Enabled" ("Disabled")) -> ()  [unwired: 1 in, 2 out]
          }
          frame 3 {
            n510 = local read "Elevator Panel"() -> (w1127:T3)
            n511 = Bundle By Name(cluster=w1127, "Floor 3"=FALSE ("Call 12")) -> (w1125:T3)
            n512 = control-ref of="Floor 3"() -> (w1129:refnum<vi>)
            n513 = local write "Elevator Panel"(w1125) -> ()
            n514 = property class="Bool (strict)"(reference=w1129, "DisabledEnum"=T7."Enabled" ("Disabled")) -> ()  [unwired: 1 in, 2 out]
          }
          frame 4 {
            n515 = local read "Elevator Panel"() -> (w1132:T3)
            n516 = Bundle By Name(cluster=w1132, "Floor 4"=FALSE ("Call 12")) -> (w1130:T3)
            n517 = control-ref of="Floor 4"() -> (w1134:refnum<vi>)
            n518 = local write "Elevator Panel"(w1130) -> ()
            n519 = property class="Bool (strict)"(reference=w1134, "DisabledEnum"=T7."Enabled" ("Disabled")) -> ()  [unwired: 1 in, 2 out]
          }
          frame 5 {
            n520 = local read "Elevator Panel"() -> (w1137:T3)
            n521 = Bundle By Name(cluster=w1137, "Floor 5"=FALSE ("Call 12")) -> (w1135:T3)
            n522 = control-ref of="Floor 5"() -> (w1139:refnum<vi>)
            n523 = local write "Elevator Panel"(w1135) -> ()
            n524 = property class="Bool (strict)"(reference=w1139, "DisabledEnum"=T7."Enabled" ("Disabled")) -> ()  [unwired: 1 in, 2 out]
          }
          frame 6 {
            n525 = local read "Elevator Panel"() -> (w1142:T3)
            n526 = Bundle By Name(cluster=w1142, "Floor 6"=FALSE ("Call 12")) -> (w1140:T3)
            n527 = control-ref of="Floor 6"() -> (w1144:refnum<vi>)
            n528 = local write "Elevator Panel"(w1140) -> ()
            n529 = property class="Bool (strict)"(reference=w1144, "DisabledEnum"=T7."Enabled" ("Disabled")) -> ()  [unwired: 1 in, 2 out]
          }
          frame 7 {
            n530 = local read "Elevator Panel"() -> (w1147:T3)
            n531 = Bundle By Name(cluster=w1147, "Floor 7"=FALSE ("Call 12")) -> (w1145:T3)
            n532 = control-ref of="Floor 7"() -> (w1149:refnum<vi>)
            n533 = local write "Elevator Panel"(w1145) -> ()
            n534 = property class="Bool (strict)"(reference=w1149, "DisabledEnum"=T7."Enabled" ("Disabled")) -> ()  [unwired: 1 in, 2 out]
          }
          frame 8 {
            n535 = local read "Elevator Panel"() -> (w1152:T3)
            n536 = Bundle By Name(cluster=w1152, "Floor 8"=FALSE ("Call 12")) -> (w1150:T3)
            n537 = control-ref of="Floor 8"() -> (w1154:refnum<vi>)
            n538 = local write "Elevator Panel"(w1150) -> ()
            n539 = property class="Bool (strict)"(reference=w1154, "DisabledEnum"=T7."Enabled" ("Disabled")) -> ()  [unwired: 1 in, 2 out]
          }
          frame 9 {
            n540 = local read "Elevator Panel"() -> (w1157:T3)
            n541 = Bundle By Name(cluster=w1157, "Floor 9"=FALSE ("Call 12")) -> (w1155:T3)
            n542 = control-ref of="Floor 9"() -> (w1159:refnum<vi>)
            n543 = local write "Elevator Panel"(w1155) -> ()
            n544 = property class="Bool (strict)"(reference=w1159, "DisabledEnum"=T7."Enabled" ("Disabled")) -> ()  [unwired: 1 in, 2 out]
          }
          frame 10 {
            n545 = local read "Elevator Panel"() -> (w1162:T3)
            n546 = Bundle By Name(cluster=w1162, "Floor 10"=FALSE ("Call 12")) -> (w1160:T3)
            n547 = control-ref of="Floor 10"() -> (w1164:refnum<vi>)
            n548 = local write "Elevator Panel"(w1160) -> ()
            n549 = property class="Bool (strict)"(reference=w1164, "DisabledEnum"=T7."Enabled" ("Disabled")) -> ()  [unwired: 1 in, 2 out]
          }
          frame 11 {
            n550 = local read "Elevator Panel"() -> (w1167:T3)
            n551 = Bundle By Name(cluster=w1167, "Floor 11"=FALSE ("Call 12")) -> (w1165:T3)
            n552 = control-ref of="Floor 11"() -> (w1169:refnum<vi>)
            n553 = local write "Elevator Panel"(w1165) -> ()
            n554 = property class="Bool (strict)"(reference=w1169, "DisabledEnum"=T7."Enabled" ("Disabled")) -> ()  [unwired: 1 in, 2 out]
          }
          frame 12 {
            n555 = local read "Elevator Panel"() -> (w1172:T3)
            n556 = Bundle By Name(cluster=w1172, "Floor 12"=FALSE ("Call 12")) -> (w1171:T3)
            n557 = control-ref of="Floor 12"() -> (w1174:refnum<vi>)
            n558 = local write "Elevator Panel"(w1171) -> ()
            n559 = property class="Bool (strict)"(reference=w1174, "DisabledEnum"=T7."Enabled" ("Disabled")) -> ()  [unwired: 1 in, 2 out]
          }
        }
      }
      n560 = Unbundle By Name(w1062) -> ("Elevator Command"=w1074:T1)
      n561 = local write "Elevator Automate"(w1062) -> ()
      n562 = Obtain Queue(name (unnamed)="Elevator Command Queue", element data type=w1074) -> (queue out=w1066:refnum<queue>, error out=w1065:errorcluster)  [unwired: 3 in, 1 out]
      n563 = call <vilib>:"Obtain Semaphore Reference.vi"("size (1)"=1, "name (unnamed)"="Global Elevator Semaphore") -> ("error out"=w1051:errorcluster, "semaphore"=w1052:T8)  [unwired: 3 in, 1 out]
      "Elevator Cabin" <- T5 100 ("Elevator Cabin")
    }
  }
  n564 = disable-structure shown="Enabled" {
    disable-tunnel: w11 -> [w1259 _]
    disable-tunnel: w10 -> [w1258 _]
    disable-tunnel: w4 -> [w1257 _]
    disable-tunnel: w3 -> [w1256 _]
    frame Disabled {
      n565 = while {
        tunnel: w1259 -> [_]
        tunnel: w1258 -> [_]
        shift-right: [w1270] -> _
        shift-left: TRUE -> [w1269]
        tunnel: w1257 -> [w1268]
        tunnel: w1256 -> [w1267]
        tunnel: [w1266] -> _
        tunnel: [w1265] -> _
        stop <- w1271 stop-if-true
        n566 = call <vilib>:"Acquire Semaphore.vi"("error in (no error)"=w1267, "semaphore"=w1268) -> ("error out"=w1262:errorcluster, "semaphore out"=w1264:T8)  [unwired: 3 in, 1 out]
        n567 = flat-sequence {
          tunnel: [w1295] -> w1270
          tunnel: w1269 -> [w1294]
          tunnel: w1264 -> [w1275]
          tunnel: [w1275] -> w1263
          tunnel: w1262 -> [w1274]
          tunnel: [w1274] -> w1261
          frame #0 {
            # "Если лифт между этажами едет наверх,\nприравниваем позицию лифта к этажу, что ниже текущего положения.\nЕсли лифт едет между этажами вниз, то приравниваем позицию лифта к этажу, что выше текущего положения"
            # "Информационное табло лифта для пассажиров"
            n568 = local read "Elevator Automate"() -> (w1284:T2)
            n569 = Unbundle By Name(w1284) -> ("Elevator Status"=w1282:T6)
            n570 = local read "Elevator Panel"() -> (w1288:T3)
            n571 = Equal?(x=w1282, y=T10."Going Up") -> (x = y?=w1276:bool)
            n572 = Unbundle By Name(w1288) -> ("Emergency"=w1287:bool)
            n573 = case shown="True" w1287 {
              tunnel: ["" ("string") w1339] -> w1289
              frame False {
                (unwired) "\r\n"
              }
              frame True {
                n574 = Concatenate Strings("\r\n", "Вызов оператора\nГоворите в микрофон" ("string")) -> (w1339:string)
              }
            }
            n575 = Equal?(x=w1282, y=T10."Stand By") -> (x = y?=w1279:bool)
            n576 = Equal?(x=w1282, y=T10."Stop") -> (x = y?=w1278:bool)
            n577 = Or(x=w1279, y=w1278) -> (x .or. y?=w1277:bool)
            n578 = case shown="False" w1277 {
              tunnel: w1276 -> [w1296 _]
              tunnel: [w1296 w1297] -> w1295
              tunnel: w1294 -> [_ w1297]
              frame False {
              }
              frame True {
              }
            }
            n579 = case shown="False" w1295 {
              tunnel: [w1298 w1320] -> w1285
              frame False {
                n580 = local read "Floors Schematic"() -> (w1301:T4)
                n581 = control-ref of="Elevator Cabin"() -> (w1302:refnum<vi>)
                n582 = property class="Slide (strict)"(reference=w1302) -> ("Top"=w1299:i32)  [unwired: 1 in, 2 out]
                n583 = Unbundle By Name(w1301) -> ("Floor Position"=w1300:i16[])
                n584 = while {
                  tunnel: w1300 -> [w1312]
                  tunnel: w1299 -> [w1310]
                  tunnel: [w1309] -> w1298
                  i -> [w1307]
                  stop <- w1308 stop-if-true
                  w1305 = T9 12 items=["Floor Length"=48, "Sum of Floors"=12, "Floor Step in ms"=63, "Elevator Door Step in ms"=30, "Global Wait in ms"=20, "Event Wait in ms"=100] ("Elevator Constants")
                  n585 = To Long Integer(number=w1305) -> (32bit integer=w1306:i32)
                  n586 = Subtract(x=w1306, y=w1307) -> (x-y=w1304:i32)
                  n587 = Decrement(x=w1304) -> (x-1=w1303:i32)
                  n588 = Index Array(array=w1312, index=w1303) -> (element=w1313:i16)
                  n589 = To Long Integer(number=w1313) -> (32bit integer=w1311:i32)
                  n590 = Equal?(x=w1310, y=w1311) -> (x = y?=w1314:bool)
                  n591 = Greater Or Equal?(x=w1311, y=w1310) -> (x >= y?=w1308:bool)
                  n592 = case shown="False" w1314 {
                    tunnel: w1303 -> [w1317 w1319]
                    tunnel: [w1315 w1318] -> w1309
                    frame False {
                      n593 = Increment(x=w1317) -> (x+1=w1316:i32)
                      n594 = Increment(x=w1316) -> (x+1=w1315:i32)
                    }
                    frame True {
                      n595 = Increment(x=w1319) -> (x+1=w1318:i32)
                    }
                  }
                }
              }
              frame True {
                n596 = local read "Floors Schematic"() -> (w1323:T4)
                n597 = control-ref of="Elevator Cabin"() -> (w1324:refnum<vi>)
                n598 = property class="Slide (strict)"(reference=w1324) -> ("Top"=w1321:i32)  [unwired: 1 in, 2 out]
                n599 = Unbundle By Name(w1323) -> ("Floor Position"=w1322:i16[])
                n600 = while {
                  tunnel: w1322 -> [w1330]
                  tunnel: w1321 -> [w1328]
                  tunnel: [w1327] -> w1320
                  i -> [w1325]
                  stop <- w1326 stop-if-true
                  n601 = Index Array(array=w1330, index=w1325) -> (element=w1331:i16)
                  n602 = To Long Integer(number=w1331) -> (32bit integer=w1329:i32)
                  n603 = Equal?(x=w1328, y=w1329) -> (x = y?=w1332:bool)
                  n604 = Less Or Equal?(x=w1329, y=w1328) -> (x <= y?=w1326:bool)
                  n605 = case shown="False" w1332 {
                    tunnel: w1325 -> [w1333 w1335]
                    tunnel: [w1333 w1334] -> w1327
                    frame False {
                    }
                    frame True {
                      n606 = Increment(x=w1335) -> (x+1=w1334:i32)
                    }
                  }
                }
              }
            }
            n607 = Number To Decimal String(number=w1285) -> (decimal integer string=w1290:string)  [unwired: 1 in]
            n608 = control-ref of="Elevator Cabin"() -> (w1273:refnum<vi>)
            n609 = Concatenate Strings("Этаж " ("string"), w1290, w1289) -> (w1291:string)
            n610 = property class="Slide (strict)"(reference=w1273) -> ("Top"=→"Position:Top":i32)  [unwired: 1 in, 2 out]
            n611 = local read "Elevator Panel"() -> (w1293:T3)
            n612 = Bundle By Name(cluster=w1293, "Passanger Window"=w1291) -> (w1292:T3)
            n613 = local write "Elevator Panel"(w1292) -> ()
          }
        }
        n614 = local read "milliseconds to wait"() -> (w1260:u32)
        n615 = Wait (ms)(milliseconds to wait=w1260) -> ()  [unwired: 1 out]
        n616 = local read "STOP"() -> (w1271:bool)
        n617 = call <vilib>:"Release Semaphore.vi"("error in (no error)"=w1261, "semaphore"=w1263) -> ("error out"=w1265:errorcluster, "semaphore out"=w1266:T8)  [unwired: 4 in]
      }
    }
    frame Enabled {
    }
  }
  n618 = disable-structure shown="Enabled" {
    disable-tunnel: w11 -> [w1345 _]
    disable-tunnel: w10 -> [w1344 _]
    disable-tunnel: w2 -> [w1343 _]
    disable-tunnel: w1 -> [w1342 _]
    disable-tunnel: w4 -> [w1341 _]
    disable-tunnel: w3 -> [w1340 _]
    frame Disabled {
      n619 = while {
        shift-right: [w1363] -> _
        shift-left: w1343 -> [w1352]
        shift-right: [w1362] -> _
        shift-left: w1342 -> [w1351]
        tunnel: w1345 -> [_]
        tunnel: w1344 -> [_]
        tunnel: w1341 -> [w1356]
        tunnel: w1340 -> [w1355]
        tunnel: [w1348] -> _
        tunnel: [w1347] -> _
        stop <- w1364 stop-if-true
        # "Передача номера первого в очереди\nэтажа в номер этажа, на который нужно приехать\nв текущий момент времени"
        n620 = call <vilib>:"Acquire Semaphore.vi"("error in (no error)"=w1355, "semaphore"=w1356) -> ("error out"=w1353:errorcluster, "semaphore out"=w1354:T8)  [unwired: 3 in, 1 out]
        n621 = local read "milliseconds to wait"() -> (w1346:u32)
        n622 = flat-sequence {
          tunnel: [w1366] -> w1361
          tunnel: [w1365] -> w1360
          tunnel: [w1371] -> w1359
          tunnel: [w1369] -> w1358
          tunnel: [w1370] -> w1357
          tunnel: w1354 -> [w1370]
          tunnel: w1353 -> [w1369]
          tunnel: w1352 -> [w1368]
          tunnel: w1351 -> [w1367]
          tunnel: [w1381] -> w1363
          tunnel: [w1380] -> w1362
          tunnel: w1361 -> [w1388]
          tunnel: w1360 -> [w1387]
          tunnel: w1359 -> [w1386]
          tunnel: w1358 -> [w1385]
          tunnel: w1357 -> [w1384]
          tunnel: [w1383] -> w1350
          tunnel: [w1382] -> w1349
          frame #0 {
            n623 = local read "Elevator Automate"() -> (w1377:T2)
            n624 = Unbundle By Name(w1377) -> ("Elevator Command"=w1379:T1)
            n625 = To Long Integer(number=1) -> (32bit integer=w1374:i32)
            n626 = Preview Queue Element(queue=w1368, timeout in ms (-1)=w1374, error in (no error)=w1367) -> (queue out=w1366:refnum<queue>, timed out?=w1375:bool, error out=w1365:errorcluster)  [unwired: 1 out]
            n627 = Not(x=w1375) -> (.not. x?=w1376:bool)
            n628 = Equal?(x=w1379, y=Elevator_Command."Idle" ("element")) -> (x = y?=w1378:bool)
            n629 = And(x=w1378, y=w1376) -> (x .and. y?=w1371:bool)
          }
          frame #1 {
            n630 = case shown="True" w1386 {
              tunnel: w1388 -> [w1392 w1400]
              tunnel: w1387 -> [w1391 w1399]
              tunnel: [w1392 w1400] -> w1381
              tunnel: [w1391 w1399] -> w1380
              tunnel: w1385 -> [w1389 w1396]
              tunnel: w1384 -> [w1390 w1395]
              tunnel: [w1390 w1394] -> w1383
              tunnel: [w1389 w1393] -> w1382
              frame False {
              }
              frame True {
                n631 = flat-sequence {
                  tunnel: [w1402] -> w1398
                  tunnel: [w1401] -> w1397
                  tunnel: w1395 -> [w1402]
                  tunnel: w1396 -> [w1401]
                  tunnel: w1398 -> [w1408]
                  tunnel: w1397 -> [w1407]
                  tunnel: [w1408] -> w1394
                  tunnel: [w1407] -> w1393
                  frame #0 {
                    n632 = local read "Elevator Automate"() -> (w1405:T2)
                    n633 = Bundle By Name(cluster=w1405, "Update Target Floor"=TRUE) -> (w1404:T2)
                    n634 = local write "Elevator Automate"(w1404) -> ()
                    n635 = Wait (ms)(milliseconds to wait=u32 1) -> ()  [unwired: 1 out]
                  }
                  frame #1 {
                    n636 = local read "Elevator Automate"() -> (w1412:T2)
                    n637 = Bundle By Name(cluster=w1412, "Take a Call"=TRUE ("Update Target Floor")) -> (w1411:T2)
                    n638 = local write "Elevator Automate"(w1411) -> ()
                    n639 = Wait (ms)(milliseconds to wait=u32 1) -> ()  [unwired: 1 out]
                  }
                }
              }
            }
          }
        }
        n640 = Wait (ms)(milliseconds to wait=w1346) -> ()  [unwired: 1 out]
        n641 = local read "STOP"() -> (w1364:bool)
        n642 = call <vilib>:"Release Semaphore.vi"("error in (no error)"=w1349, "semaphore"=w1350) -> ("error out"=w1347:errorcluster, "semaphore out"=w1348:T8)  [unwired: 4 in]
      }
    }
    frame Enabled {
    }
  }
  n643 = while {
    shift-right: [w1423] -> w18
    shift-left: w2 -> [w1425]
    shift-right: [w1422] -> w19
    shift-left: w1 -> [w1424]
    shift-right: [w1418] -> w14
    shift-left: w8 -> [w1420]
    shift-right: [w1419] -> w15
    shift-left: w9 -> [w1421]
    tunnel: w11 -> [_]
    tunnel: w10 -> [_]
    tunnel: w4 -> [w1417]
    tunnel: w3 -> [w1416]
    tunnel: [w1415] -> w7
    tunnel: [w1414] -> w6
    stop <- w1427 stop-if-true
    n644 = event shown="[5] \"Floors Schematic.Call 5\", \"Elevator Panel.Floor 5\": Value Change" {
      selector: _ -> [_ _ _ _ _ _ _ _ _ _ _ _ _ _ _]
      dyn-events: _ -> [_ _ _ _ _ _ _ _ _ _ _ _ _ _ _]
      timeout: 100 -> [_ _ _ _ _ _ _ _ _ _ _ _ _ _ _]
      tunnel: w1425 -> [w1439 w1478 w1581 w1682 w1785 w1886 w1987 w2088 w2189 w2290 w2391 w2492 w2593 w2689 w2787]
      tunnel: w1424 -> [w1438 w1477 w1580 w1681 w1784 w1885 w1986 w2087 w2188 w2289 w2390 w2491 w2592 w2688 w2786]
      tunnel: [w1437 w1476 w1579 w1680 w1783 w1884 w1985 w2086 w2187 w2288 w2389 w2490 w2591 w2689 w2787] -> w1423
      tunnel: [w1436 w1475 w1578 w1679 w1782 w1883 w1984 w2085 w2186 w2287 w2388 w2489 w2590 w2688 w2786] -> w1422
      tunnel: w1421 -> [w1443 w1472 w1575 w1676 w1779 w1880 w1981 w2082 w2183 w2284 w2385 w2486 w2587 w2693 w2791]
      tunnel: w1420 -> [w1442 w1470 w1573 w1674 w1777 w1878 w1979 w2080 w2181 w2282 w2383 w2484 w2585 w2691 w2790]
      tunnel: [w1441 w1473 w1576 w1677 w1780 w1881 w1982 w2083 w2184 w2285 w2386 w2487 w2588 w2692 w2789] -> w1419
      tunnel: [w1440 w1471 w1574 w1675 w1778 w1879 w1980 w2081 w2182 w2283 w2384 w2485 w2586 w2690 w2788] -> w1418
      tunnel: w1417 -> [w1433 w1469 w1572 w1672 w1776 w1877 w1978 w2078 w2179 w2281 w2382 w2482 w2584 w2686 w2784]
      tunnel: w1416 -> [w1432 w1468 w1571 w1673 w1775 w1876 w1977 w2079 w2180 w2280 w2381 w2483 w2583 w2687 w2785]
      tunnel: [w1429 w1463 w1566 w1669 w1770 w1873 w1974 w2075 w2176 w2277 w2378 w2479 w2581 w2681 w2778] -> w1415
      tunnel: [w1428 w1462 w1565 w1668 w1769 w1872 w1973 w2074 w2175 w2276 w2377 w2478 w2579 w2680 w2781] -> w1414
      event Timeout {
        n645 = event-data() -> ()  [unwired: 1 in, 3 out]
        n646 = call <vilib>:"Acquire Semaphore.vi"("error in (no error)"=w1432, "semaphore"=w1433) -> ("error out"=w1434:errorcluster, "semaphore out"=w1435:T8)  [unwired: 3 in, 1 out]
        n647 = flat-sequence {
          tunnel: w1443 -> [w1458]
          tunnel: w1442 -> [w1457]
          tunnel: [w1456] -> w1441
          tunnel: [w1455] -> w1440
          tunnel: w1439 -> [w1454]
          tunnel: w1438 -> [w1453]
          tunnel: [w1452] -> w1437
          tunnel: [w1451] -> w1436
          tunnel: w1435 -> [w1450]
          tunnel: w1434 -> [w1449]
          tunnel: [w1448] -> w1431
          tunnel: [w1447] -> w1430
          frame #0 {
            n648 = Get Queue Status(queue=w1454, error in (no error)=w1453) -> (queue out=w1452:refnum<queue>, error out=w1451:errorcluster, # elements in queue=→"# elements in Elevator Floor Queue":i32, elements=→"Elevator Floor Queue":u8[])  [unwired: 1 in, 4 out]
            n649 = call <vilib>:"Get Semaphore Status.vi"("error in (no error)"=w1449, "semaphore"=w1450) -> ("error out"=w1447:errorcluster, "# waiting"=→"# waiting":i32, "# available"=→"# available":i32, "semaphore out"=w1448:T8, "size"=→"size":i32)  [unwired: 4 in, 1 out]
            n650 = Get Queue Status(queue=w1458, error in (no error)=w1457) -> (queue out=w1456:refnum<queue>, error out=w1455:errorcluster, elements=→"Elevator Command Queue":T1[])  [unwired: 1 in, 5 out]
          }
        }
        n651 = call <vilib>:"Release Semaphore.vi"("error in (no error)"=w1430, "semaphore"=w1431) -> ("error out"=w1428:errorcluster, "semaphore out"=w1429:T8)  [unwired: 4 in]
      }
      event Value Change {
        n652 = event-data() -> ("NewVal"=w1474:bool)  [unwired: 1 in, 5 out]
        n653 = call <vilib>:"Acquire Semaphore.vi"("error in (no error)"=w1468, "semaphore"=w1469) -> ("error out"=w1466:errorcluster, "semaphore out"=w1467:T8)  [unwired: 3 in, 1 out]
        n654 = flat-sequence {
          tunnel: w1478 -> [w1491]
          tunnel: w1477 -> [w1490]
          tunnel: [w1489] -> w1476
          tunnel: [w1488] -> w1475
          tunnel: w1474 -> [w1487]
          tunnel: [w1486] -> w1473
          tunnel: w1472 -> [w1485]
          tunnel: [w1484] -> w1471
          tunnel: w1470 -> [w1483]
          tunnel: w1467 -> [w1482]
          tunnel: w1466 -> [w1480]
          tunnel: [w1481] -> w1465
          tunnel: [w1479] -> w1464
          frame #0 {
            n655 = case shown="True" w1487 {
              tunnel: w1491 -> [w1497 w1518]
              tunnel: w1490 -> [w1496 w1517]
              tunnel: [w1497 w1518] -> w1489
              tunnel: [w1496 w1517] -> w1488
              tunnel: [w1495 w1516] -> w1486
              tunnel: w1485 -> [w1495 w1507]
              tunnel: [w1494 w1515] -> w1484
              tunnel: w1483 -> [w1494 w1506]
              tunnel: w1482 -> [w1493 w1499]
              tunnel: [w1493 w1499] -> w1481
              tunnel: w1480 -> [w1492 w1498]
              tunnel: [w1492 w1498] -> w1479
              frame False {
              }
              frame True {
                n656 = control-ref of="Elevator Cabin"() -> (w1514:refnum<vi>)
                n657 = property class="Slide (strict)"(reference=w1514) -> ("Top"=w1513:i32)  [unwired: 1 in, 2 out]
                n658 = local read "Floors Schematic"() -> (w1511:T4)
                n659 = Preview Queue Element(queue=w1507, timeout in ms (-1)=1, error in (no error)=w1506) -> (timed out?=w1505:bool)  [unwired: 3 out]
                n660 = Unbundle By Name(w1511) -> ("Floor Position"=w1512:i16[])
                n661 = Decrement(x=1 ("32bit integer")) -> (x-1=w1501:i32)
                n662 = Index Array(array=w1512, index=w1501) -> (element=w1509:i16)
                n663 = To Long Integer(number=w1509) -> (32bit integer=w1510:i32)
                n664 = Not Equal?(x=w1510, y=w1513) -> (x != y?=w1504:bool)
                n665 = Select(t=TRUE, s=w1505, f=w1504) -> (s? t:f=w1502:bool)
                n666 = case shown="False" w1502 {
                  tunnel: w1507 -> [w1520 w1532]
                  tunnel: w1506 -> [w1519 w1531]
                  tunnel: [w1520 w1530] -> w1516
                  tunnel: [w1519 w1529] -> w1515
                  frame True {
                    n667 = local read "Elevator Automate"() -> (w1522:T2)
                    n668 = Bundle By Name(cluster=w1522, "Cancel Delay"=TRUE ("Add to Queue")) -> (w1523:T2)
                    n669 = local write "Elevator Automate"(w1523) -> ()
                  }
                  frame False {
                    n670 = local read "Elevator Automate"() -> (w1536:T2)
                    n671 = Unbundle By Name(w1536) -> ("Elevator Command"=w1535:T1)
                    n672 = Equal?(x=w1535, y=Elevator_Command."Close Doors") -> (x = y?=w1533:bool)
                    n673 = case shown="True" w1533 {
                      tunnel: w1532 -> [w1549 w1564]
                      tunnel: w1531 -> [w1548 w1563]
                      tunnel: [w1547 w1564] -> w1530
                      tunnel: [w1546 w1563] -> w1529
                      tunnel: [FALSE ("Call 12") FALSE ("Call 12")] -> w1524
                      frame True {
                        w1559 = T9 20 items=["Floor Length"=48, "Sum of Floors"=12, "Floor Step in ms"=63, "Elevator Door Step in ms"=30, "Global Wait in ms"=20, "Event Wait in ms"=100] ("Elevator Constants")
                        n674 = local read "Elevator Automate"() -> (w1558:T2)
                        n675 = Flush Queue(queue=w1549, error in (no error)=w1548) -> (queue out=w1545:refnum<queue>, error out=w1544:errorcluster)  [unwired: 1 out]
                        n676 = To Long Integer(number=w1559) -> (32bit integer=w1560:i32)
                        n677 = Preview Queue Element(queue=w1545, timeout in ms (-1)=w1560, error in (no error)=w1544) -> (queue out=w1539:refnum<queue>, timed out?=w1538:bool, error out=w1540:errorcluster)  [unwired: 1 out]
                        n678 = Bundle By Name(cluster=w1558, "Forced Stop"=w1538) -> (w1557:T2)
                        n679 = Enqueue Element(queue=w1539, element=Elevator_Command."Open Doors", error in (no error)=w1540) -> (queue out=w1542:refnum<queue>, error out=w1541:errorcluster)  [unwired: 1 in, 1 out]
                        n680 = local write "Elevator Automate"(w1557) -> ()
                        n681 = Enqueue Element(queue=w1542, element=Elevator_Command."Long Delay", error in (no error)=w1541) -> (queue out=w1556:refnum<queue>, error out=w1555:errorcluster)  [unwired: 1 in, 1 out]
                        n682 = Enqueue Element(queue=w1556, element=Elevator_Command."Close Doors", error in (no error)=w1555) -> (queue out=w1554:refnum<queue>, error out=w1553:errorcluster)  [unwired: 1 in, 1 out]
                        n683 = Enqueue Element(queue=w1554, element=Elevator_Command."Idle", error in (no error)=w1553) -> (queue out=w1547:refnum<queue>, error out=w1546:errorcluster)  [unwired: 1 in, 1 out]
                      }
                      frame False {
                        n684 = Wait (ms)(milliseconds to wait=u32 250) -> ()  [unwired: 1 out]
                      }
                    }
                    n685 = local read "Floors Schematic"() -> (w1528:T4)
                    n686 = local read "Elevator Panel"() -> (w1526:T3)
                    n687 = Bundle By Name(cluster=w1528, "Call 1"=w1524) -> (w1527:T4)
                    n688 = Bundle By Name(cluster=w1526, "Floor 1"=w1524) -> (w1525:T3)
                    n689 = local write "Elevator Panel"(w1525) -> ()
                    n690 = local write "Floors Schematic"(w1527) -> ()
                  }
                }
              }
            }
          }
        }
        n691 = call <vilib>:"Release Semaphore.vi"("error in (no error)"=w1464, "semaphore"=w1465) -> ("error out"=w1462:errorcluster, "semaphore out"=w1463:T8)  [unwired: 4 in]
      }
      event Value Change {
        n692 = event-data() -> ("NewVal"=w1577:bool)  [unwired: 1 in, 5 out]
        n693 = call <vilib>:"Acquire Semaphore.vi"("error in (no error)"=w1571, "semaphore"=w1572) -> ("error out"=w1569:errorcluster, "semaphore out"=w1570:T8)  [unwired: 3 in, 1 out]
        n694 = flat-sequence {
          tunnel: w1581 -> [w1594]
          tunnel: w1580 -> [w1593]
          tunnel: [w1592] -> w1579
          tunnel: [w1591] -> w1578
          tunnel: w1577 -> [w1590]
          tunnel: [w1589] -> w1576
          tunnel: w1575 -> [w1588]
          tunnel: [w1587] -> w1574
          tunnel: w1573 -> [w1586]
          tunnel: w1570 -> [w1585]
          tunnel: w1569 -> [w1583]
          tunnel: [w1584] -> w1568
          tunnel: [w1582] -> w1567
          frame #0 {
            n695 = case shown="True" w1590 {
              tunnel: w1594 -> [w1600 w1621]
              tunnel: w1593 -> [w1599 w1620]
              tunnel: [w1600 w1621] -> w1592
              tunnel: [w1599 w1620] -> w1591
              tunnel: [w1598 w1619] -> w1589
              tunnel: w1588 -> [w1598 w1610]
              tunnel: [w1597 w1618] -> w1587
              tunnel: w1586 -> [w1597 w1609]
              tunnel: w1585 -> [w1596 w1602]
              tunnel: [w1596 w1602] -> w1584
              tunnel: w1583 -> [w1595 w1601]
              tunnel: [w1595 w1601] -> w1582
              frame False {
              }
              frame True {
                n696 = control-ref of="Elevator Cabin"() -> (w1617:refnum<vi>)
                n697 = property class="Slide (strict)"(reference=w1617) -> ("Top"=w1616:i32)  [unwired: 1 in, 2 out]
                n698 = local read "Floors Schematic"() -> (w1614:T4)
                n699 = Preview Queue Element(queue=w1610, timeout in ms (-1)=1, error in (no error)=w1609) -> (timed out?=w1608:bool)  [unwired: 3 out]
                n700 = Unbundle By Name(w1614) -> ("Floor Position"=w1615:i16[])
                n701 = Decrement(x=2 ("32bit integer")) -> (x-1=w1604:i32)
                n702 = Index Array(array=w1615, index=w1604) -> (element=w1612:i16)
                n703 = To Long Integer(number=w1612) -> (32bit integer=w1613:i32)
                n704 = Not Equal?(x=w1613, y=w1616) -> (x != y?=w1607:bool)
                n705 = Select(t=TRUE, s=w1608, f=w1607) -> (s? t:f=w1605:bool)
                n706 = case shown="False" w1605 {
                  tunnel: w1610 -> [w1623 w1635]
                  tunnel: w1609 -> [w1622 w1634]
                  tunnel: [w1623 w1633] -> w1619
                  tunnel: [w1622 w1632] -> w1618
                  frame True {
                    n707 = local read "Elevator Automate"() -> (w1625:T2)
                    n708 = Bundle By Name(cluster=w1625, "Cancel Delay"=TRUE ("Add to Queue")) -> (w1626:T2)
                    n709 = local write "Elevator Automate"(w1626) -> ()
                  }
                  frame False {
                    n710 = local read "Elevator Automate"() -> (w1639:T2)
                    n711 = Unbundle By Name(w1639) -> ("Elevator Command"=w1638:T1)
                    n712 = Equal?(x=w1638, y=Elevator_Command."Close Doors") -> (x = y?=w1636:bool)
                    n713 = case shown="True" w1636 {
                      tunnel: w1635 -> [w1652 w1667]
                      tunnel: w1634 -> [w1651 w1666]
                      tunnel: [w1650 w1667] -> w1633
                      tunnel: [w1649 w1666] -> w1632
                      tunnel: [FALSE ("Call 12") FALSE ("Call 12")] -> w1627
                      frame True {
                        w1662 = T9 20 items=["Floor Length"=48, "Sum of Floors"=12, "Floor Step in ms"=63, "Elevator Door Step in ms"=30, "Global Wait in ms"=20, "Event Wait in ms"=100] ("Elevator Constants")
                        n714 = local read "Elevator Automate"() -> (w1661:T2)
                        n715 = Flush Queue(queue=w1652, error in (no error)=w1651) -> (queue out=w1648:refnum<queue>, error out=w1647:errorcluster)  [unwired: 1 out]
                        n716 = To Long Integer(number=w1662) -> (32bit integer=w1663:i32)
                        n717 = Preview Queue Element(queue=w1648, timeout in ms (-1)=w1663, error in (no error)=w1647) -> (queue out=w1642:refnum<queue>, timed out?=w1641:bool, error out=w1643:errorcluster)  [unwired: 1 out]
                        n718 = Bundle By Name(cluster=w1661, "Forced Stop"=w1641) -> (w1660:T2)
                        n719 = Enqueue Element(queue=w1642, element=Elevator_Command."Open Doors", error in (no error)=w1643) -> (queue out=w1645:refnum<queue>, error out=w1644:errorcluster)  [unwired: 1 in, 1 out]
                        n720 = local write "Elevator Automate"(w1660) -> ()
                        n721 = Enqueue Element(queue=w1645, element=Elevator_Command."Long Delay", error in (no error)=w1644) -> (queue out=w1659:refnum<queue>, error out=w1658:errorcluster)  [unwired: 1 in, 1 out]
                        n722 = Enqueue Element(queue=w1659, element=Elevator_Command."Close Doors", error in (no error)=w1658) -> (queue out=w1657:refnum<queue>, error out=w1656:errorcluster)  [unwired: 1 in, 1 out]
                        n723 = Enqueue Element(queue=w1657, element=Elevator_Command."Idle", error in (no error)=w1656) -> (queue out=w1650:refnum<queue>, error out=w1649:errorcluster)  [unwired: 1 in, 1 out]
                      }
                      frame False {
                        n724 = Wait (ms)(milliseconds to wait=u32 250) -> ()  [unwired: 1 out]
                      }
                    }
                    n725 = local read "Floors Schematic"() -> (w1631:T4)
                    n726 = local read "Elevator Panel"() -> (w1629:T3)
                    n727 = Bundle By Name(cluster=w1631, "Call 2"=w1627) -> (w1630:T4)
                    n728 = Bundle By Name(cluster=w1629, "Floor 2"=w1627) -> (w1628:T3)
                    n729 = local write "Elevator Panel"(w1628) -> ()
                    n730 = local write "Floors Schematic"(w1630) -> ()
                  }
                }
              }
            }
          }
        }
        n731 = call <vilib>:"Release Semaphore.vi"("error in (no error)"=w1567, "semaphore"=w1568) -> ("error out"=w1565:errorcluster, "semaphore out"=w1566:T8)  [unwired: 4 in]
      }
      event Value Change {
        n732 = event-data() -> ("NewVal"=w1678:bool)  [unwired: 1 in, 5 out]
        n733 = call <vilib>:"Acquire Semaphore.vi"("error in (no error)"=w1673, "semaphore"=w1672) -> ("error out"=w1670:errorcluster, "semaphore out"=w1671:T8)  [unwired: 3 in, 1 out]
        n734 = flat-sequence {
          tunnel: w1682 -> [w1695]
          tunnel: w1681 -> [w1694]
          tunnel: [w1693] -> w1680
          tunnel: [w1692] -> w1679
          tunnel: w1678 -> [w1691]
          tunnel: [w1690] -> w1677
          tunnel: w1676 -> [w1689]
          tunnel: [w1688] -> w1675
          tunnel: w1674 -> [w1687]
          tunnel: w1671 -> [w1686]
          tunnel: w1670 -> [w1684]
          tunnel: [w1685] -> w1669
          tunnel: [w1683] -> w1668
          frame #0 {
            n735 = case shown="True" w1691 {
              tunnel: w1695 -> [w1701 w1722]
              tunnel: w1694 -> [w1700 w1721]
              tunnel: [w1701 w1722] -> w1693
              tunnel: [w1700 w1721] -> w1692
              tunnel: [w1699 w1720] -> w1690
              tunnel: w1689 -> [w1699 w1711]
              tunnel: [w1698 w1719] -> w1688
              tunnel: w1687 -> [w1698 w1710]
              tunnel: w1686 -> [w1697 w1703]
              tunnel: [w1697 w1703] -> w1685
              tunnel: w1684 -> [w1696 w1702]
              tunnel: [w1696 w1702] -> w1683
              frame False {
              }
              frame True {
                n736 = control-ref of="Elevator Cabin"() -> (w1718:refnum<vi>)
                n737 = property class="Slide (strict)"(reference=w1718) -> ("Top"=w1717:i32)  [unwired: 1 in, 2 out]
                n738 = local read "Floors Schematic"() -> (w1715:T4)
                n739 = Preview Queue Element(queue=w1711, timeout in ms (-1)=1, error in (no error)=w1710) -> (timed out?=w1709:bool)  [unwired: 3 out]
                n740 = Unbundle By Name(w1715) -> ("Floor Position"=w1716:i16[])
                n741 = Decrement(x=3 ("32bit integer")) -> (x-1=w1705:i32)
                n742 = Index Array(array=w1716, index=w1705) -> (element=w1713:i16)
                n743 = To Long Integer(number=w1713) -> (32bit integer=w1714:i32)
                n744 = Not Equal?(x=w1714, y=w1717) -> (x != y?=w1708:bool)
                n745 = Select(t=TRUE, s=w1709, f=w1708) -> (s? t:f=w1706:bool)
                n746 = case shown="False" w1706 {
                  tunnel: w1711 -> [w1724 w1736]
                  tunnel: w1710 -> [w1723 w1735]
                  tunnel: [w1724 w1734] -> w1720
                  tunnel: [w1723 w1733] -> w1719
                  frame True {
                    n747 = local read "Elevator Automate"() -> (w1726:T2)
                    n748 = Bundle By Name(cluster=w1726, "Cancel Delay"=TRUE ("Add to Queue")) -> (w1727:T2)
                    n749 = local write "Elevator Automate"(w1727) -> ()
                  }
                  frame False {
                    n750 = local read "Elevator Automate"() -> (w1740:T2)
                    n751 = Unbundle By Name(w1740) -> ("Elevator Command"=w1739:T1)
                    n752 = Equal?(x=w1739, y=Elevator_Command."Close Doors") -> (x = y?=w1737:bool)
                    n753 = case shown="True" w1737 {
                      tunnel: w1736 -> [w1753 w1768]
                      tunnel: w1735 -> [w1752 w1767]
                      tunnel: [w1751 w1768] -> w1734
                      tunnel: [w1750 w1767] -> w1733
                      tunnel: [FALSE ("Call 12") FALSE ("Call 12")] -> w1728
                      frame True {
                        w1763 = T9 20 items=["Floor Length"=48, "Sum of Floors"=12, "Floor Step in ms"=63, "Elevator Door Step in ms"=30, "Global Wait in ms"=20, "Event Wait in ms"=100] ("Elevator Constants")
                        n754 = local read "Elevator Automate"() -> (w1762:T2)
                        n755 = Flush Queue(queue=w1753, error in (no error)=w1752) -> (queue out=w1749:refnum<queue>, error out=w1748:errorcluster)  [unwired: 1 out]
                        n756 = To Long Integer(number=w1763) -> (32bit integer=w1764:i32)
                        n757 = Preview Queue Element(queue=w1749, timeout in ms (-1)=w1764, error in (no error)=w1748) -> (queue out=w1743:refnum<queue>, timed out?=w1742:bool, error out=w1744:errorcluster)  [unwired: 1 out]
                        n758 = Bundle By Name(cluster=w1762, "Forced Stop"=w1742) -> (w1761:T2)
                        n759 = Enqueue Element(queue=w1743, element=Elevator_Command."Open Doors", error in (no error)=w1744) -> (queue out=w1746:refnum<queue>, error out=w1745:errorcluster)  [unwired: 1 in, 1 out]
                        n760 = local write "Elevator Automate"(w1761) -> ()
                        n761 = Enqueue Element(queue=w1746, element=Elevator_Command."Long Delay", error in (no error)=w1745) -> (queue out=w1760:refnum<queue>, error out=w1759:errorcluster)  [unwired: 1 in, 1 out]
                        n762 = Enqueue Element(queue=w1760, element=Elevator_Command."Close Doors", error in (no error)=w1759) -> (queue out=w1758:refnum<queue>, error out=w1757:errorcluster)  [unwired: 1 in, 1 out]
                        n763 = Enqueue Element(queue=w1758, element=Elevator_Command."Idle", error in (no error)=w1757) -> (queue out=w1751:refnum<queue>, error out=w1750:errorcluster)  [unwired: 1 in, 1 out]
                      }
                      frame False {
                        n764 = Wait (ms)(milliseconds to wait=u32 250) -> ()  [unwired: 1 out]
                      }
                    }
                    n765 = local read "Floors Schematic"() -> (w1732:T4)
                    n766 = local read "Elevator Panel"() -> (w1730:T3)
                    n767 = Bundle By Name(cluster=w1732, "Call 3"=w1728) -> (w1731:T4)
                    n768 = Bundle By Name(cluster=w1730, "Floor 3"=w1728) -> (w1729:T3)
                    n769 = local write "Elevator Panel"(w1729) -> ()
                    n770 = local write "Floors Schematic"(w1731) -> ()
                  }
                }
              }
            }
          }
        }
      }
      event Value Change {
        n771 = event-data() -> ("NewVal"=w1781:bool)  [unwired: 1 in, 5 out]
        n772 = call <vilib>:"Acquire Semaphore.vi"("error in (no error)"=w1775, "semaphore"=w1776) -> ("error out"=w1773:errorcluster, "semaphore out"=w1774:T8)  [unwired: 3 in, 1 out]
        n773 = flat-sequence {
          tunnel: w1785 -> [w1798]
          tunnel: w1784 -> [w1797]
          tunnel: [w1796] -> w1783
          tunnel: [w1795] -> w1782
          tunnel: w1781 -> [w1794]
          tunnel: [w1793] -> w1780
          tunnel: w1779 -> [w1792]
          tunnel: [w1791] -> w1778
          tunnel: w1777 -> [w1790]
          tunnel: w1774 -> [w1789]
          tunnel: w1773 -> [w1787]
          tunnel: [w1788] -> w1772
          tunnel: [w1786] -> w1771
          frame #0 {
            n774 = case shown="True" w1794 {
              tunnel: w1798 -> [w1804 w1825]
              tunnel: w1797 -> [w1803 w1824]
              tunnel: [w1804 w1825] -> w1796
              tunnel: [w1803 w1824] -> w1795
              tunnel: [w1802 w1823] -> w1793
              tunnel: w1792 -> [w1802 w1814]
              tunnel: [w1801 w1822] -> w1791
              tunnel: w1790 -> [w1801 w1813]
              tunnel: w1789 -> [w1800 w1806]
              tunnel: [w1800 w1806] -> w1788
              tunnel: w1787 -> [w1799 w1805]
              tunnel: [w1799 w1805] -> w1786
              frame False {
              }
              frame True {
                n775 = control-ref of="Elevator Cabin"() -> (w1821:refnum<vi>)
                n776 = property class="Slide (strict)"(reference=w1821) -> ("Top"=w1820:i32)  [unwired: 1 in, 2 out]
                n777 = local read "Floors Schematic"() -> (w1818:T4)
                n778 = Preview Queue Element(queue=w1814, timeout in ms (-1)=1, error in (no error)=w1813) -> (timed out?=w1812:bool)  [unwired: 3 out]
                n779 = Unbundle By Name(w1818) -> ("Floor Position"=w1819:i16[])
                n780 = Decrement(x=4 ("32bit integer")) -> (x-1=w1808:i32)
                n781 = Index Array(array=w1819, index=w1808) -> (element=w1816:i16)
                n782 = To Long Integer(number=w1816) -> (32bit integer=w1817:i32)
                n783 = Not Equal?(x=w1817, y=w1820) -> (x != y?=w1811:bool)
                n784 = Select(t=TRUE, s=w1812, f=w1811) -> (s? t:f=w1809:bool)
                n785 = case shown="False" w1809 {
                  tunnel: w1814 -> [w1827 w1839]
                  tunnel: w1813 -> [w1826 w1838]
                  tunnel: [w1827 w1837] -> w1823
                  tunnel: [w1826 w1836] -> w1822
                  frame True {
                    n786 = local read "Elevator Automate"() -> (w1829:T2)
                    n787 = Bundle By Name(cluster=w1829, "Cancel Delay"=TRUE ("Add to Queue")) -> (w1830:T2)
                    n788 = local write "Elevator Automate"(w1830) -> ()
                  }
                  frame False {
                    n789 = local read "Elevator Automate"() -> (w1843:T2)
                    n790 = Unbundle By Name(w1843) -> ("Elevator Command"=w1842:T1)
                    n791 = Equal?(x=w1842, y=Elevator_Command."Close Doors") -> (x = y?=w1840:bool)
                    n792 = case shown="True" w1840 {
                      tunnel: w1839 -> [w1856 w1871]
                      tunnel: w1838 -> [w1855 w1870]
                      tunnel: [w1854 w1871] -> w1837
                      tunnel: [w1853 w1870] -> w1836
                      tunnel: [FALSE ("Call 12") FALSE ("Call 12")] -> w1831
                      frame True {
                        w1866 = T9 20 items=["Floor Length"=48, "Sum of Floors"=12, "Floor Step in ms"=63, "Elevator Door Step in ms"=30, "Global Wait in ms"=20, "Event Wait in ms"=100] ("Elevator Constants")
                        n793 = local read "Elevator Automate"() -> (w1865:T2)
                        n794 = Flush Queue(queue=w1856, error in (no error)=w1855) -> (queue out=w1852:refnum<queue>, error out=w1851:errorcluster)  [unwired: 1 out]
                        n795 = To Long Integer(number=w1866) -> (32bit integer=w1867:i32)
                        n796 = Preview Queue Element(queue=w1852, timeout in ms (-1)=w1867, error in (no error)=w1851) -> (queue out=w1846:refnum<queue>, timed out?=w1845:bool, error out=w1847:errorcluster)  [unwired: 1 out]
                        n797 = Bundle By Name(cluster=w1865, "Forced Stop"=w1845) -> (w1864:T2)
                        n798 = Enqueue Element(queue=w1846, element=Elevator_Command."Open Doors", error in (no error)=w1847) -> (queue out=w1849:refnum<queue>, error out=w1848:errorcluster)  [unwired: 1 in, 1 out]
                        n799 = local write "Elevator Automate"(w1864) -> ()
                        n800 = Enqueue Element(queue=w1849, element=Elevator_Command."Long Delay", error in (no error)=w1848) -> (queue out=w1863:refnum<queue>, error out=w1862:errorcluster)  [unwired: 1 in, 1 out]
                        n801 = Enqueue Element(queue=w1863, element=Elevator_Command."Close Doors", error in (no error)=w1862) -> (queue out=w1861:refnum<queue>, error out=w1860:errorcluster)  [unwired: 1 in, 1 out]
                        n802 = Enqueue Element(queue=w1861, element=Elevator_Command."Idle", error in (no error)=w1860) -> (queue out=w1854:refnum<queue>, error out=w1853:errorcluster)  [unwired: 1 in, 1 out]
                      }
                      frame False {
                        n803 = Wait (ms)(milliseconds to wait=u32 250) -> ()  [unwired: 1 out]
                      }
                    }
                    n804 = local read "Floors Schematic"() -> (w1835:T4)
                    n805 = local read "Elevator Panel"() -> (w1833:T3)
                    n806 = Bundle By Name(cluster=w1835, "Call 4"=w1831) -> (w1834:T4)
                    n807 = Bundle By Name(cluster=w1833, "Floor 4"=w1831) -> (w1832:T3)
                    n808 = local write "Elevator Panel"(w1832) -> ()
                    n809 = local write "Floors Schematic"(w1834) -> ()
                  }
                }
              }
            }
          }
        }
        n810 = call <vilib>:"Release Semaphore.vi"("error in (no error)"=w1771, "semaphore"=w1772) -> ("error out"=w1769:errorcluster, "semaphore out"=w1770:T8)  [unwired: 4 in]
      }
      event Value Change {
        n811 = event-data() -> ("NewVal"=w1882:bool)  [unwired: 1 in, 5 out]
        n812 = call <vilib>:"Acquire Semaphore.vi"("error in (no error)"=w1876, "semaphore"=w1877) -> ("error out"=w1874:errorcluster, "semaphore out"=w1875:T8)  [unwired: 3 in, 1 out]
        n813 = flat-sequence {
          tunnel: w1886 -> [w1899]
          tunnel: w1885 -> [w1898]
          tunnel: [w1897] -> w1884
          tunnel: [w1896] -> w1883
          tunnel: w1882 -> [w1895]
          tunnel: [w1894] -> w1881
          tunnel: w1880 -> [w1893]
          tunnel: [w1892] -> w1879
          tunnel: w1878 -> [w1891]
          tunnel: w1875 -> [w1890]
          tunnel: w1874 -> [w1888]
          tunnel: [w1889] -> w1873
          tunnel: [w1887] -> w1872
          frame #0 {
            n814 = case shown="True" w1895 {
              tunnel: w1899 -> [w1905 w1926]
              tunnel: w1898 -> [w1904 w1925]
              tunnel: [w1905 w1926] -> w1897
              tunnel: [w1904 w1925] -> w1896
              tunnel: [w1903 w1924] -> w1894
              tunnel: w1893 -> [w1903 w1915]
              tunnel: [w1902 w1923] -> w1892
              tunnel: w1891 -> [w1902 w1914]
              tunnel: w1890 -> [w1901 w1907]
              tunnel: [w1901 w1907] -> w1889
              tunnel: w1888 -> [w1900 w1906]
              tunnel: [w1900 w1906] -> w1887
              frame False {
              }
              frame True {
                n815 = control-ref of="Elevator Cabin"() -> (w1922:refnum<vi>)
                n816 = property class="Slide (strict)"(reference=w1922) -> ("Top"=w1921:i32)  [unwired: 1 in, 2 out]
                n817 = local read "Floors Schematic"() -> (w1919:T4)
                n818 = Preview Queue Element(queue=w1915, timeout in ms (-1)=1, error in (no error)=w1914) -> (timed out?=w1913:bool)  [unwired: 3 out]
                n819 = Unbundle By Name(w1919) -> ("Floor Position"=w1920:i16[])
                n820 = Decrement(x=5 ("32bit integer")) -> (x-1=w1909:i32)
                n821 = Index Array(array=w1920, index=w1909) -> (element=w1917:i16)
                n822 = To Long Integer(number=w1917) -> (32bit integer=w1918:i32)
                n823 = Not Equal?(x=w1918, y=w1921) -> (x != y?=w1912:bool)
                n824 = Select(t=TRUE, s=w1913, f=w1912) -> (s? t:f=w1910:bool)
                n825 = case shown="False" w1910 {
                  tunnel: w1915 -> [w1928 w1940]
                  tunnel: w1914 -> [w1927 w1939]
                  tunnel: [w1928 w1938] -> w1924
                  tunnel: [w1927 w1937] -> w1923
                  frame True {
                    n826 = local read "Elevator Automate"() -> (w1930:T2)
                    n827 = Bundle By Name(cluster=w1930, "Cancel Delay"=TRUE ("Add to Queue")) -> (w1931:T2)
                    n828 = local write "Elevator Automate"(w1931) -> ()
                  }
                  frame False {
                    n829 = local read "Elevator Automate"() -> (w1944:T2)
                    n830 = Unbundle By Name(w1944) -> ("Elevator Command"=w1943:T1)
                    n831 = Equal?(x=w1943, y=Elevator_Command."Close Doors") -> (x = y?=w1941:bool)
                    n832 = case shown="True" w1941 {
                      tunnel: w1940 -> [w1957 w1972]
                      tunnel: w1939 -> [w1956 w1971]
                      tunnel: [w1955 w1972] -> w1938
                      tunnel: [w1954 w1971] -> w1937
                      tunnel: [FALSE ("Call 12") FALSE ("Call 12")] -> w1932
                      frame True {
                        w1967 = T9 20 items=["Floor Length"=48, "Sum of Floors"=12, "Floor Step in ms"=63, "Elevator Door Step in ms"=30, "Global Wait in ms"=20, "Event Wait in ms"=100] ("Elevator Constants")
                        n833 = local read "Elevator Automate"() -> (w1966:T2)
                        n834 = Flush Queue(queue=w1957, error in (no error)=w1956) -> (queue out=w1953:refnum<queue>, error out=w1952:errorcluster)  [unwired: 1 out]
                        n835 = To Long Integer(number=w1967) -> (32bit integer=w1968:i32)
                        n836 = Preview Queue Element(queue=w1953, timeout in ms (-1)=w1968, error in (no error)=w1952) -> (queue out=w1947:refnum<queue>, timed out?=w1946:bool, error out=w1948:errorcluster)  [unwired: 1 out]
                        n837 = Bundle By Name(cluster=w1966, "Forced Stop"=w1946) -> (w1965:T2)
                        n838 = Enqueue Element(queue=w1947, element=Elevator_Command."Open Doors", error in (no error)=w1948) -> (queue out=w1950:refnum<queue>, error out=w1949:errorcluster)  [unwired: 1 in, 1 out]
                        n839 = local write "Elevator Automate"(w1965) -> ()
                        n840 = Enqueue Element(queue=w1950, element=Elevator_Command."Long Delay", error in (no error)=w1949) -> (queue out=w1964:refnum<queue>, error out=w1963:errorcluster)  [unwired: 1 in, 1 out]
                        n841 = Enqueue Element(queue=w1964, element=Elevator_Command."Close Doors", error in (no error)=w1963) -> (queue out=w1962:refnum<queue>, error out=w1961:errorcluster)  [unwired: 1 in, 1 out]
                        n842 = Enqueue Element(queue=w1962, element=Elevator_Command."Idle", error in (no error)=w1961) -> (queue out=w1955:refnum<queue>, error out=w1954:errorcluster)  [unwired: 1 in, 1 out]
                      }
                      frame False {
                        n843 = Wait (ms)(milliseconds to wait=u32 250) -> ()  [unwired: 1 out]
                      }
                    }
                    n844 = local read "Floors Schematic"() -> (w1936:T4)
                    n845 = local read "Elevator Panel"() -> (w1934:T3)
                    n846 = Bundle By Name(cluster=w1936, "Call 5"=w1932) -> (w1935:T4)
                    n847 = Bundle By Name(cluster=w1934, "Floor 5"=w1932) -> (w1933:T3)
                    n848 = local write "Elevator Panel"(w1933) -> ()
                    n849 = local write "Floors Schematic"(w1935) -> ()
                  }
                }
              }
            }
          }
        }
      }
      event Value Change {
        n850 = event-data() -> ("NewVal"=w1983:bool)  [unwired: 1 in, 5 out]
        n851 = call <vilib>:"Acquire Semaphore.vi"("error in (no error)"=w1977, "semaphore"=w1978) -> ("error out"=w1975:errorcluster, "semaphore out"=w1976:T8)  [unwired: 3 in, 1 out]
        n852 = flat-sequence {
          tunnel: w1987 -> [w2000]
          tunnel: w1986 -> [w1999]
          tunnel: [w1998] -> w1985
          tunnel: [w1997] -> w1984
          tunnel: w1983 -> [w1996]
          tunnel: [w1995] -> w1982
          tunnel: w1981 -> [w1994]
          tunnel: [w1993] -> w1980
          tunnel: w1979 -> [w1992]
          tunnel: w1976 -> [w1991]
          tunnel: w1975 -> [w1989]
          tunnel: [w1990] -> w1974
          tunnel: [w1988] -> w1973
          frame #0 {
            n853 = case shown="True" w1996 {
              tunnel: w2000 -> [w2006 w2027]
              tunnel: w1999 -> [w2005 w2026]
              tunnel: [w2006 w2027] -> w1998
              tunnel: [w2005 w2026] -> w1997
              tunnel: [w2004 w2025] -> w1995
              tunnel: w1994 -> [w2004 w2016]
              tunnel: [w2003 w2024] -> w1993
              tunnel: w1992 -> [w2003 w2015]
              tunnel: w1991 -> [w2002 w2008]
              tunnel: [w2002 w2008] -> w1990
              tunnel: w1989 -> [w2001 w2007]
              tunnel: [w2001 w2007] -> w1988
              frame False {
              }
              frame True {
                n854 = control-ref of="Elevator Cabin"() -> (w2023:refnum<vi>)
                n855 = property class="Slide (strict)"(reference=w2023) -> ("Top"=w2022:i32)  [unwired: 1 in, 2 out]
                n856 = local read "Floors Schematic"() -> (w2020:T4)
                n857 = Preview Queue Element(queue=w2016, timeout in ms (-1)=1, error in (no error)=w2015) -> (timed out?=w2014:bool)  [unwired: 3 out]
                n858 = Unbundle By Name(w2020) -> ("Floor Position"=w2021:i16[])
                n859 = Decrement(x=6 ("32bit integer")) -> (x-1=w2010:i32)
                n860 = Index Array(array=w2021, index=w2010) -> (element=w2018:i16)
                n861 = To Long Integer(number=w2018) -> (32bit integer=w2019:i32)
                n862 = Not Equal?(x=w2019, y=w2022) -> (x != y?=w2013:bool)
                n863 = Select(t=TRUE, s=w2014, f=w2013) -> (s? t:f=w2011:bool)
                n864 = case shown="False" w2011 {
                  tunnel: w2016 -> [w2029 w2041]
                  tunnel: w2015 -> [w2028 w2040]
                  tunnel: [w2029 w2039] -> w2025
                  tunnel: [w2028 w2038] -> w2024
                  frame True {
                    n865 = local read "Elevator Automate"() -> (w2031:T2)
                    n866 = Bundle By Name(cluster=w2031, "Cancel Delay"=TRUE ("Add to Queue")) -> (w2032:T2)
                    n867 = local write "Elevator Automate"(w2032) -> ()
                  }
                  frame False {
                    n868 = local read "Elevator Automate"() -> (w2045:T2)
                    n869 = Unbundle By Name(w2045) -> ("Elevator Command"=w2044:T1)
                    n870 = Equal?(x=w2044, y=Elevator_Command."Close Doors") -> (x = y?=w2042:bool)
                    n871 = case shown="True" w2042 {
                      tunnel: w2041 -> [w2058 w2073]
                      tunnel: w2040 -> [w2057 w2072]
                      tunnel: [w2056 w2073] -> w2039
                      tunnel: [w2055 w2072] -> w2038
                      tunnel: [FALSE ("Call 12") FALSE ("Call 12")] -> w2033
                      frame True {
                        w2068 = T9 20 items=["Floor Length"=48, "Sum of Floors"=12, "Floor Step in ms"=63, "Elevator Door Step in ms"=30, "Global Wait in ms"=20, "Event Wait in ms"=100] ("Elevator Constants")
                        n872 = local read "Elevator Automate"() -> (w2067:T2)
                        n873 = Flush Queue(queue=w2058, error in (no error)=w2057) -> (queue out=w2054:refnum<queue>, error out=w2053:errorcluster)  [unwired: 1 out]
                        n874 = To Long Integer(number=w2068) -> (32bit integer=w2069:i32)
                        n875 = Preview Queue Element(queue=w2054, timeout in ms (-1)=w2069, error in (no error)=w2053) -> (queue out=w2048:refnum<queue>, timed out?=w2047:bool, error out=w2049:errorcluster)  [unwired: 1 out]
                        n876 = Bundle By Name(cluster=w2067, "Forced Stop"=w2047) -> (w2066:T2)
                        n877 = Enqueue Element(queue=w2048, element=Elevator_Command."Open Doors", error in (no error)=w2049) -> (queue out=w2051:refnum<queue>, error out=w2050:errorcluster)  [unwired: 1 in, 1 out]
                        n878 = local write "Elevator Automate"(w2066) -> ()
                        n879 = Enqueue Element(queue=w2051, element=Elevator_Command."Long Delay", error in (no error)=w2050) -> (queue out=w2065:refnum<queue>, error out=w2064:errorcluster)  [unwired: 1 in, 1 out]
                        n880 = Enqueue Element(queue=w2065, element=Elevator_Command."Close Doors", error in (no error)=w2064) -> (queue out=w2063:refnum<queue>, error out=w2062:errorcluster)  [unwired: 1 in, 1 out]
                        n881 = Enqueue Element(queue=w2063, element=Elevator_Command."Idle", error in (no error)=w2062) -> (queue out=w2056:refnum<queue>, error out=w2055:errorcluster)  [unwired: 1 in, 1 out]
                      }
                      frame False {
                        n882 = Wait (ms)(milliseconds to wait=u32 250) -> ()  [unwired: 1 out]
                      }
                    }
                    n883 = local read "Floors Schematic"() -> (w2037:T4)
                    n884 = local read "Elevator Panel"() -> (w2035:T3)
                    n885 = Bundle By Name(cluster=w2037, "Call 6"=w2033) -> (w2036:T4)
                    n886 = Bundle By Name(cluster=w2035, "Floor 6"=w2033) -> (w2034:T3)
                    n887 = local write "Elevator Panel"(w2034) -> ()
                    n888 = local write "Floors Schematic"(w2036) -> ()
                  }
                }
              }
            }
          }
        }
      }
      event Value Change {
        n889 = event-data() -> ("NewVal"=w2084:bool)  [unwired: 1 in, 5 out]
        n890 = call <vilib>:"Acquire Semaphore.vi"("error in (no error)"=w2079, "semaphore"=w2078) -> ("error out"=w2076:errorcluster, "semaphore out"=w2077:T8)  [unwired: 3 in, 1 out]
        n891 = flat-sequence {
          tunnel: w2088 -> [w2101]
          tunnel: w2087 -> [w2100]
          tunnel: [w2099] -> w2086
          tunnel: [w2098] -> w2085
          tunnel: w2084 -> [w2097]
          tunnel: [w2096] -> w2083
          tunnel: w2082 -> [w2095]
          tunnel: [w2094] -> w2081
          tunnel: w2080 -> [w2093]
          tunnel: w2077 -> [w2092]
          tunnel: w2076 -> [w2091]
          tunnel: [w2090] -> w2075
          tunnel: [w2089] -> w2074
          frame #0 {
            n892 = case shown="True" w2097 {
              tunnel: w2101 -> [w2107 w2128]
              tunnel: w2100 -> [w2106 w2127]
              tunnel: [w2107 w2128] -> w2099
              tunnel: [w2106 w2127] -> w2098
              tunnel: [w2105 w2126] -> w2096
              tunnel: w2095 -> [w2105 w2117]
              tunnel: [w2104 w2125] -> w2094
              tunnel: w2093 -> [w2104 w2116]
              tunnel: w2092 -> [w2103 w2109]
              tunnel: w2091 -> [w2102 w2108]
              tunnel: [w2103 w2109] -> w2090
              tunnel: [w2102 w2108] -> w2089
              frame False {
              }
              frame True {
                n893 = control-ref of="Elevator Cabin"() -> (w2124:refnum<vi>)
                n894 = property class="Slide (strict)"(reference=w2124) -> ("Top"=w2123:i32)  [unwired: 1 in, 2 out]
                n895 = local read "Floors Schematic"() -> (w2121:T4)
                n896 = Preview Queue Element(queue=w2117, timeout in ms (-1)=1, error in (no error)=w2116) -> (timed out?=w2115:bool)  [unwired: 3 out]
                n897 = Unbundle By Name(w2121) -> ("Floor Position"=w2122:i16[])
                n898 = Decrement(x=7 ("32bit integer")) -> (x-1=w2111:i32)
                n899 = Index Array(array=w2122, index=w2111) -> (element=w2119:i16)
                n900 = To Long Integer(number=w2119) -> (32bit integer=w2120:i32)
                n901 = Not Equal?(x=w2120, y=w2123) -> (x != y?=w2114:bool)
                n902 = Select(t=TRUE, s=w2115, f=w2114) -> (s? t:f=w2112:bool)
                n903 = case shown="False" w2112 {
                  tunnel: w2117 -> [w2130 w2142]
                  tunnel: w2116 -> [w2129 w2141]
                  tunnel: [w2130 w2140] -> w2126
                  tunnel: [w2129 w2139] -> w2125
                  frame True {
                    n904 = local read "Elevator Automate"() -> (w2132:T2)
                    n905 = Bundle By Name(cluster=w2132, "Cancel Delay"=TRUE ("Add to Queue")) -> (w2133:T2)
                    n906 = local write "Elevator Automate"(w2133) -> ()
                  }
                  frame False {
                    n907 = local read "Elevator Automate"() -> (w2146:T2)
                    n908 = Unbundle By Name(w2146) -> ("Elevator Command"=w2145:T1)
                    n909 = Equal?(x=w2145, y=Elevator_Command."Close Doors") -> (x = y?=w2143:bool)
                    n910 = case shown="True" w2143 {
                      tunnel: w2142 -> [w2159 w2174]
                      tunnel: w2141 -> [w2158 w2173]
                      tunnel: [w2157 w2174] -> w2140
                      tunnel: [w2156 w2173] -> w2139
                      tunnel: [FALSE ("Call 12") FALSE ("Call 12")] -> w2134
                      frame True {
                        w2169 = T9 20 items=["Floor Length"=48, "Sum of Floors"=12, "Floor Step in ms"=63, "Elevator Door Step in ms"=30, "Global Wait in ms"=20, "Event Wait in ms"=100] ("Elevator Constants")
                        n911 = local read "Elevator Automate"() -> (w2168:T2)
                        n912 = Flush Queue(queue=w2159, error in (no error)=w2158) -> (queue out=w2155:refnum<queue>, error out=w2154:errorcluster)  [unwired: 1 out]
                        n913 = To Long Integer(number=w2169) -> (32bit integer=w2170:i32)
                        n914 = Preview Queue Element(queue=w2155, timeout in ms (-1)=w2170, error in (no error)=w2154) -> (queue out=w2149:refnum<queue>, timed out?=w2148:bool, error out=w2150:errorcluster)  [unwired: 1 out]
                        n915 = Bundle By Name(cluster=w2168, "Forced Stop"=w2148) -> (w2167:T2)
                        n916 = Enqueue Element(queue=w2149, element=Elevator_Command."Open Doors", error in (no error)=w2150) -> (queue out=w2152:refnum<queue>, error out=w2151:errorcluster)  [unwired: 1 in, 1 out]
                        n917 = local write "Elevator Automate"(w2167) -> ()
                        n918 = Enqueue Element(queue=w2152, element=Elevator_Command."Long Delay", error in (no error)=w2151) -> (queue out=w2166:refnum<queue>, error out=w2165:errorcluster)  [unwired: 1 in, 1 out]
                        n919 = Enqueue Element(queue=w2166, element=Elevator_Command."Close Doors", error in (no error)=w2165) -> (queue out=w2164:refnum<queue>, error out=w2163:errorcluster)  [unwired: 1 in, 1 out]
                        n920 = Enqueue Element(queue=w2164, element=Elevator_Command."Idle", error in (no error)=w2163) -> (queue out=w2157:refnum<queue>, error out=w2156:errorcluster)  [unwired: 1 in, 1 out]
                      }
                      frame False {
                        n921 = Wait (ms)(milliseconds to wait=u32 250) -> ()  [unwired: 1 out]
                      }
                    }
                    n922 = local read "Floors Schematic"() -> (w2138:T4)
                    n923 = local read "Elevator Panel"() -> (w2136:T3)
                    n924 = Bundle By Name(cluster=w2138, "Call 7"=w2134) -> (w2137:T4)
                    n925 = Bundle By Name(cluster=w2136, "Floor 7"=w2134) -> (w2135:T3)
                    n926 = local write "Elevator Panel"(w2135) -> ()
                    n927 = local write "Floors Schematic"(w2137) -> ()
                  }
                }
              }
            }
          }
        }
      }
      event Value Change {
        n928 = event-data() -> ("NewVal"=w2185:bool)  [unwired: 1 in, 5 out]
        n929 = call <vilib>:"Acquire Semaphore.vi"("error in (no error)"=w2180, "semaphore"=w2179) -> ("error out"=w2177:errorcluster, "semaphore out"=w2178:T8)  [unwired: 3 in, 1 out]
        n930 = flat-sequence {
          tunnel: w2189 -> [w2202]
          tunnel: w2188 -> [w2201]
          tunnel: [w2200] -> w2187
          tunnel: [w2199] -> w2186
          tunnel: w2185 -> [w2198]
          tunnel: [w2197] -> w2184
          tunnel: w2183 -> [w2196]
          tunnel: [w2195] -> w2182
          tunnel: w2181 -> [w2194]
          tunnel: w2178 -> [w2193]
          tunnel: w2177 -> [w2192]
          tunnel: [w2191] -> w2176
          tunnel: [w2190] -> w2175
          frame #0 {
            n931 = case shown="True" w2198 {
              tunnel: w2202 -> [w2208 w2229]
              tunnel: w2201 -> [w2207 w2228]
              tunnel: [w2208 w2229] -> w2200
              tunnel: [w2207 w2228] -> w2199
              tunnel: [w2206 w2227] -> w2197
              tunnel: w2196 -> [w2206 w2218]
              tunnel: [w2205 w2226] -> w2195
              tunnel: w2194 -> [w2205 w2217]
              tunnel: w2193 -> [w2204 w2210]
              tunnel: w2192 -> [w2203 w2209]
              tunnel: [w2204 w2210] -> w2191
              tunnel: [w2203 w2209] -> w2190
              frame False {
              }
              frame True {
                n932 = control-ref of="Elevator Cabin"() -> (w2225:refnum<vi>)
                n933 = property class="Slide (strict)"(reference=w2225) -> ("Top"=w2224:i32)  [unwired: 1 in, 2 out]
                n934 = local read "Floors Schematic"() -> (w2222:T4)
                n935 = Preview Queue Element(queue=w2218, timeout in ms (-1)=1, error in (no error)=w2217) -> (timed out?=w2216:bool)  [unwired: 3 out]
                n936 = Unbundle By Name(w2222) -> ("Floor Position"=w2223:i16[])
                n937 = Decrement(x=8 ("32bit integer")) -> (x-1=w2212:i32)
                n938 = Index Array(array=w2223, index=w2212) -> (element=w2220:i16)
                n939 = To Long Integer(number=w2220) -> (32bit integer=w2221:i32)
                n940 = Not Equal?(x=w2221, y=w2224) -> (x != y?=w2215:bool)
                n941 = Select(t=TRUE, s=w2216, f=w2215) -> (s? t:f=w2213:bool)
                n942 = case shown="False" w2213 {
                  tunnel: w2218 -> [w2231 w2243]
                  tunnel: w2217 -> [w2230 w2242]
                  tunnel: [w2231 w2241] -> w2227
                  tunnel: [w2230 w2240] -> w2226
                  frame True {
                    n943 = local read "Elevator Automate"() -> (w2233:T2)
                    n944 = Bundle By Name(cluster=w2233, "Cancel Delay"=TRUE ("Add to Queue")) -> (w2234:T2)
                    n945 = local write "Elevator Automate"(w2234) -> ()
                  }
                  frame False {
                    n946 = local read "Elevator Automate"() -> (w2247:T2)
                    n947 = Unbundle By Name(w2247) -> ("Elevator Command"=w2246:T1)
                    n948 = Equal?(x=w2246, y=Elevator_Command."Close Doors") -> (x = y?=w2244:bool)
                    n949 = case shown="True" w2244 {
                      tunnel: w2243 -> [w2260 w2275]
                      tunnel: w2242 -> [w2259 w2274]
                      tunnel: [w2258 w2275] -> w2241
                      tunnel: [w2257 w2274] -> w2240
                      tunnel: [FALSE ("Call 12") FALSE ("Call 12")] -> w2235
                      frame True {
                        w2270 = T9 20 items=["Floor Length"=48, "Sum of Floors"=12, "Floor Step in ms"=63, "Elevator Door Step in ms"=30, "Global Wait in ms"=20, "Event Wait in ms"=100] ("Elevator Constants")
                        n950 = local read "Elevator Automate"() -> (w2269:T2)
                        n951 = Flush Queue(queue=w2260, error in (no error)=w2259) -> (queue out=w2256:refnum<queue>, error out=w2255:errorcluster)  [unwired: 1 out]
                        n952 = To Long Integer(number=w2270) -> (32bit integer=w2271:i32)
                        n953 = Preview Queue Element(queue=w2256, timeout in ms (-1)=w2271, error in (no error)=w2255) -> (queue out=w2250:refnum<queue>, timed out?=w2249:bool, error out=w2251:errorcluster)  [unwired: 1 out]
                        n954 = Bundle By Name(cluster=w2269, "Forced Stop"=w2249) -> (w2268:T2)
                        n955 = Enqueue Element(queue=w2250, element=Elevator_Command."Open Doors", error in (no error)=w2251) -> (queue out=w2253:refnum<queue>, error out=w2252:errorcluster)  [unwired: 1 in, 1 out]
                        n956 = local write "Elevator Automate"(w2268) -> ()
                        n957 = Enqueue Element(queue=w2253, element=Elevator_Command."Long Delay", error in (no error)=w2252) -> (queue out=w2267:refnum<queue>, error out=w2266:errorcluster)  [unwired: 1 in, 1 out]
                        n958 = Enqueue Element(queue=w2267, element=Elevator_Command."Close Doors", error in (no error)=w2266) -> (queue out=w2265:refnum<queue>, error out=w2264:errorcluster)  [unwired: 1 in, 1 out]
                        n959 = Enqueue Element(queue=w2265, element=Elevator_Command."Idle", error in (no error)=w2264) -> (queue out=w2258:refnum<queue>, error out=w2257:errorcluster)  [unwired: 1 in, 1 out]
                      }
                      frame False {
                        n960 = Wait (ms)(milliseconds to wait=u32 250) -> ()  [unwired: 1 out]
                      }
                    }
                    n961 = local read "Floors Schematic"() -> (w2239:T4)
                    n962 = local read "Elevator Panel"() -> (w2237:T3)
                    n963 = Bundle By Name(cluster=w2239, "Call 8"=w2235) -> (w2238:T4)
                    n964 = Bundle By Name(cluster=w2237, "Floor 8"=w2235) -> (w2236:T3)
                    n965 = local write "Elevator Panel"(w2236) -> ()
                    n966 = local write "Floors Schematic"(w2238) -> ()
                  }
                }
              }
            }
          }
        }
      }
      event Value Change {
        n967 = event-data() -> ("NewVal"=w2286:bool)  [unwired: 1 in, 5 out]
        n968 = call <vilib>:"Acquire Semaphore.vi"("error in (no error)"=w2280, "semaphore"=w2281) -> ("error out"=w2278:errorcluster, "semaphore out"=w2279:T8)  [unwired: 3 in, 1 out]
        n969 = flat-sequence {
          tunnel: w2290 -> [w2303]
          tunnel: w2289 -> [w2302]
          tunnel: [w2301] -> w2288
          tunnel: [w2300] -> w2287
          tunnel: w2286 -> [w2299]
          tunnel: [w2298] -> w2285
          tunnel: w2284 -> [w2297]
          tunnel: [w2296] -> w2283
          tunnel: w2282 -> [w2295]
          tunnel: w2279 -> [w2294]
          tunnel: w2278 -> [w2292]
          tunnel: [w2293] -> w2277
          tunnel: [w2291] -> w2276
          frame #0 {
            n970 = case shown="True" w2299 {
              tunnel: w2303 -> [w2309 w2330]
              tunnel: w2302 -> [w2308 w2329]
              tunnel: [w2309 w2330] -> w2301
              tunnel: [w2308 w2329] -> w2300
              tunnel: [w2307 w2328] -> w2298
              tunnel: w2297 -> [w2307 w2319]
              tunnel: [w2306 w2327] -> w2296
              tunnel: w2295 -> [w2306 w2318]
              tunnel: w2294 -> [w2305 w2311]
              tunnel: [w2305 w2311] -> w2293
              tunnel: w2292 -> [w2304 w2310]
              tunnel: [w2304 w2310] -> w2291
              frame False {
              }
              frame True {
                n971 = control-ref of="Elevator Cabin"() -> (w2326:refnum<vi>)
                n972 = property class="Slide (strict)"(reference=w2326) -> ("Top"=w2325:i32)  [unwired: 1 in, 2 out]
                n973 = local read "Floors Schematic"() -> (w2323:T4)
                n974 = Preview Queue Element(queue=w2319, timeout in ms (-1)=1, error in (no error)=w2318) -> (timed out?=w2317:bool)  [unwired: 3 out]
                n975 = Unbundle By Name(w2323) -> ("Floor Position"=w2324:i16[])
                n976 = Decrement(x=9 ("32bit integer")) -> (x-1=w2313:i32)
                n977 = Index Array(array=w2324, index=w2313) -> (element=w2321:i16)
                n978 = To Long Integer(number=w2321) -> (32bit integer=w2322:i32)
                n979 = Not Equal?(x=w2322, y=w2325) -> (x != y?=w2316:bool)
                n980 = Select(t=TRUE, s=w2317, f=w2316) -> (s? t:f=w2314:bool)
                n981 = case shown="False" w2314 {
                  tunnel: w2319 -> [w2332 w2344]
                  tunnel: w2318 -> [w2331 w2343]
                  tunnel: [w2332 w2342] -> w2328
                  tunnel: [w2331 w2341] -> w2327
                  frame True {
                    n982 = local read "Elevator Automate"() -> (w2334:T2)
                    n983 = Bundle By Name(cluster=w2334, "Cancel Delay"=TRUE ("Add to Queue")) -> (w2335:T2)
                    n984 = local write "Elevator Automate"(w2335) -> ()
                  }
                  frame False {
                    n985 = local read "Elevator Automate"() -> (w2348:T2)
                    n986 = Unbundle By Name(w2348) -> ("Elevator Command"=w2347:T1)
                    n987 = Equal?(x=w2347, y=Elevator_Command."Close Doors") -> (x = y?=w2345:bool)
                    n988 = case shown="True" w2345 {
                      tunnel: w2344 -> [w2361 w2376]
                      tunnel: w2343 -> [w2360 w2375]
                      tunnel: [w2359 w2376] -> w2342
                      tunnel: [w2358 w2375] -> w2341
                      tunnel: [FALSE ("Call 12") FALSE ("Call 12")] -> w2336
                      frame True {
                        w2371 = T9 20 items=["Floor Length"=48, "Sum of Floors"=12, "Floor Step in ms"=63, "Elevator Door Step in ms"=30, "Global Wait in ms"=20, "Event Wait in ms"=100] ("Elevator Constants")
                        n989 = local read "Elevator Automate"() -> (w2370:T2)
                        n990 = Flush Queue(queue=w2361, error in (no error)=w2360) -> (queue out=w2357:refnum<queue>, error out=w2356:errorcluster)  [unwired: 1 out]
                        n991 = To Long Integer(number=w2371) -> (32bit integer=w2372:i32)
                        n992 = Preview Queue Element(queue=w2357, timeout in ms (-1)=w2372, error in (no error)=w2356) -> (queue out=w2351:refnum<queue>, timed out?=w2350:bool, error out=w2352:errorcluster)  [unwired: 1 out]
                        n993 = Bundle By Name(cluster=w2370, "Forced Stop"=w2350) -> (w2369:T2)
                        n994 = Enqueue Element(queue=w2351, element=Elevator_Command."Open Doors", error in (no error)=w2352) -> (queue out=w2354:refnum<queue>, error out=w2353:errorcluster)  [unwired: 1 in, 1 out]
                        n995 = local write "Elevator Automate"(w2369) -> ()
                        n996 = Enqueue Element(queue=w2354, element=Elevator_Command."Long Delay", error in (no error)=w2353) -> (queue out=w2368:refnum<queue>, error out=w2367:errorcluster)  [unwired: 1 in, 1 out]
                        n997 = Enqueue Element(queue=w2368, element=Elevator_Command."Close Doors", error in (no error)=w2367) -> (queue out=w2366:refnum<queue>, error out=w2365:errorcluster)  [unwired: 1 in, 1 out]
                        n998 = Enqueue Element(queue=w2366, element=Elevator_Command."Idle", error in (no error)=w2365) -> (queue out=w2359:refnum<queue>, error out=w2358:errorcluster)  [unwired: 1 in, 1 out]
                      }
                      frame False {
                        n999 = Wait (ms)(milliseconds to wait=u32 250) -> ()  [unwired: 1 out]
                      }
                    }
                    n1000 = local read "Floors Schematic"() -> (w2340:T4)
                    n1001 = local read "Elevator Panel"() -> (w2338:T3)
                    n1002 = Bundle By Name(cluster=w2340, "Call 9"=w2336) -> (w2339:T4)
                    n1003 = Bundle By Name(cluster=w2338, "Floor 9"=w2336) -> (w2337:T3)
                    n1004 = local write "Elevator Panel"(w2337) -> ()
                    n1005 = local write "Floors Schematic"(w2339) -> ()
                  }
                }
              }
            }
          }
        }
      }
      event Value Change {
        n1006 = event-data() -> ("NewVal"=w2387:bool)  [unwired: 1 in, 5 out]
        n1007 = call <vilib>:"Acquire Semaphore.vi"("error in (no error)"=w2381, "semaphore"=w2382) -> ("error out"=w2379:errorcluster, "semaphore out"=w2380:T8)  [unwired: 3 in, 1 out]
        n1008 = flat-sequence {
          tunnel: w2391 -> [w2404]
          tunnel: w2390 -> [w2403]
          tunnel: [w2402] -> w2389
          tunnel: [w2401] -> w2388
          tunnel: w2387 -> [w2400]
          tunnel: [w2399] -> w2386
          tunnel: w2385 -> [w2398]
          tunnel: [w2397] -> w2384
          tunnel: w2383 -> [w2396]
          tunnel: w2380 -> [w2395]
          tunnel: w2379 -> [w2393]
          tunnel: [w2394] -> w2378
          tunnel: [w2392] -> w2377
          frame #0 {
            n1009 = case shown="True" w2400 {
              tunnel: w2404 -> [w2410 w2431]
              tunnel: w2403 -> [w2409 w2430]
              tunnel: [w2410 w2431] -> w2402
              tunnel: [w2409 w2430] -> w2401
              tunnel: [w2408 w2429] -> w2399
              tunnel: w2398 -> [w2408 w2420]
              tunnel: [w2407 w2428] -> w2397
              tunnel: w2396 -> [w2407 w2419]
              tunnel: w2395 -> [w2406 w2412]
              tunnel: [w2406 w2412] -> w2394
              tunnel: w2393 -> [w2405 w2411]
              tunnel: [w2405 w2411] -> w2392
              frame False {
              }
              frame True {
                n1010 = control-ref of="Elevator Cabin"() -> (w2427:refnum<vi>)
                n1011 = property class="Slide (strict)"(reference=w2427) -> ("Top"=w2426:i32)  [unwired: 1 in, 2 out]
                n1012 = local read "Floors Schematic"() -> (w2424:T4)
                n1013 = Preview Queue Element(queue=w2420, timeout in ms (-1)=1, error in (no error)=w2419) -> (timed out?=w2418:bool)  [unwired: 3 out]
                n1014 = Unbundle By Name(w2424) -> ("Floor Position"=w2425:i16[])
                n1015 = Decrement(x=10 ("32bit integer")) -> (x-1=w2414:i32)
                n1016 = Index Array(array=w2425, index=w2414) -> (element=w2422:i16)
                n1017 = To Long Integer(number=w2422) -> (32bit integer=w2423:i32)
                n1018 = Not Equal?(x=w2423, y=w2426) -> (x != y?=w2417:bool)
                n1019 = Select(t=TRUE, s=w2418, f=w2417) -> (s? t:f=w2415:bool)
                n1020 = case shown="False" w2415 {
                  tunnel: w2420 -> [w2433 w2445]
                  tunnel: w2419 -> [w2432 w2444]
                  tunnel: [w2433 w2443] -> w2429
                  tunnel: [w2432 w2442] -> w2428
                  frame True {
                    n1021 = local read "Elevator Automate"() -> (w2435:T2)
                    n1022 = Bundle By Name(cluster=w2435, "Cancel Delay"=TRUE ("Add to Queue")) -> (w2436:T2)
                    n1023 = local write "Elevator Automate"(w2436) -> ()
                  }
                  frame False {
                    n1024 = local read "Elevator Automate"() -> (w2449:T2)
                    n1025 = Unbundle By Name(w2449) -> ("Elevator Command"=w2448:T1)
                    n1026 = Equal?(x=w2448, y=Elevator_Command."Close Doors") -> (x = y?=w2446:bool)
                    n1027 = case shown="True" w2446 {
                      tunnel: w2445 -> [w2462 w2477]
                      tunnel: w2444 -> [w2461 w2476]
                      tunnel: [w2460 w2477] -> w2443
                      tunnel: [w2459 w2476] -> w2442
                      tunnel: [FALSE ("Call 12") FALSE ("Call 12")] -> w2437
                      frame True {
                        w2472 = T9 20 items=["Floor Length"=48, "Sum of Floors"=12, "Floor Step in ms"=63, "Elevator Door Step in ms"=30, "Global Wait in ms"=20, "Event Wait in ms"=100] ("Elevator Constants")
                        n1028 = local read "Elevator Automate"() -> (w2471:T2)
                        n1029 = Flush Queue(queue=w2462, error in (no error)=w2461) -> (queue out=w2458:refnum<queue>, error out=w2457:errorcluster)  [unwired: 1 out]
                        n1030 = To Long Integer(number=w2472) -> (32bit integer=w2473:i32)
                        n1031 = Preview Queue Element(queue=w2458, timeout in ms (-1)=w2473, error in (no error)=w2457) -> (queue out=w2452:refnum<queue>, timed out?=w2451:bool, error out=w2453:errorcluster)  [unwired: 1 out]
                        n1032 = Bundle By Name(cluster=w2471, "Forced Stop"=w2451) -> (w2470:T2)
                        n1033 = Enqueue Element(queue=w2452, element=Elevator_Command."Open Doors", error in (no error)=w2453) -> (queue out=w2455:refnum<queue>, error out=w2454:errorcluster)  [unwired: 1 in, 1 out]
                        n1034 = local write "Elevator Automate"(w2470) -> ()
                        n1035 = Enqueue Element(queue=w2455, element=Elevator_Command."Long Delay", error in (no error)=w2454) -> (queue out=w2469:refnum<queue>, error out=w2468:errorcluster)  [unwired: 1 in, 1 out]
                        n1036 = Enqueue Element(queue=w2469, element=Elevator_Command."Close Doors", error in (no error)=w2468) -> (queue out=w2467:refnum<queue>, error out=w2466:errorcluster)  [unwired: 1 in, 1 out]
                        n1037 = Enqueue Element(queue=w2467, element=Elevator_Command."Idle", error in (no error)=w2466) -> (queue out=w2460:refnum<queue>, error out=w2459:errorcluster)  [unwired: 1 in, 1 out]
                      }
                      frame False {
                        n1038 = Wait (ms)(milliseconds to wait=u32 250) -> ()  [unwired: 1 out]
                      }
                    }
                    n1039 = local read "Floors Schematic"() -> (w2441:T4)
                    n1040 = local read "Elevator Panel"() -> (w2439:T3)
                    n1041 = Bundle By Name(cluster=w2441, "Call 10"=w2437) -> (w2440:T4)
                    n1042 = Bundle By Name(cluster=w2439, "Floor 10"=w2437) -> (w2438:T3)
                    n1043 = local write "Elevator Panel"(w2438) -> ()
                    n1044 = local write "Floors Schematic"(w2440) -> ()
                  }
                }
              }
            }
          }
        }
      }
      event Value Change {
        n1045 = event-data() -> ("NewVal"=w2488:bool)  [unwired: 1 in, 5 out]
        n1046 = call <vilib>:"Acquire Semaphore.vi"("error in (no error)"=w2483, "semaphore"=w2482) -> ("error out"=w2480:errorcluster, "semaphore out"=w2481:T8)  [unwired: 3 in, 1 out]
        n1047 = flat-sequence {
          tunnel: w2492 -> [w2505]
          tunnel: w2491 -> [w2504]
          tunnel: [w2503] -> w2490
          tunnel: [w2502] -> w2489
          tunnel: w2488 -> [w2501]
          tunnel: [w2500] -> w2487
          tunnel: w2486 -> [w2499]
          tunnel: [w2498] -> w2485
          tunnel: w2484 -> [w2497]
          tunnel: w2481 -> [w2495]
          tunnel: w2480 -> [w2494]
          tunnel: [w2496] -> w2479
          tunnel: [w2493] -> w2478
          frame #0 {
            n1048 = case shown="True" w2501 {
              tunnel: w2505 -> [w2511 w2532]
              tunnel: w2504 -> [w2510 w2531]
              tunnel: [w2511 w2532] -> w2503
              tunnel: [w2510 w2531] -> w2502
              tunnel: [w2509 w2530] -> w2500
              tunnel: w2499 -> [w2509 w2521]
              tunnel: [w2508 w2529] -> w2498
              tunnel: w2497 -> [w2508 w2520]
              tunnel: [w2507 w2513] -> w2496
              tunnel: w2495 -> [w2507 w2513]
              tunnel: w2494 -> [w2506 w2512]
              tunnel: [w2506 w2512] -> w2493
              frame False {
              }
              frame True {
                n1049 = control-ref of="Elevator Cabin"() -> (w2528:refnum<vi>)
                n1050 = property class="Slide (strict)"(reference=w2528) -> ("Top"=w2527:i32)  [unwired: 1 in, 2 out]
                n1051 = local read "Floors Schematic"() -> (w2525:T4)
                n1052 = Preview Queue Element(queue=w2521, timeout in ms (-1)=1, error in (no error)=w2520) -> (timed out?=w2519:bool)  [unwired: 3 out]
                n1053 = Unbundle By Name(w2525) -> ("Floor Position"=w2526:i16[])
                n1054 = Decrement(x=11 ("32bit integer")) -> (x-1=w2515:i32)
                n1055 = Index Array(array=w2526, index=w2515) -> (element=w2523:i16)
                n1056 = To Long Integer(number=w2523) -> (32bit integer=w2524:i32)
                n1057 = Not Equal?(x=w2524, y=w2527) -> (x != y?=w2518:bool)
                n1058 = Select(t=TRUE, s=w2519, f=w2518) -> (s? t:f=w2516:bool)
                n1059 = case shown="False" w2516 {
                  tunnel: w2521 -> [w2534 w2546]
                  tunnel: w2520 -> [w2533 w2545]
                  tunnel: [w2534 w2544] -> w2530
                  tunnel: [w2533 w2543] -> w2529
                  frame True {
                    n1060 = local read "Elevator Automate"() -> (w2536:T2)
                    n1061 = Bundle By Name(cluster=w2536, "Cancel Delay"=TRUE ("Add to Queue")) -> (w2537:T2)
                    n1062 = local write "Elevator Automate"(w2537) -> ()
                  }
                  frame False {
                    n1063 = local read "Elevator Automate"() -> (w2550:T2)
                    n1064 = Unbundle By Name(w2550) -> ("Elevator Command"=w2549:T1)
                    n1065 = Equal?(x=w2549, y=Elevator_Command."Close Doors") -> (x = y?=w2547:bool)
                    n1066 = case shown="False" w2547 {
                      tunnel: w2546 -> [w2563 w2578]
                      tunnel: w2545 -> [w2562 w2577]
                      tunnel: [w2561 w2578] -> w2544
                      tunnel: [w2560 w2577] -> w2543
                      tunnel: [FALSE ("Call 12") FALSE ("Call 12")] -> w2538
                      frame True {
                        w2573 = T9 20 items=["Floor Length"=48, "Sum of Floors"=12, "Floor Step in ms"=63, "Elevator Door Step in ms"=30, "Global Wait in ms"=20, "Event Wait in ms"=100] ("Elevator Constants")
                        n1067 = local read "Elevator Automate"() -> (w2572:T2)
                        n1068 = Flush Queue(queue=w2563, error in (no error)=w2562) -> (queue out=w2559:refnum<queue>, error out=w2558:errorcluster)  [unwired: 1 out]
                        n1069 = To Long Integer(number=w2573) -> (32bit integer=w2574:i32)
                        n1070 = Preview Queue Element(queue=w2559, timeout in ms (-1)=w2574, error in (no error)=w2558) -> (queue out=w2553:refnum<queue>, timed out?=w2552:bool, error out=w2554:errorcluster)  [unwired: 1 out]
                        n1071 = Bundle By Name(cluster=w2572, "Forced Stop"=w2552) -> (w2571:T2)
                        n1072 = Enqueue Element(queue=w2553, element=Elevator_Command."Open Doors", error in (no error)=w2554) -> (queue out=w2556:refnum<queue>, error out=w2555:errorcluster)  [unwired: 1 in, 1 out]
                        n1073 = local write "Elevator Automate"(w2571) -> ()
                        n1074 = Enqueue Element(queue=w2556, element=Elevator_Command."Long Delay", error in (no error)=w2555) -> (queue out=w2570:refnum<queue>, error out=w2569:errorcluster)  [unwired: 1 in, 1 out]
                        n1075 = Enqueue Element(queue=w2570, element=Elevator_Command."Close Doors", error in (no error)=w2569) -> (queue out=w2568:refnum<queue>, error out=w2567:errorcluster)  [unwired: 1 in, 1 out]
                        n1076 = Enqueue Element(queue=w2568, element=Elevator_Command."Idle", error in (no error)=w2567) -> (queue out=w2561:refnum<queue>, error out=w2560:errorcluster)  [unwired: 1 in, 1 out]
                      }
                      frame False {
                        n1077 = Wait (ms)(milliseconds to wait=u32 250) -> ()  [unwired: 1 out]
                      }
                    }
                    n1078 = local read "Floors Schematic"() -> (w2542:T4)
                    n1079 = local read "Elevator Panel"() -> (w2540:T3)
                    n1080 = Bundle By Name(cluster=w2542, "Call 11"=w2538) -> (w2541:T4)
                    n1081 = Bundle By Name(cluster=w2540, "Floor 11"=w2538) -> (w2539:T3)
                    n1082 = local write "Elevator Panel"(w2539) -> ()
                    n1083 = local write "Floors Schematic"(w2541) -> ()
                  }
                }
              }
            }
          }
        }
      }
      event Value Change {
        n1084 = event-data() -> ("NewVal"=w2589:bool)  [unwired: 1 in, 5 out]
        n1085 = call <vilib>:"Acquire Semaphore.vi"("error in (no error)"=w2583, "semaphore"=w2584) -> ("error out"=w2580:errorcluster, "semaphore out"=w2582:T8)  [unwired: 3 in, 1 out]
        n1086 = flat-sequence {
          tunnel: w2593 -> [w2606]
          tunnel: w2592 -> [w2605]
          tunnel: [w2604] -> w2591
          tunnel: [w2603] -> w2590
          tunnel: w2589 -> [w2602]
          tunnel: [w2601] -> w2588
          tunnel: w2587 -> [w2600]
          tunnel: [w2599] -> w2586
          tunnel: w2585 -> [w2598]
          tunnel: w2582 -> [w2597]
          tunnel: [w2595] -> w2581
          tunnel: w2580 -> [w2596]
          tunnel: [w2594] -> w2579
          frame #0 {
            n1087 = case shown="True" w2602 {
              tunnel: w2606 -> [w2612 w2633]
              tunnel: w2605 -> [w2611 w2632]
              tunnel: [w2612 w2633] -> w2604
              tunnel: [w2611 w2632] -> w2603
              tunnel: [w2610 w2631] -> w2601
              tunnel: w2600 -> [w2610 w2622]
              tunnel: [w2609 w2630] -> w2599
              tunnel: w2598 -> [w2609 w2621]
              tunnel: w2597 -> [w2608 w2614]
              tunnel: w2596 -> [w2607 w2613]
              tunnel: [w2608 w2614] -> w2595
              tunnel: [w2607 w2613] -> w2594
              frame False {
              }
              frame True {
                n1088 = control-ref of="Elevator Cabin"() -> (w2629:refnum<vi>)
                n1089 = property class="Slide (strict)"(reference=w2629) -> ("Top"=w2628:i32)  [unwired: 1 in, 2 out]
                n1090 = local read "Floors Schematic"() -> (w2626:T4)
                n1091 = Preview Queue Element(queue=w2622, timeout in ms (-1)=1, error in (no error)=w2621) -> (timed out?=w2620:bool)  [unwired: 3 out]
                n1092 = Unbundle By Name(w2626) -> ("Floor Position"=w2627:i16[])
                n1093 = Decrement(x=12 ("32bit integer")) -> (x-1=w2616:i32)
                n1094 = Index Array(array=w2627, index=w2616) -> (element=w2624:i16)
                n1095 = To Long Integer(number=w2624) -> (32bit integer=w2625:i32)
                n1096 = Not Equal?(x=w2625, y=w2628) -> (x != y?=w2619:bool)
                n1097 = Select(t=TRUE, s=w2620, f=w2619) -> (s? t:f=w2617:bool)
                n1098 = case shown="False" w2617 {
                  tunnel: w2622 -> [w2635 w2647]
                  tunnel: w2621 -> [w2634 w2646]
                  tunnel: [w2635 w2645] -> w2631
                  tunnel: [w2634 w2644] -> w2630
                  frame True {
                    n1099 = local read "Elevator Automate"() -> (w2637:T2)
                    n1100 = Bundle By Name(cluster=w2637, "Cancel Delay"=TRUE ("Add to Queue")) -> (w2638:T2)
                    n1101 = local write "Elevator Automate"(w2638) -> ()
                  }
                  frame False {
                    n1102 = local read "Elevator Automate"() -> (w2651:T2)
                    n1103 = Unbundle By Name(w2651) -> ("Elevator Command"=w2650:T1)
                    n1104 = Equal?(x=w2650, y=Elevator_Command."Close Doors") -> (x = y?=w2648:bool)
                    n1105 = case shown="True" w2648 {
                      tunnel: w2647 -> [w2664 w2679]
                      tunnel: w2646 -> [w2663 w2678]
                      tunnel: [w2662 w2679] -> w2645
                      tunnel: [w2661 w2678] -> w2644
                      tunnel: [FALSE ("Call 12") FALSE ("Call 12")] -> w2639
                      frame True {
                        w2674 = T9 20 items=["Floor Length"=48, "Sum of Floors"=12, "Floor Step in ms"=63, "Elevator Door Step in ms"=30, "Global Wait in ms"=20, "Event Wait in ms"=100] ("Elevator Constants")
                        n1106 = local read "Elevator Automate"() -> (w2673:T2)
                        n1107 = Flush Queue(queue=w2664, error in (no error)=w2663) -> (queue out=w2660:refnum<queue>, error out=w2659:errorcluster)  [unwired: 1 out]
                        n1108 = To Long Integer(number=w2674) -> (32bit integer=w2675:i32)
                        n1109 = Preview Queue Element(queue=w2660, timeout in ms (-1)=w2675, error in (no error)=w2659) -> (queue out=w2654:refnum<queue>, timed out?=w2653:bool, error out=w2655:errorcluster)  [unwired: 1 out]
                        n1110 = Bundle By Name(cluster=w2673, "Forced Stop"=w2653) -> (w2672:T2)
                        n1111 = Enqueue Element(queue=w2654, element=Elevator_Command."Open Doors", error in (no error)=w2655) -> (queue out=w2657:refnum<queue>, error out=w2656:errorcluster)  [unwired: 1 in, 1 out]
                        n1112 = local write "Elevator Automate"(w2672) -> ()
                        n1113 = Enqueue Element(queue=w2657, element=Elevator_Command."Long Delay", error in (no error)=w2656) -> (queue out=w2671:refnum<queue>, error out=w2670:errorcluster)  [unwired: 1 in, 1 out]
                        n1114 = Enqueue Element(queue=w2671, element=Elevator_Command."Close Doors", error in (no error)=w2670) -> (queue out=w2669:refnum<queue>, error out=w2668:errorcluster)  [unwired: 1 in, 1 out]
                        n1115 = Enqueue Element(queue=w2669, element=Elevator_Command."Idle", error in (no error)=w2668) -> (queue out=w2662:refnum<queue>, error out=w2661:errorcluster)  [unwired: 1 in, 1 out]
                      }
                      frame False {
                        n1116 = Wait (ms)(milliseconds to wait=u32 250) -> ()  [unwired: 1 out]
                      }
                    }
                    n1117 = local read "Floors Schematic"() -> (w2643:T4)
                    n1118 = local read "Elevator Panel"() -> (w2641:T3)
                    n1119 = Bundle By Name(cluster=w2643, "Call 12"=w2639) -> (w2642:T4)
                    n1120 = Bundle By Name(cluster=w2641, "Floor 12"=w2639) -> (w2640:T3)
                    n1121 = local write "Elevator Panel"(w2640) -> ()
                    n1122 = local write "Floors Schematic"(w2642) -> ()
                  }
                }
              }
            }
          }
        }
      }
      event Value Change {
        n1123 = event-data() -> ("NewVal"=w2694:bool)  [unwired: 1 in, 5 out]
        n1124 = call <vilib>:"Acquire Semaphore.vi"("error in (no error)"=w2687, "semaphore"=w2686) -> ("error out"=w2684:errorcluster, "semaphore out"=w2685:T8)  [unwired: 3 in, 1 out]
        n1125 = flat-sequence {
          tunnel: w2694 -> [w2703]
          tunnel: w2693 -> [w2702]
          tunnel: [w2701] -> w2692
          tunnel: w2691 -> [w2700]
          tunnel: [w2699] -> w2690
          tunnel: w2685 -> [w2698]
          tunnel: w2684 -> [w2697]
          tunnel: [w2696] -> w2683
          tunnel: [w2695] -> w2682
          frame #0 {
            n1126 = case shown="True" w2703 {
              tunnel: [w2707 w2713] -> w2701
              tunnel: [w2706 w2710] -> w2699
              tunnel: w2702 -> [w2707 w2717]
              tunnel: w2700 -> [w2706 w2716]
              tunnel: w2698 -> [w2705 w2709]
              tunnel: w2697 -> [w2704 w2708]
              tunnel: [w2705 w2709] -> w2696
              tunnel: [w2704 w2708] -> w2695
              frame False {
              }
              frame True {
                # "Проверка, что лифт на этаже"
                n1127 = local read "Floors Schematic"() -> (w2723:T4)
                n1128 = local read "Elevator Automate"() -> (w2725:T2)
                n1129 = Unbundle By Name(w2725) -> ("Elevator Command"=w2727:T1)
                n1130 = control-ref of="Elevator Cabin"() -> (w2724:refnum<vi>)
                n1131 = property class="Slide (strict)"(reference=w2724) -> ("Top"=w2721:i32)  [unwired: 1 in, 2 out]
                n1132 = Equal?(x=w2727, y=Elevator_Command."Long Delay") -> (x = y?=w2730:bool)
                n1133 = Equal?(x=w2727, y=Elevator_Command."Idle") -> (x = y?=w2728:bool)
                n1134 = Unbundle By Name(w2723) -> ("Floor Position"=w2722:i16[])
                n1135 = Compound Arithmetic op=OR(w2730, w2728) -> (w2719:bool)
                n1136 = while {
                  tunnel: w2722 -> [w2744]
                  tunnel: w2721 -> [w2742]
                  tunnel: [w2739] -> w2718
                  i -> [w2740]
                  stop <- w2741 stop-if-true
                  n1137 = Index Array(array=w2744, index=w2740) -> (element=w2745:i16)
                  n1138 = To Long Integer(number=w2745) -> (32bit integer=w2743:i32)
                  n1139 = Less Or Equal?(x=w2743, y=w2742) -> (x <= y?=w2741:bool)
                  n1140 = Equal?(x=w2742, y=w2743) -> (x = y?=w2746:bool)
                  n1141 = case shown="True" w2746 {
                    selector: w2746 -> [w2747 w2748]
                    tunnel: [w2747 w2748] -> w2739
                    frame False {
                    }
                    frame True {
                    }
                  }
                }
                n1142 = And(x=w2719, y=w2718) -> (x .and. y?=w2720:bool)
                n1143 = case shown="True" w2720 {
                  tunnel: [w2750 w2757] -> w2714
                  tunnel: [w2749 w2756] -> w2711
                  tunnel: w2725 -> [_ w2755]
                  tunnel: w2717 -> [w2750 w2752]
                  tunnel: w2716 -> [w2749 w2751]
                  frame False {
                  }
                  frame True {
                    n1144 = flat-sequence {
                      tunnel: w2755 -> [w2766]
                      tunnel: [w2764] -> w2754
                      tunnel: [w2763] -> w2753
                      tunnel: w2752 -> [w2762]
                      tunnel: w2751 -> [w2761]
                      tunnel: [w2773] -> w2757
                      tunnel: [w2772] -> w2756
                      tunnel: w2754 -> [w2769]
                      tunnel: w2753 -> [w2768]
                      frame #0 {
                        w2759 = T9 20 items=["Floor Length"=48, "Sum of Floors"=12, "Floor Step in ms"=63, "Elevator Door Step in ms"=30, "Global Wait in ms"=20, "Event Wait in ms"=100] ("Elevator Constants")
                        n1145 = To Long Integer(number=w2759) -> (32bit integer=w2758:i32)
                        n1146 = Preview Queue Element(queue=w2762, timeout in ms (-1)=w2758, error in (no error)=w2761) -> (queue out=w2764:refnum<queue>, timed out?=w2760:bool, error out=w2763:errorcluster)  [unwired: 1 out]
                        n1147 = Not(x=w2760) -> (.not. x?=w2767:bool)
                        n1148 = Bundle By Name(cluster=w2766, "Forced Stop"=w2767) -> (w2765:T2)
                        n1149 = local write "Elevator Automate"(w2765) -> ()
                      }
                      frame #1 {
                        n1150 = Flush Queue(queue=w2769, error in (no error)=w2768) -> (queue out=w2771:refnum<queue>, error out=w2770:errorcluster)  [unwired: 1 out]
                        n1151 = Enqueue Element(queue=w2771, element=Elevator_Command."Close Doors", error in (no error)=w2770) -> (queue out=w2776:refnum<queue>, error out=w2775:errorcluster)  [unwired: 1 in, 1 out]
                        n1152 = Enqueue Element(queue=w2776, element=Elevator_Command."Idle", error in (no error)=w2775) -> (queue out=w2773:refnum<queue>, error out=w2772:errorcluster)  [unwired: 1 in, 1 out]
                      }
                    }
                  }
                }
                n1153 = flat-sequence {
                  tunnel: [w2732] -> w2715
                  tunnel: w2714 -> [w2732]
                  tunnel: [w2731] -> w2712
                  tunnel: w2711 -> [w2731]
                  tunnel: w2715 -> [w2735]
                  tunnel: [w2735] -> w2713
                  tunnel: w2712 -> [w2734]
                  tunnel: [w2734] -> w2710
                  frame #0 {
                    n1154 = Wait (ms)(milliseconds to wait=u32 500) -> ()  [unwired: 1 out]
                  }
                  frame #1 {
                    n1155 = local read "Elevator Panel"() -> (w2738:T3)
                    n1156 = Bundle By Name(cluster=w2738, "Close Doors"=FALSE ("Open Doors")) -> (w2737:T3)
                    n1157 = local write "Elevator Panel"(w2737) -> ()
                  }
                }
              }
            }
          }
        }
        n1158 = call <vilib>:"Release Semaphore.vi"("error in (no error)"=w2682, "semaphore"=w2683) -> ("error out"=w2680:errorcluster, "semaphore out"=w2681:T8)  [unwired: 4 in]
      }
      event Value Change {
        n1159 = event-data() -> ("NewVal"=w2792:bool)  [unwired: 1 in, 5 out]
        n1160 = call <vilib>:"Acquire Semaphore.vi"("error in (no error)"=w2785, "semaphore"=w2784) -> ("error out"=w2782:errorcluster, "semaphore out"=w2783:T8)  [unwired: 3 in, 1 out]
        n1161 = flat-sequence {
          tunnel: w2792 -> [w2799]
          tunnel: w2791 -> [w2798]
          tunnel: w2790 -> [w2797]
          tunnel: [w2796] -> w2789
          tunnel: [w2795] -> w2788
          tunnel: w2783 -> [w2794]
          tunnel: w2782 -> [w2793]
          tunnel: [w2794] -> w2780
          tunnel: [w2793] -> w2779
          frame #0 {
            n1162 = case shown="True" w2799 {
              tunnel: [w2801 w2803] -> w2796
              tunnel: [w2800 w2802] -> w2795
              tunnel: w2798 -> [w2801 w2821]
              tunnel: w2797 -> [w2800 w2820]
              frame False {
              }
              frame True {
                # "Проверка, что лифт не между этажами"
                n1163 = local read "Elevator Automate"() -> (w2819:T2)
                n1164 = Unbundle By Name(w2819) -> ("Elevator Command"=w2817:T1)
                n1165 = Equal?(x=w2817, y=Elevator_Command."Long Delay") -> (x = y?=w2824:bool)
                n1166 = Equal?(x=w2817, y=Elevator_Command."Close Doors") -> (x = y?=w2816:bool)
                n1167 = Equal?(x=w2817, y=Elevator_Command."Idle") -> (x = y?=w2815:bool)
                n1168 = Compound Arithmetic op=OR(w2824, w2816, w2815) -> (w2808:bool)
                n1169 = local read "Floors Schematic"() -> (w2813:T4)
                n1170 = control-ref of="Elevator Cabin"() -> (w2814:refnum<vi>)
                n1171 = property class="Slide (strict)"(reference=w2814) -> ("Top"=w2811:i32)  [unwired: 1 in, 2 out]
                n1172 = Unbundle By Name(w2813) -> ("Floor Position"=w2812:i16[])
                n1173 = while {
                  tunnel: w2812 -> [w2838]
                  tunnel: w2811 -> [w2836]
                  tunnel: [w2833] -> w2809
                  i -> [w2834]
                  stop <- w2835 stop-if-true
                  n1174 = Index Array(array=w2838, index=w2834) -> (element=w2839:i16)
                  n1175 = To Long Integer(number=w2839) -> (32bit integer=w2837:i32)
                  n1176 = Less Or Equal?(x=w2837, y=w2836) -> (x <= y?=w2835:bool)
                  n1177 = Equal?(x=w2836, y=w2837) -> (x = y?=w2840:bool)
                  n1178 = case shown="True" w2840 {
                    selector: w2840 -> [w2841 w2842]
                    tunnel: [w2841 w2842] -> w2833
                    frame False {
                    }
                    frame True {
                    }
                  }
                }
                n1179 = And(x=w2809, y=w2808) -> (x .and. y?=w2810:bool)
                n1180 = case shown="True" w2810 {
                  selector: w2810 -> [_ w2847]
                  tunnel: w2821 -> [w2844 w2850]
                  tunnel: w2820 -> [w2843 w2849]
                  tunnel: [w2844 w2852] -> w2807
                  tunnel: [w2843 w2851] -> w2806
                  tunnel: w2819 -> [_ w2846]
                  frame False {
                  }
                  frame True {
                    n1181 = flat-sequence {
                      tunnel: w2849 -> [w2857]
                      tunnel: w2850 -> [w2858]
                      tunnel: [w2856] -> w2848
                      tunnel: w2847 -> [_]
                      tunnel: w2846 -> [w2861]
                      tunnel: [w2855] -> w2845
                      tunnel: [w2864] -> w2852
                      tunnel: [w2863] -> w2851
                      tunnel: w2848 -> [w2875]
                      tunnel: w2845 -> [w2874]
                      frame #0 {
                        w2860 = T9 20 items=["Floor Length"=48, "Sum of Floors"=12, "Floor Step in ms"=63, "Elevator Door Step in ms"=30, "Global Wait in ms"=20, "Event Wait in ms"=100] ("Elevator Constants")
                        n1182 = To Long Integer(number=w2860) -> (32bit integer=w2854:i32)
                        n1183 = Preview Queue Element(queue=w2858, timeout in ms (-1)=w2854, error in (no error)=w2857) -> (queue out=w2856:refnum<queue>, timed out?=w2853:bool, error out=w2855:errorcluster)  [unwired: 1 out]
                        n1184 = Not(x=w2853) -> (.not. x?=w2859:bool)
                        n1185 = Bundle By Name(cluster=w2861, "Forced Stop"=w2859) -> (w2862:T2)
                        n1186 = local write "Elevator Automate"(w2862) -> ()
                      }
                      frame #1 {
                        n1187 = Flush Queue(queue=w2875, error in (no error)=w2874) -> (queue out=w2877:refnum<queue>, error out=w2876:errorcluster)  [unwired: 1 out]
                        n1188 = Enqueue Element(queue=w2877, element=Elevator_Command."Open Doors", error in (no error)=w2876) -> (queue out=w2866:refnum<queue>, error out=w2865:errorcluster)  [unwired: 1 in, 1 out]
                        n1189 = Enqueue Element(queue=w2866, element=Elevator_Command."Long Delay", error in (no error)=w2865) -> (queue out=w2873:refnum<queue>, error out=w2872:errorcluster)  [unwired: 1 in, 1 out]
                        n1190 = Enqueue Element(queue=w2873, element=Elevator_Command."Close Doors", error in (no error)=w2872) -> (queue out=w2871:refnum<queue>, error out=w2870:errorcluster)  [unwired: 1 in, 1 out]
                        n1191 = Enqueue Element(queue=w2871, element=Elevator_Command."Idle", error in (no error)=w2870) -> (queue out=w2864:refnum<queue>, error out=w2863:errorcluster)  [unwired: 1 in, 1 out]
                      }
                    }
                  }
                }
                n1192 = flat-sequence {
                  tunnel: w2807 -> [w2826]
                  tunnel: w2806 -> [w2825]
                  tunnel: [w2826] -> w2805
                  tunnel: [w2825] -> w2804
                  tunnel: [w2829] -> w2803
                  tunnel: w2805 -> [w2829]
                  tunnel: [w2828] -> w2802
                  tunnel: w2804 -> [w2828]
                  frame #0 {
                    n1193 = Wait (ms)(milliseconds to wait=u32 500) -> ()  [unwired: 1 out]
                  }
                  frame #1 {
                    n1194 = local read "Elevator Panel"() -> (w2832:T3)
                    n1195 = Bundle By Name(cluster=w2832, "Open Doors"=FALSE) -> (w2831:T3)
                    n1196 = local write "Elevator Panel"(w2831) -> ()
                  }
                }
              }
            }
          }
        }
        n1197 = call <vilib>:"Release Semaphore.vi"("error in (no error)"=w2779, "semaphore"=w2780) -> ("error out"=w2781:errorcluster, "semaphore out"=w2778:T8)  [unwired: 4 in]
      }
    }
    n1198 = local read "milliseconds to wait"() -> (w1413:u32)
    n1199 = Wait (ms)(milliseconds to wait=w1413) -> ()  [unwired: 1 out]
    n1200 = local read "STOP"() -> (w1427:bool)
  }
  n1201 = while {
    shift-right: [w2889] -> _
    shift-left: w2 -> [w2891]
    shift-right: [w2888] -> _
    shift-left: w1 -> [w2892]
    tunnel: w11 -> [_]
    tunnel: w10 -> [_]
    tunnel: w4 -> [w2880]
    tunnel: w3 -> [w2879]
    tunnel: [w2885] -> _
    tunnel: [w2884] -> _
    stop <- w2890 stop-if-true
    # "Передача номера первого в очереди\nэтажа в номер этажа, на который нужно приехать в текущий момент времени"
    n1202 = call <vilib>:"Acquire Semaphore.vi"("error in (no error)"=w2879, "semaphore"=w2880) -> ("error out"=w2882:errorcluster, "semaphore out"=w2881:T8)  [unwired: 3 in, 1 out]
    n1203 = local read "milliseconds to wait"() -> (w2883:u32)
    n1204 = flat-sequence {
      tunnel: w2892 -> [w2902]
      tunnel: w2891 -> [w2901]
      tunnel: [w2899] -> w2889
      tunnel: [w2898] -> w2888
      tunnel: [w2896] -> w2887
      tunnel: [w2895] -> w2886
      tunnel: w2882 -> [w2894]
      tunnel: w2881 -> [w2893]
      frame #0 {
        n1205 = local read "Elevator Automate"() -> (w2897:T2)
        n1206 = Unbundle By Name(w2897) -> ("Update Target Floor"=w2900:bool)
        n1207 = case shown="False" w2900 {
          tunnel: w2902 -> [w2905 w2917]
          tunnel: w2901 -> [w2906 w2916]
          tunnel: [w2906 w2915] -> w2899
          tunnel: [w2905 w2914] -> w2898
          tunnel: [w2904 w2910] -> w2896
          tunnel: w2893 -> [w2904 w2910]
          tunnel: w2894 -> [w2903 w2909]
          tunnel: [w2903 w2909] -> w2895
          frame False {
          }
          frame True {
            n1208 = local read "Elevator Automate"() -> (w2907:T2)
            n1209 = Dequeue Element(queue=w2916, error in (no error)=w2917) -> (queue out=w2915:refnum<queue>, element=w2911:u8, error out=w2914:errorcluster)  [unwired: 1 in, 1 out]
            n1210 = Bundle By Name(cluster=w2907, "Target Floor"=w2911, "Update Target Floor"=FALSE) -> (w2913:T2)
            n1211 = local write "Elevator Automate"(w2913) -> ()
            n1212 = Wait (ms)(milliseconds to wait=u32 1) -> ()  [unwired: 1 out]
          }
        }
      }
    }
    n1213 = Wait (ms)(milliseconds to wait=w2883) -> ()  [unwired: 1 out]
    n1214 = local read "STOP"() -> (w2890:bool)
    n1215 = call <vilib>:"Release Semaphore.vi"("error in (no error)"=w2886, "semaphore"=w2887) -> ("error out"=w2884:errorcluster, "semaphore out"=w2885:T8)  [unwired: 4 in]
  }
  n1216 = while {
    shift-right: [w2935] -> _
    shift-left: w8 -> [w2934]
    shift-right: [w2931] -> _
    shift-left: w9 -> [w2933]
    tunnel: w10 -> [_]
    tunnel: w11 -> [_]
    tunnel: w4 -> [w2930]
    tunnel: w3 -> [w2929]
    tunnel: [w2924] -> _
    tunnel: [w2923] -> _
    shift-right: [w2919] -> _
    shift-left: w2 -> [w2921]
    shift-right: [w2918] -> _
    shift-left: w1 -> [w2920]
    stop <- w2932 stop-if-true
    # "Принятие следующего в очереди вызова с добавлением команд управления лифтом в очередь"
    n1217 = call <vilib>:"Acquire Semaphore.vi"("error in (no error)"=w2929, "semaphore"=w2930) -> ("error out"=w2927:errorcluster, "semaphore out"=w2928:T8)  [unwired: 3 in, 1 out]
    n1218 = local read "milliseconds to wait"() -> (w2922:u32)
    n1219 = flat-sequence {
      tunnel: [w2955] -> w2935
      tunnel: w2934 -> [w2945]
      tunnel: w2933 -> [w2946]
      tunnel: w2928 -> [w2953]
      tunnel: w2927 -> [w2952]
      tunnel: [w2954] -> w2931
      tunnel: [w2951] -> w2926
      tunnel: [w2950] -> w2925
      tunnel: w2921 -> [w2938]
      tunnel: w2920 -> [w2937]
      tunnel: [w2942] -> w2919
      tunnel: [w2941] -> w2918
      frame #0 {
        n1220 = local read "Elevator Automate"() -> (w2944:T2)
        n1221 = Unbundle By Name(w2944) -> ("Elevator Command"=w2949:T1)
        n1222 = local read "# elements in Elevator Floor Queue"() -> (w2939:i32)
        n1223 = Equal?(x=w2949, y=Elevator_Command."Idle" ("element")) -> (x = y?=w2948:bool)
        n1224 = Not Equal To 0?(x=w2939) -> (x != 0?=w2936:bool)
        n1225 = And(x=w2948, y=w2936) -> (x .and. y?=w2940:bool)
        n1226 = Bundle By Name(cluster=w2944, "Take a Call"=w2940) -> (w2943:T2)
        n1227 = local write "Elevator Automate"(w2943) -> ()
        n1228 = case shown="False" w2940 {
          tunnel: w2946 -> [w2960 w3005]
          tunnel: w2945 -> [w2961 w3004]
          tunnel: [w2961 w3006] -> w2955
          tunnel: [w2960 w2970] -> w2954
          tunnel: w2953 -> [w2959 w2969]
          tunnel: w2952 -> [w2958 w2968]
          tunnel: [w2959 w2969] -> w2951
          tunnel: [w2958 w2968] -> w2950
          tunnel: w2938 -> [w2957 w2967]
          tunnel: w2937 -> [w2956 w2966]
          tunnel: [w2957 w2964] -> w2942
          tunnel: [w2956 w2963] -> w2941
          frame False {
          }
          frame True {
            n1229 = flat-sequence {
              tunnel: w2967 -> [w3013]
              tunnel: w2966 -> [w3012]
              tunnel: [w3009] -> w2964
              tunnel: [w3008] -> w2963
              tunnel: [w3007] -> w2962
              frame #0 {
                n1230 = Dequeue Element(queue=w3013, error in (no error)=w3012) -> (queue out=w3009:refnum<queue>, element=w3010:u8, error out=w3008:errorcluster)  [unwired: 1 in, 1 out]
                n1231 = local read "Elevator Automate"() -> (w3011:T2)
                n1232 = Bundle By Name(cluster=w3011, "Target Floor"=w3010) -> (w3007:T2)
                n1233 = local write "Elevator Automate"(w3007) -> ()
              }
            }
            n1234 = local read "Floors Schematic"() -> (w2991:T4)
            n1235 = Unbundle By Name(w2962) -> ("Elevator Status"=w2977:T6)
            n1236 = Equal?(x=w2977, y=T10."Stand By") -> (x = y?=w2973:bool)
            n1237 = Unbundle By Name(w2991) -> ("Floor Position"=w2992:i16[])
            n1238 = Unbundle By Name(w2962) -> ("Target Floor"=w2988:u8)
            n1239 = control-ref of="Elevator Cabin"() -> (w2986:refnum<vi>)
            n1240 = Decrement(x=w2988) -> (x-1=w2989:u8)
            n1241 = property class="Slide (strict)"(reference=w2986) -> ("Top"=w2975:i32)  [unwired: 1 in, 2 out]
            n1242 = To Long Integer(number=w2989) -> (32bit integer=w2990:i32)
            n1243 = Index Array(array=w2992, index=w2990) -> (element=w2987:i16)
            n1244 = To Long Integer(number=w2987) -> (32bit integer=w2974:i32)
            n1245 = Greater Or Equal?(x=w2975, y=w2974) -> (x >= y?=w2980:bool)
            n1246 = case shown="True" w2980 {
              tunnel: [Elevator_Command."Going Up" ("element") Elevator_Command."Going Down" ("element")] -> w2978
              frame True {
              }
              frame False {
              }
            }
            n1247 = Enqueue Element(queue=w3005, element=w2978, error in (no error)=w3004) -> (queue out=w3003:refnum<queue>, error out=w3002:errorcluster)  [unwired: 1 in, 1 out]
            n1248 = Equal?(x=w2975, y=w2974) -> (x = y?=w2971:bool)
            n1249 = And(x=w2971, y=w2973) -> (x .and. y?=w2972:bool)
            n1250 = case shown="False" w2972 {
              tunnel: w3003 -> [w3020 w3025]
              tunnel: w3002 -> [w3019 w3024]
              tunnel: [w3020 w3022] -> w2985
              tunnel: [w3019 w3021] -> w2984
              frame True {
              }
              frame False {
                n1251 = Enqueue Element(queue=w3025, element=Elevator_Command."Short Delay", error in (no error)=w3024) -> (queue out=w3022:refnum<queue>, error out=w3021:errorcluster)  [unwired: 1 in, 1 out]
              }
            }
            n1252 = Enqueue Element(queue=w2985, element=Elevator_Command."Unpress Button", error in (no error)=w2984) -> (queue out=w2983:refnum<queue>, error out=w2982:errorcluster)  [unwired: 1 in, 1 out]
            n1253 = Enqueue Element(queue=w2983, element=Elevator_Command."Open Doors", error in (no error)=w2982) -> (queue out=w3000:refnum<queue>, error out=w3001:errorcluster)  [unwired: 1 in, 1 out]
            n1254 = flat-sequence {
              tunnel: w2962 -> [w3014]
              tunnel: [w3014] -> w2965
              tunnel: w2965 -> [w3016]
              frame #0 {
                n1255 = Wait (ms)(milliseconds to wait=u32 2000) -> ()  [unwired: 1 out]
              }
              frame #1 {
                n1256 = Bundle By Name(cluster=w3016, "Take a Call"=FALSE ("Update Target Floor")) -> (w3017:T2)
                n1257 = local write "Elevator Automate"(w3017) -> ()
              }
            }
            n1258 = Enqueue Element(queue=w3000, element=Elevator_Command."Long Delay", error in (no error)=w3001) -> (queue out=w2999:refnum<queue>, error out=w2998:errorcluster)  [unwired: 1 in, 1 out]
            n1259 = Enqueue Element(queue=w2999, element=Elevator_Command."Close Doors", error in (no error)=w2998) -> (queue out=w2995:refnum<queue>, error out=w2994:errorcluster)  [unwired: 1 in, 1 out]
            n1260 = Enqueue Element(queue=w2995, element=Elevator_Command."Idle", error in (no error)=w2994) -> (queue out=w2970:refnum<queue>, error out=w3006:errorcluster)  [unwired: 1 in, 1 out]
          }
        }
      }
    }
    n1261 = Wait (ms)(milliseconds to wait=w2922) -> ()  [unwired: 1 out]
    n1262 = local read "STOP"() -> (w2932:bool)
    n1263 = call <vilib>:"Release Semaphore.vi"("error in (no error)"=w2925, "semaphore"=w2926) -> ("error out"=w2923:errorcluster, "semaphore out"=w2924:T8)  [unwired: 4 in]
  }
  n1264 = while {
    tunnel: w11 -> [_]
    tunnel: w10 -> [_]
    shift-right: [w3042] -> _
    shift-left: w9 -> [w3044]
    shift-right: [w3041] -> _
    shift-left: w8 -> [w3043]
    tunnel: w2 -> [_]
    tunnel: w1 -> [_]
    tunnel: w4 -> [w3036]
    tunnel: w3 -> [w3035]
    tunnel: [w3039] -> _
    tunnel: [w3038] -> _
    stop <- "STOP" stop-if-true
    n1265 = call <vilib>:"Acquire Semaphore.vi"("error in (no error)"=w3035, "semaphore"=w3036) -> ("error out"=w3033:errorcluster, "semaphore out"=w3034:T8)  [unwired: 3 in, 1 out]
    n1266 = flat-sequence {
      tunnel: w3044 -> [w3054]
      tunnel: w3043 -> [w3053]
      tunnel: [w3052] -> w3042
      tunnel: [w3051] -> w3041
      tunnel: [w3050] -> w3040
      tunnel: [w3049] -> w3037
      tunnel: w3034 -> [w3048]
      tunnel: w3033 -> [w3047]
      tunnel: [w3048] -> w3031
      tunnel: [w3047] -> w3032
      tunnel: w3028 -> [w3046]
      frame #0 {
        n1267 = Dequeue Element(queue=w3054, timeout in ms (-1)=w3046, error in (no error)=w3053) -> (queue out=w3052:refnum<queue>, element=w3050:T1, timed out?=w3049:bool, error out=w3051:errorcluster)
      }
    }
    n1268 = call <vilib>:"Release Semaphore.vi"("error in (no error)"=w3032, "semaphore"=w3031) -> ("error out"=w3029:errorcluster, "semaphore out"=w3030:T8)  [unwired: 4 in]
    n1269 = local read "milliseconds to wait"() -> (w3028:u32)
    n1270 = case shown="False" w3037 {
      tunnel: w3040 -> [w3059 _]
      tunnel: w3030 -> [w3058 w3724]
      tunnel: w3029 -> [w3057 w3723]
      tunnel: [w3056 w3724] -> w3039
      tunnel: [w3055 w3723] -> w3038
      frame False {
        n1271 = case shown="\"Idle\", Default" w3059 {
          selector: w3059 -> [w3068 w3101 w3182 w3252 w3292 w3376 w3443 w3507 w3575]
          tunnel: w3058 -> [w3066 w3089 w3170 w3246 w3285 w3369 w3442 w3506 w3573]
          tunnel: w3057 -> [w3067 w3090 w3171 w3245 w3286 w3370 w3441 w3505 w3574]
          tunnel: [w3062 w3098 w3179 w3246 w3271 w3355 w3440 w3504 w3569] -> w3056
          tunnel: [w3063 w3099 w3180 w3245 w3276 w3360 w3439 w3503 w3570] -> w3055
          frame "Idle", Default {
            # "Команда ожидания"
            n1272 = call <vilib>:"Acquire Semaphore.vi"("error in (no error)"=w3067, "semaphore"=w3066) -> ("error out"=w3065:errorcluster, "semaphore out"=w3064:T8)  [unwired: 3 in, 1 out]
            n1273 = flat-sequence {
              tunnel: w3068 -> [w3077]
              tunnel: w3064 -> [w3070]
              tunnel: w3065 -> [w3069]
              tunnel: [w3070] -> w3061
              tunnel: [w3069] -> w3060
              frame #0 {
                n1274 = local read "# elements in Elevator Floor Queue"() -> (w3072:i32)
                n1275 = local read "Elevator Automate"() -> (w3078:T2)
                n1276 = Bundle By Name(cluster=w3078, "Elevator Command"=w3077, "Forced Stop"=FALSE) -> (w3075:T2)
                n1277 = Equal To 0?(x=w3072) -> (x = 0?=w3073:bool)
                n1278 = case shown="True" w3073 {
                  tunnel: w3075 -> [w3079 w3081]
                  tunnel: [w3079 w3080] -> w3074
                  frame False {
                  }
                  frame True {
                    n1279 = Bundle By Name(cluster=w3081, "Elevator Status"=T10."Stand By") -> (w3080:T2)
                  }
                }
                n1280 = local write "Elevator Automate"(w3074) -> ()
                n1281 = Wait (ms)(milliseconds to wait=u32 1) -> ()  [unwired: 1 out]
              }
            }
            n1282 = call <vilib>:"Release Semaphore.vi"("error in (no error)"=w3060, "semaphore"=w3061) -> ("error out"=w3063:errorcluster, "semaphore out"=w3062:T8)  [unwired: 4 in]
          }
          frame "Short Delay" {
            # "Короткая задержка ожидания"
            n1283 = flat-sequence {
              tunnel: w3101 -> [w3122]
              tunnel: [w3122] -> w3091
              tunnel: w3090 -> [w3121]
              tunnel: w3089 -> [w3120]
              tunnel: [w3119] -> w3086
              tunnel: [w3118] -> w3084
              tunnel: w3091 -> [w3125]
              tunnel: [w3124] -> w3087
              tunnel: w3086 -> [w3124]
              tunnel: [w3123] -> w3085
              tunnel: w3084 -> [w3123]
              tunnel: [w3131] -> w3088
              tunnel: w3087 -> [w3130]
              tunnel: w3085 -> [w3129]
              tunnel: [w3128] -> w3083
              frame #0 {
                n1284 = call <vilib>:"Acquire Semaphore.vi"("error in (no error)"=w3121, "semaphore"=w3120) -> ("error out"=w3118:errorcluster, "semaphore out"=w3119:T8)  [unwired: 3 in, 1 out]
              }
              frame #1 {
                n1285 = local read "Elevator Automate"() -> (w3127:T2)
                n1286 = Bundle By Name(cluster=w3127, "Elevator Command"=w3125) -> (w3126:T2)
                n1287 = local write "Elevator Automate"(w3126) -> ()
              }
              frame #2 {
                n1288 = call <vilib>:"Release Semaphore.vi"("error in (no error)"=w3129, "semaphore"=w3130) -> ("error out"=w3128:errorcluster, "semaphore out"=w3131:T8)  [unwired: 4 in]
              }
            }
            n1289 = while {
              tunnel: [w3143] -> w3102
              tunnel: [w3140] -> w3093
              tunnel: [w3139] -> w3092
              tunnel: w3088 -> [w3134]
              tunnel: w3083 -> [w3133]
              i -> [w3144]
              stop <- w3143 stop-if-true
              n1290 = flat-sequence {
                tunnel: w3144 -> [w3149]
                tunnel: [w3149] -> w3141
                tunnel: [w3148] -> w3137
                tunnel: [w3147] -> w3135
                tunnel: w3134 -> [w3146]
                tunnel: w3133 -> [w3145]
                tunnel: [w3152] -> w3142
                tunnel: w3141 -> [w3156]
                tunnel: [w3151] -> w3138
                tunnel: w3137 -> [w3151]
                tunnel: [w3150] -> w3136
                tunnel: w3135 -> [w3150]
                tunnel: [w3163] -> w3143
                tunnel: w3142 -> [w3163]
                tunnel: [w3162] -> w3140
                tunnel: [w3161] -> w3139
                tunnel: w3138 -> [w3160]
                tunnel: w3136 -> [w3159]
                frame #0 {
                  n1291 = call <vilib>:"Acquire Semaphore.vi"("error in (no error)"=w3145, "semaphore"=w3146) -> ("error out"=w3147:errorcluster, "semaphore out"=w3148:T8)  [unwired: 3 in, 1 out]
                }
                frame #1 {
                  n1292 = local read "Elevator Automate"() -> (w3154:T2)
                  n1293 = Unbundle By Name(w3154) -> ("Forced Stop"=w3153:bool)
                  n1294 = Greater Or Equal?(x=w3156, y=2000) -> (x >= y?=w3157:bool)
                  n1295 = local read "STOP"() -> (w3158:bool)
                  n1296 = Compound Arithmetic op=OR(w3153, w3157, w3158) -> (w3152:bool)
                }
                frame #2 {
                  n1297 = call <vilib>:"Release Semaphore.vi"("error in (no error)"=w3159, "semaphore"=w3160) -> ("error out"=w3161:errorcluster, "semaphore out"=w3162:T8)  [unwired: 4 in]
                }
              }
              n1298 = Wait (ms)(milliseconds to wait=u32 1) -> ()  [unwired: 1 out]
            }
            n1299 = flat-sequence {
              tunnel: w3102 -> [w3107]
              tunnel: [w3107] -> w3100
              tunnel: [w3106] -> w3096
              tunnel: [w3105] -> w3094
              tunnel: w3093 -> [w3104]
              tunnel: w3092 -> [w3103]
              tunnel: w3100 -> [w3110]
              tunnel: [w3109] -> w3097
              tunnel: w3096 -> [w3109]
              tunnel: [w3108] -> w3095
              tunnel: w3094 -> [w3108]
              tunnel: [w3117] -> w3099
              tunnel: [w3116] -> w3098
              tunnel: w3097 -> [w3115]
              tunnel: w3095 -> [w3114]
              frame #0 {
                n1300 = call <vilib>:"Acquire Semaphore.vi"("error in (no error)"=w3103, "semaphore"=w3104) -> ("error out"=w3105:errorcluster, "semaphore out"=w3106:T8)  [unwired: 3 in, 1 out]
              }
              frame #1 {
                n1301 = Not(x=w3110) -> (.not. x?=w3111:bool)
                n1302 = local read "Elevator Automate"() -> (w3112:T2)
                n1303 = Bundle By Name(cluster=w3112, "Forced Stop"=w3111) -> (w3113:T2)
                n1304 = local write "Elevator Automate"(w3113) -> ()
              }
              frame #2 {
                n1305 = call <vilib>:"Release Semaphore.vi"("error in (no error)"=w3114, "semaphore"=w3115) -> ("error out"=w3117:errorcluster, "semaphore out"=w3116:T8)  [unwired: 4 in]
              }
            }
          }
          frame "Long Delay" {
            # "Долгая задержка ожидания"
            n1306 = flat-sequence {
              tunnel: w3182 -> [w3203]
              tunnel: [w3203] -> w3172
              tunnel: w3171 -> [w3202]
              tunnel: w3170 -> [w3201]
              tunnel: [w3200] -> w3167
              tunnel: [w3199] -> w3165
              tunnel: w3172 -> [w3206]
              tunnel: [w3205] -> w3168
              tunnel: w3167 -> [w3205]
              tunnel: [w3204] -> w3166
              tunnel: w3165 -> [w3204]
              tunnel: [w3212] -> w3169
              tunnel: w3168 -> [w3211]
              tunnel: w3166 -> [w3210]
              tunnel: [w3209] -> w3164
              frame #0 {
                n1307 = call <vilib>:"Acquire Semaphore.vi"("error in (no error)"=w3202, "semaphore"=w3201) -> ("error out"=w3199:errorcluster, "semaphore out"=w3200:T8)  [unwired: 3 in, 1 out]
              }
              frame #1 {
                n1308 = local read "Elevator Automate"() -> (w3208:T2)
                n1309 = Bundle By Name(cluster=w3208, "Elevator Command"=w3206) -> (w3207:T2)
                n1310 = local write "Elevator Automate"(w3207) -> ()
              }
              frame #2 {
                n1311 = call <vilib>:"Release Semaphore.vi"("error in (no error)"=w3210, "semaphore"=w3211) -> ("error out"=w3209:errorcluster, "semaphore out"=w3212:T8)  [unwired: 4 in]
              }
            }
            n1312 = while {
              tunnel: [w3224] -> w3183
              tunnel: [w3221] -> w3174
              tunnel: [w3220] -> w3173
              tunnel: w3169 -> [w3215]
              tunnel: w3164 -> [w3214]
              i -> [w3225]
              stop <- w3224 stop-if-true
              n1313 = flat-sequence {
                tunnel: w3225 -> [w3230]
                tunnel: [w3230] -> w3222
                tunnel: [w3229] -> w3218
                tunnel: [w3228] -> w3216
                tunnel: w3215 -> [w3227]
                tunnel: w3214 -> [w3226]
                tunnel: [w3233] -> w3223
                tunnel: w3222 -> [w3237]
                tunnel: [w3232] -> w3219
                tunnel: w3218 -> [w3232]
                tunnel: [w3231] -> w3217
                tunnel: w3216 -> [w3231]
                tunnel: [w3244] -> w3224
                tunnel: w3223 -> [w3244]
                tunnel: [w3243] -> w3221
                tunnel: [w3242] -> w3220
                tunnel: w3219 -> [w3241]
                tunnel: w3217 -> [w3240]
                frame #0 {
                  n1314 = call <vilib>:"Acquire Semaphore.vi"("error in (no error)"=w3226, "semaphore"=w3227) -> ("error out"=w3228:errorcluster, "semaphore out"=w3229:T8)  [unwired: 3 in, 1 out]
                }
                frame #1 {
                  n1315 = local read "Elevator Automate"() -> (w3235:T2)
                  n1316 = Unbundle By Name(w3235) -> ("Forced Stop"=w3234:bool)
                  n1317 = Greater Or Equal?(x=w3237, y=6000) -> (x >= y?=w3238:bool)
                  n1318 = local read "STOP"() -> (w3239:bool)
                  n1319 = Compound Arithmetic op=OR(w3234, w3238, w3239) -> (w3233:bool)
                }
                frame #2 {
                  n1320 = call <vilib>:"Release Semaphore.vi"("error in (no error)"=w3240, "semaphore"=w3241) -> ("error out"=w3242:errorcluster, "semaphore out"=w3243:T8)  [unwired: 4 in]
                }
              }
              n1321 = Wait (ms)(milliseconds to wait=u32 1) -> ()  [unwired: 1 out]
            }
            n1322 = flat-sequence {
              tunnel: w3183 -> [w3188]
              tunnel: [w3188] -> w3181
              tunnel: [w3187] -> w3177
              tunnel: [w3186] -> w3175
              tunnel: w3174 -> [w3185]
              tunnel: w3173 -> [w3184]
              tunnel: w3181 -> [w3191]
              tunnel: [w3190] -> w3178
              tunnel: w3177 -> [w3190]
              tunnel: [w3189] -> w3176
              tunnel: w3175 -> [w3189]
              tunnel: [w3198] -> w3180
              tunnel: [w3197] -> w3179
              tunnel: w3178 -> [w3196]
              tunnel: w3176 -> [w3195]
              frame #0 {
                n1323 = call <vilib>:"Acquire Semaphore.vi"("error in (no error)"=w3184, "semaphore"=w3185) -> ("error out"=w3186:errorcluster, "semaphore out"=w3187:T8)  [unwired: 3 in, 1 out]
              }
              frame #1 {
                n1324 = Not(x=w3191) -> (.not. x?=w3192:bool)
                n1325 = local read "Elevator Automate"() -> (w3193:T2)
                n1326 = Bundle By Name(cluster=w3193, "Forced Stop"=w3192) -> (w3194:T2)
                n1327 = local write "Elevator Automate"(w3194) -> ()
              }
              frame #2 {
                n1328 = call <vilib>:"Release Semaphore.vi"("error in (no error)"=w3195, "semaphore"=w3196) -> ("error out"=w3198:errorcluster, "semaphore out"=w3197:T8)  [unwired: 4 in]
              }
            }
          }
          frame "Cancel Delay" {
            # "Задержка в случае отмены вызова"
            n1329 = local read "Elevator Automate"() -> (w3253:T2)
            n1330 = Bundle By Name(cluster=w3253, "Elevator Command"=w3252) -> (w3251:T2)
            n1331 = local write "Elevator Automate"(w3251) -> ()
            n1332 = while {
              tunnel: w3251 -> [_]
              tunnel: [w3254] -> w3247
              i -> [w3265]
              stop <- w3254 stop-if-true
              n1333 = local read "Elevator Automate"() -> (w3263:T2)
              n1334 = Unbundle By Name(w3263) -> ("Elevator Command"=w3259:T1)
              n1335 = local read "Elevator Automate"() -> (w3256:T2)
              n1336 = Equal?(x=w3259, y=Elevator_Command."Going Down") -> (x = y?=w3258:bool)
              n1337 = Equal?(x=w3259, y=Elevator_Command."Going Up" ("element")) -> (x = y?=w3261:bool)
              n1338 = Or(x=w3261, y=w3258) -> (x .or. y?=w3262:bool)
              n1339 = Wait (ms)(milliseconds to wait=u32 1) -> ()  [unwired: 1 out]
              n1340 = case shown="True" w3262 {
                tunnel: [6000 ("y") 15000 ("y")] -> w3264
                frame False {
                }
                frame True {
                }
              }
              n1341 = Unbundle By Name(w3256) -> ("Forced Stop"=w3255:bool)
              n1342 = Greater Or Equal?(x=w3265, y=w3264) -> (x >= y?=w3266:bool)
              n1343 = local read "STOP"() -> (w3268:bool)
              n1344 = Compound Arithmetic op=OR(w3255, w3266, w3268) -> (w3254:bool)
            }
            n1345 = Not(x=w3247) -> (.not. x?=w3248:bool)
            n1346 = local read "Elevator Automate"() -> (w3249:T2)
            n1347 = Bundle By Name(cluster=w3249, "Forced Stop"=w3248) -> (w3250:T2)
            n1348 = local write "Elevator Automate"(w3250) -> ()
          }
          frame "Open Doors" {
            # "Открыть двери лифта"
            n1349 = flat-sequence {
              tunnel: w3292 -> [w3312]
              tunnel: [w3312] -> w3288
              tunnel: w3286 -> [w3311]
              tunnel: w3285 -> [w3310]
              tunnel: [w3309] -> w3283
              tunnel: [w3308] -> w3281
              tunnel: [w3315] -> w3289
              tunnel: w3288 -> [w3316]
              tunnel: [w3314] -> w3284
              tunnel: w3283 -> [w3314]
              tunnel: [w3313] -> w3282
              tunnel: w3281 -> [w3313]
              tunnel: [w3322] -> w3291
              tunnel: w3289 -> [w3322]
              tunnel: w3284 -> [w3321]
              tunnel: w3282 -> [w3320]
              tunnel: [w3319] -> w3280
              tunnel: [w3318] -> w3279
              frame #0 {
                n1350 = call <vilib>:"Acquire Semaphore.vi"("error in (no error)"=w3311, "semaphore"=w3310) -> ("error out"=w3308:errorcluster, "semaphore out"=w3309:T8)  [unwired: 3 in, 1 out]
              }
              frame #1 {
                n1351 = local read "Elevator Automate"() -> (w3317:T2)
                n1352 = Bundle By Name(cluster=w3317, "Elevator Command"=w3316) -> (w3315:T2)
                n1353 = local write "Elevator Automate"(w3315) -> ()
              }
              frame #2 {
                n1354 = call <vilib>:"Release Semaphore.vi"("error in (no error)"=w3320, "semaphore"=w3321) -> ("error out"=w3318:errorcluster, "semaphore out"=w3319:T8)  [unwired: 4 in]
              }
            }
            n1355 = while {
              tunnel: w3291 -> [_]
              tunnel: [w3334] -> w3290
              tunnel: w3280 -> [w3332]
              tunnel: w3279 -> [w3331]
              tunnel: [w3326] -> w3278
              tunnel: [w3325] -> w3277
              stop <- w3334 stop-if-true
              w3323 = T9 30 items=["Floor Length"=48, "Sum of Floors"=12, "Floor Step in ms"=63, "Elevator Door Step in ms"=30, "Global Wait in ms"=20, "Event Wait in ms"=100] ("Elevator Constants")
              n1356 = flat-sequence {
                tunnel: w3332 -> [w3338]
                tunnel: w3331 -> [w3337]
                tunnel: [w3336] -> w3329
                tunnel: [w3335] -> w3327
                tunnel: [w3345] -> w3333
                tunnel: [w3340] -> w3330
                tunnel: w3329 -> [w3340]
                tunnel: [w3339] -> w3328
                tunnel: w3327 -> [w3339]
                tunnel: [w3354] -> w3334
                tunnel: w3333 -> [w3354]
                tunnel: w3330 -> [w3353]
                tunnel: w3328 -> [w3352]
                tunnel: [w3351] -> w3326
                tunnel: [w3350] -> w3325
                frame #0 {
                  n1357 = call <vilib>:"Acquire Semaphore.vi"("error in (no error)"=w3337, "semaphore"=w3338) -> ("error out"=w3335:errorcluster, "semaphore out"=w3336:T8)  [unwired: 3 in, 1 out]
                }
                frame #1 {
                  n1358 = local read "Elevator Cabin"() -> (w3342:T5)
                  n1359 = local read "Elevator Automate"() -> (w3346:T2)
                  n1360 = Unbundle By Name(w3346) -> ("Forced Stop"=w3347:bool)
                  n1361 = Decrement(x=w3342) -> (x-1=w3343:T5)
                  n1362 = Equal?(x=w3342, y=T5 0) -> (x = y?=w3344:bool)
                  n1363 = local read "STOP"() -> (w3348:bool)
                  n1364 = Select(t=w3342, s=w3344, f=w3343) -> (s? t:f=w3341:T5)
                  n1365 = local write "Elevator Cabin"(w3341) -> ()
                  n1366 = Compound Arithmetic op=OR(w3347, w3344, w3348) -> (w3345:bool)
                }
                frame #2 {
                  n1367 = call <vilib>:"Release Semaphore.vi"("error in (no error)"=w3352, "semaphore"=w3353) -> ("error out"=w3350:errorcluster, "semaphore out"=w3351:T8)  [unwired: 4 in]
                }
              }
              n1368 = To Unsigned Long Integer(number=w3323) -> (unsigned 32bit integer=w3324:u32)
              n1369 = Wait (ms)(milliseconds to wait=w3324) -> ()  [unwired: 1 out]
            }
            n1370 = flat-sequence {
              tunnel: w3290 -> [w3297]
              tunnel: [w3297] -> w3287
              tunnel: w3278 -> [w3296]
              tunnel: w3277 -> [w3295]
              tunnel: [w3294] -> w3274
              tunnel: [w3293] -> w3272
              tunnel: w3287 -> [w3300]
              tunnel: [w3299] -> w3275
              tunnel: w3274 -> [w3299]
              tunnel: [w3298] -> w3273
              tunnel: w3272 -> [w3298]
              tunnel: [w3307] -> w3276
              tunnel: w3275 -> [w3306]
              tunnel: w3273 -> [w3305]
              tunnel: [w3304] -> w3271
              frame #0 {
                n1371 = call <vilib>:"Acquire Semaphore.vi"("error in (no error)"=w3295, "semaphore"=w3296) -> ("error out"=w3293:errorcluster, "semaphore out"=w3294:T8)  [unwired: 3 in, 1 out]
              }
              frame #1 {
                n1372 = Not(x=w3300) -> (.not. x?=w3301:bool)
                n1373 = local read "Elevator Automate"() -> (w3302:T2)
                n1374 = Bundle By Name(cluster=w3302, "Forced Stop"=w3301) -> (w3303:T2)
                n1375 = local write "Elevator Automate"(w3303) -> ()
              }
              frame #2 {
                n1376 = call <vilib>:"Release Semaphore.vi"("error in (no error)"=w3305, "semaphore"=w3306) -> ("error out"=w3307:errorcluster, "semaphore out"=w3304:T8)  [unwired: 4 in]
              }
            }
          }
          frame "Close Doors" {
            # "Закрыть двери лифта"
            n1377 = flat-sequence {
              tunnel: w3376 -> [w3396]
              tunnel: [w3396] -> w3372
              tunnel: w3370 -> [w3395]
              tunnel: w3369 -> [w3394]
              tunnel: [w3393] -> w3367
              tunnel: [w3392] -> w3365
              tunnel: [w3399] -> w3373
              tunnel: w3372 -> [w3400]
              tunnel: [w3398] -> w3368
              tunnel: w3367 -> [w3398]
              tunnel: [w3397] -> w3366
              tunnel: w3365 -> [w3397]
              tunnel: [w3406] -> w3375
              tunnel: w3373 -> [w3406]
              tunnel: w3368 -> [w3405]
              tunnel: w3366 -> [w3404]
              tunnel: [w3403] -> w3364
              tunnel: [w3402] -> w3363
              frame #0 {
                n1378 = call <vilib>:"Acquire Semaphore.vi"("error in (no error)"=w3395, "semaphore"=w3394) -> ("error out"=w3392:errorcluster, "semaphore out"=w3393:T8)  [unwired: 3 in, 1 out]
              }
              frame #1 {
                n1379 = local read "Elevator Automate"() -> (w3401:T2)
                n1380 = Bundle By Name(cluster=w3401, "Elevator Command"=w3400) -> (w3399:T2)
                n1381 = local write "Elevator Automate"(w3399) -> ()
              }
              frame #2 {
                n1382 = call <vilib>:"Release Semaphore.vi"("error in (no error)"=w3404, "semaphore"=w3405) -> ("error out"=w3402:errorcluster, "semaphore out"=w3403:T8)  [unwired: 4 in]
              }
            }
            n1383 = while {
              tunnel: w3375 -> [_]
              tunnel: [w3418] -> w3374
              tunnel: w3364 -> [w3416]
              tunnel: w3363 -> [w3415]
              tunnel: [w3410] -> w3362
              tunnel: [w3409] -> w3361
              stop <- w3418 stop-if-true
              w3407 = T9 30 items=["Floor Length"=48, "Sum of Floors"=12, "Floor Step in ms"=63, "Elevator Door Step in ms"=30, "Global Wait in ms"=20, "Event Wait in ms"=100] ("Elevator Constants")
              n1384 = flat-sequence {
                tunnel: w3416 -> [w3422]
                tunnel: w3415 -> [w3421]
                tunnel: [w3420] -> w3413
                tunnel: [w3419] -> w3411
                tunnel: [w3429] -> w3417
                tunnel: [w3424] -> w3414
                tunnel: w3413 -> [w3424]
                tunnel: [w3423] -> w3412
                tunnel: w3411 -> [w3423]
                tunnel: [w3438] -> w3418
                tunnel: w3417 -> [w3438]
                tunnel: w3414 -> [w3437]
                tunnel: w3412 -> [w3436]
                tunnel: [w3435] -> w3410
                tunnel: [w3434] -> w3409
                frame #0 {
                  n1385 = call <vilib>:"Acquire Semaphore.vi"("error in (no error)"=w3421, "semaphore"=w3422) -> ("error out"=w3419:errorcluster, "semaphore out"=w3420:T8)  [unwired: 3 in, 1 out]
                }
                frame #1 {
                  n1386 = local read "Elevator Cabin"() -> (w3426:T5)
                  n1387 = local read "Elevator Automate"() -> (w3430:T2)
                  n1388 = Unbundle By Name(w3430) -> ("Forced Stop"=w3431:bool)
                  n1389 = Increment(x=w3426) -> (x+1=w3427:T5)
                  n1390 = Equal?(x=w3426, y=T5 100) -> (x = y?=w3428:bool)
                  n1391 = local read "STOP"() -> (w3432:bool)
                  n1392 = Select(t=w3426, s=w3428, f=w3427) -> (s? t:f=w3425:T5)
                  n1393 = local write "Elevator Cabin"(w3425) -> ()
                  n1394 = Compound Arithmetic op=OR(w3431, w3428, w3432) -> (w3429:bool)
                }
                frame #2 {
                  n1395 = call <vilib>:"Release Semaphore.vi"("error in (no error)"=w3436, "semaphore"=w3437) -> ("error out"=w3434:errorcluster, "semaphore out"=w3435:T8)  [unwired: 4 in]
                }
              }
              n1396 = To Unsigned Long Integer(number=w3407) -> (unsigned 32bit integer=w3408:u32)
              n1397 = Wait (ms)(milliseconds to wait=w3408) -> ()  [unwired: 1 out]
            }
            n1398 = flat-sequence {
              tunnel: w3374 -> [w3381]
              tunnel: [w3381] -> w3371
              tunnel: w3362 -> [w3380]
              tunnel: w3361 -> [w3379]
              tunnel: [w3378] -> w3358
              tunnel: [w3377] -> w3356
              tunnel: w3371 -> [w3384]
              tunnel: [w3383] -> w3359
              tunnel: w3358 -> [w3383]
              tunnel: [w3382] -> w3357
              tunnel: w3356 -> [w3382]
              tunnel: [w3391] -> w3360
              tunnel: w3359 -> [w3390]
              tunnel: w3357 -> [w3389]
              tunnel: [w3388] -> w3355
              frame #0 {
                n1399 = call <vilib>:"Acquire Semaphore.vi"("error in (no error)"=w3379, "semaphore"=w3380) -> ("error out"=w3377:errorcluster, "semaphore out"=w3378:T8)  [unwired: 3 in, 1 out]
              }
              frame #1 {
                n1400 = Not(x=w3384) -> (.not. x?=w3385:bool)
                n1401 = local read "Elevator Automate"() -> (w3386:T2)
                n1402 = Bundle By Name(cluster=w3386, "Forced Stop"=w3385) -> (w3387:T2)
                n1403 = local write "Elevator Automate"(w3387) -> ()
              }
              frame #2 {
                n1404 = call <vilib>:"Release Semaphore.vi"("error in (no error)"=w3389, "semaphore"=w3390) -> ("error out"=w3391:errorcluster, "semaphore out"=w3388:T8)  [unwired: 4 in]
              }
            }
          }
          frame "Going Down" {
            # "Отправить кабину лифта вниз"
            n1405 = control-ref of="Elevator Cabin"() -> (w3446:refnum<vi>)
            n1406 = property class="Slide (strict)"(reference=w3446) -> (reference out=w3444:refnum<vi>, "Top"=w3445:i32)  [unwired: 1 in, 1 out]
            n1407 = while {
              shift-right: [w3462] -> _
              shift-left: w3445 -> [w3459]
              tunnel: w3444 -> [w3463]
              tunnel: w3443 -> [w3460]
              tunnel: w3442 -> [w3454]
              tunnel: w3441 -> [w3453]
              tunnel: [w3448] -> w3440
              tunnel: [w3447] -> w3439
              stop <- w3461 stop-if-true
              n1408 = flat-sequence {
                tunnel: w3459 -> [w3468]
                tunnel: w3460 -> [w3469]
                tunnel: w3463 -> [w3470]
                tunnel: [w3470] -> w3457
                tunnel: [w3469] -> w3456
                tunnel: [w3468] -> w3455
                tunnel: w3454 -> [w3467]
                tunnel: w3453 -> [w3466]
                tunnel: [w3465] -> w3451
                tunnel: [w3464] -> w3449
                tunnel: [w3482] -> w3461
                tunnel: [w3495] -> w3458
                tunnel: w3457 -> [w3496]
                tunnel: w3456 -> [w3478]
                tunnel: w3455 -> [w3474]
                tunnel: [w3473] -> w3452
                tunnel: w3451 -> [w3473]
                tunnel: [w3472] -> w3450
                tunnel: w3449 -> [w3472]
                tunnel: [w3502] -> w3462
                tunnel: w3458 -> [w3502]
                tunnel: w3452 -> [w3501]
                tunnel: w3450 -> [w3500]
                tunnel: [w3499] -> w3448
                tunnel: [w3498] -> w3447
                frame #0 {
                  n1409 = call <vilib>:"Acquire Semaphore.vi"("error in (no error)"=w3466, "semaphore"=w3467) -> ("error out"=w3464:errorcluster, "semaphore out"=w3465:T8)  [unwired: 3 in, 1 out]
                }
                frame #1 {
                  w3475 = T9 40 items=["Floor Length"=48, "Sum of Floors"=12, "Floor Step in ms"=40, "Elevator Door Step in ms"=30, "Global Wait in ms"=20, "Event Wait in ms"=100] ("Elevator Constants")
                  n1410 = local read "Elevator Automate"() -> (w3471:T2)
                  n1411 = local read "Floors Schematic"() -> (w3491:T4)
                  n1412 = Unbundle By Name(w3491) -> ("Floor Position"=w3490:i16[])
                  n1413 = Unbundle By Name(w3471) -> ("Target Floor"=w3488:u8)
                  n1414 = property class="Slide (strict)"(reference=w3496, "Top"=w3474) -> ()  [unwired: 1 in, 2 out]
                  n1415 = Unbundle By Name(w3471) -> ("Forced Stop"=w3476:bool)
                  n1416 = Decrement(x=w3488) -> (x-1=w3486:u8)
                  n1417 = To Long Integer(number=w3486) -> (32bit integer=w3487:i32)
                  n1418 = Index Array(array=w3490, index=w3487) -> (element=w3489:i16)
                  n1419 = To Unsigned Long Integer(number=w3475) -> (unsigned 32bit integer=w3494:u32)
                  n1420 = To Long Integer(number=w3489) -> (32bit integer=w3497:i32)
                  n1421 = Wait (ms)(milliseconds to wait=w3494) -> ()  [unwired: 1 out]
                  n1422 = Increment(x=w3474) -> (x+1=w3495:i32)
                  n1423 = Equal?(x=w3474, y=w3497) -> (x = y?=w3493:bool)
                  n1424 = local read "STOP"() -> (w3492:bool)
                  n1425 = Compound Arithmetic op=OR(w3476, w3493, w3492) -> (w3482:bool)
                  n1426 = Select(t=Elevator_Command."Idle" ("Elevator Command"), s=w3476, f=w3478) -> (s? t:f=w3480:T1)
                  n1427 = Select(t=T10."Stop" ("Elevator Status"), s=w3482, f=T10."Going Down") -> (s? t:f=w3483:T10)
                  n1428 = Bundle By Name(cluster=w3471, "Elevator Status"=w3483) -> (w3477:T2)
                  n1429 = Bundle By Name(cluster=w3477, "Elevator Command"=w3480) -> (w3481:T2)
                  n1430 = local write "Elevator Automate"(w3481) -> ()
                }
                frame #2 {
                  n1431 = call <vilib>:"Release Semaphore.vi"("error in (no error)"=w3500, "semaphore"=w3501) -> ("error out"=w3498:errorcluster, "semaphore out"=w3499:T8)  [unwired: 4 in]
                }
              }
            }
          }
          frame "Going Up" {
            # "Отправить кабину лифта наверх"
            n1432 = control-ref of="Elevator Cabin"() -> (w3510:refnum<vi>)
            n1433 = property class="Slide (strict)"(reference=w3510) -> (reference out=w3508:refnum<vi>, "Top"=w3509:i32)  [unwired: 1 in, 1 out]
            n1434 = while {
              shift-right: [w3526] -> _
              shift-left: w3509 -> [w3523]
              tunnel: w3508 -> [w3527]
              tunnel: w3507 -> [w3525]
              tunnel: w3506 -> [w3518]
              tunnel: w3505 -> [w3517]
              tunnel: [w3512] -> w3504
              tunnel: [w3511] -> w3503
              stop <- w3524 stop-if-true
              n1435 = flat-sequence {
                tunnel: w3523 -> [w3532]
                tunnel: w3525 -> [w3533]
                tunnel: w3527 -> [w3534]
                tunnel: [w3534] -> w3522
                tunnel: [w3533] -> w3521
                tunnel: [w3532] -> w3520
                tunnel: w3518 -> [w3531]
                tunnel: w3517 -> [w3530]
                tunnel: [w3529] -> w3515
                tunnel: [w3528] -> w3513
                tunnel: [w3542] -> w3524
                tunnel: w3522 -> [w3560]
                tunnel: w3521 -> [w3543]
                tunnel: w3520 -> [w3538]
                tunnel: [w3559] -> w3519
                tunnel: [w3536] -> w3516
                tunnel: w3515 -> [w3536]
                tunnel: [w3535] -> w3514
                tunnel: w3513 -> [w3535]
                tunnel: [w3566] -> w3526
                tunnel: w3519 -> [w3566]
                tunnel: w3516 -> [w3565]
                tunnel: w3514 -> [w3564]
                tunnel: [w3563] -> w3512
                tunnel: [w3562] -> w3511
                frame #0 {
                  n1436 = call <vilib>:"Acquire Semaphore.vi"("error in (no error)"=w3530, "semaphore"=w3531) -> ("error out"=w3528:errorcluster, "semaphore out"=w3529:T8)  [unwired: 3 in, 1 out]
                }
                frame #1 {
                  w3539 = T9 40 items=["Floor Length"=48, "Sum of Floors"=12, "Floor Step in ms"=40, "Elevator Door Step in ms"=30, "Global Wait in ms"=20, "Event Wait in ms"=100] ("Elevator Constants")
                  n1437 = local read "Floors Schematic"() -> (w3556:T4)
                  n1438 = local read "Elevator Automate"() -> (w3537:T2)
                  n1439 = Unbundle By Name(w3556) -> ("Floor Position"=w3555:i16[])
                  n1440 = Unbundle By Name(w3537) -> ("Target Floor"=w3553:u8)
                  n1441 = property class="Slide (strict)"(reference=w3560, "Top"=w3538) -> ()  [unwired: 1 in, 2 out]
                  n1442 = Decrement(x=w3553) -> (x-1=w3551:u8)
                  n1443 = To Long Integer(number=w3551) -> (32bit integer=w3552:i32)
                  n1444 = To Unsigned Long Integer(number=w3539) -> (unsigned 32bit integer=w3550:u32)
                  n1445 = Unbundle By Name(w3537) -> ("Forced Stop"=w3540:bool)
                  n1446 = Index Array(array=w3555, index=w3552) -> (element=w3554:i16)
                  n1447 = Wait (ms)(milliseconds to wait=w3550) -> ()  [unwired: 1 out]
                  n1448 = To Long Integer(number=w3554) -> (32bit integer=w3561:i32)
                  n1449 = Decrement(x=w3538) -> (x-1=w3559:i32)
                  n1450 = Equal?(x=w3538, y=w3561) -> (x = y?=w3558:bool)
                  n1451 = local read "STOP"() -> (w3557:bool)
                  n1452 = Select(t=Elevator_Command."Idle", s=w3540, f=w3543) -> (s? t:f=w3545:T1)
                  n1453 = Compound Arithmetic op=OR(w3540, w3558, w3557) -> (w3542:bool)
                  n1454 = Select(t=T10."Stop" ("Elevator Status"), s=w3542, f=T10."Going Up" ("Elevator Status")) -> (s? t:f=w3547:T10)
                  n1455 = Bundle By Name(cluster=w3537, "Elevator Status"=w3547) -> (w3541:T2)
                  n1456 = Bundle By Name(cluster=w3541, "Elevator Command"=w3545) -> (w3546:T2)
                  n1457 = local write "Elevator Automate"(w3546) -> ()
                }
                frame #2 {
                  n1458 = call <vilib>:"Release Semaphore.vi"("error in (no error)"=w3564, "semaphore"=w3565) -> ("error out"=w3562:errorcluster, "semaphore out"=w3563:T8)  [unwired: 4 in]
                }
              }
            }
          }
          frame "Unpress Button" {
            n1459 = call <vilib>:"Acquire Semaphore.vi"("error in (no error)"=w3574, "semaphore"=w3573) -> ("error out"=w3572:errorcluster, "semaphore out"=w3571:T8)  [unwired: 3 in, 1 out]
            n1460 = flat-sequence {
              tunnel: w3575 -> [w3590]
              tunnel: w3571 -> [w3577]
              tunnel: w3572 -> [w3576]
              tunnel: [w3577] -> w3568
              tunnel: [w3576] -> w3567
              frame #0 {
                # "Отжать кнопку на этаже дома и кнопку в кабине"
                n1461 = local read "Elevator Automate"() -> (w3578:T2)
                n1462 = Unbundle By Name(w3578) -> ("Target Floor"=w3582:u8)
                n1463 = Unbundle By Name(w3578) -> ("Elevator Panel Array"=w3585:bool[])
                n1464 = Decrement(x=w3582) -> (x-1=w3591:u8)
                n1465 = To Long Integer(number=w3591) -> (32bit integer=w3583:i32)
                n1466 = Replace Array Subset(array=w3585, new element=FALSE ("new element/subarray"), index=w3583) -> (w3586:bool[])
                n1467 = Bundle By Name(cluster=w3578, "Elevator Panel Array"=w3586) -> (w3581:T2)
                n1468 = Unbundle By Name(w3581) -> ("Floor Array"=w3589:bool[])
                n1469 = Replace Array Subset(array=w3589, new element=FALSE ("new element/subarray"), index=w3583) -> (w3587:bool[])
                n1470 = Bundle By Name(cluster=w3581, "Floor Array"=w3587) -> (w3580:T2)
                n1471 = Bundle By Name(cluster=w3580, "Elevator Command"=w3590) -> (w3579:T2)
                n1472 = local write "Elevator Automate"(w3579) -> ()
                n1473 = case shown="11" w3582 {
                  tunnel: w3579 -> [_ _ _ _ _ _ _ _ _ _ _ _]
                  frame 1, Default {
                    n1474 = local read "Floors Schematic"() -> (w3665:T4)
                    n1475 = Bundle By Name(cluster=w3665, "Call 1"=FALSE ("Call 12")) -> (w3663:T4)
                    n1476 = control-ref of="Call 1"() -> (w3667:refnum<vi>)
                    n1477 = local write "Floors Schematic"(w3663) -> ()
                    n1478 = property class="Bool (strict)"(reference=w3667, "DisabledEnum"=T7."Enabled" ("Disabled")) -> ()  [unwired: 1 in, 2 out]
                  }
                  frame 2 {
                    n1479 = local read "Floors Schematic"() -> (w3670:T4)
                    n1480 = Bundle By Name(cluster=w3670, "Call 2"=FALSE ("Call 12")) -> (w3668:T4)
                    n1481 = control-ref of="Call 2"() -> (w3672:refnum<vi>)
                    n1482 = local write "Floors Schematic"(w3668) -> ()
                    n1483 = property class="Bool (strict)"(reference=w3672, "DisabledEnum"=T7."Enabled" ("Disabled")) -> ()  [unwired: 1 in, 2 out]
                  }
                  frame 3 {
                    n1484 = local read "Floors Schematic"() -> (w3675:T4)
                    n1485 = Bundle By Name(cluster=w3675, "Call 3"=FALSE ("Call 12")) -> (w3673:T4)
                    n1486 = control-ref of="Call 3"() -> (w3677:refnum<vi>)
                    n1487 = local write "Floors Schematic"(w3673) -> ()
                    n1488 = property class="Bool (strict)"(reference=w3677, "DisabledEnum"=T7."Enabled" ("Disabled")) -> ()  [unwired: 1 in, 2 out]
                  }
                  frame 4 {
                    n1489 = local read "Floors Schematic"() -> (w3680:T4)
                    n1490 = Bundle By Name(cluster=w3680, "Call 4"=FALSE ("Call 12")) -> (w3678:T4)
                    n1491 = control-ref of="Call 4"() -> (w3682:refnum<vi>)
                    n1492 = local write "Floors Schematic"(w3678) -> ()
                    n1493 = property class="Bool (strict)"(reference=w3682, "DisabledEnum"=T7."Enabled" ("Disabled")) -> ()  [unwired: 1 in, 2 out]
                  }
                  frame 5 {
                    n1494 = local read "Floors Schematic"() -> (w3685:T4)
                    n1495 = Bundle By Name(cluster=w3685, "Call 5"=FALSE ("Call 12")) -> (w3683:T4)
                    n1496 = control-ref of="Call 5"() -> (w3687:refnum<vi>)
                    n1497 = local write "Floors Schematic"(w3683) -> ()
                    n1498 = property class="Bool (strict)"(reference=w3687, "DisabledEnum"=T7."Enabled" ("Disabled")) -> ()  [unwired: 1 in, 2 out]
                  }
                  frame 6 {
                    n1499 = local read "Floors Schematic"() -> (w3690:T4)
                    n1500 = Bundle By Name(cluster=w3690, "Call 6"=FALSE ("Call 12")) -> (w3688:T4)
                    n1501 = control-ref of="Call 6"() -> (w3692:refnum<vi>)
                    n1502 = local write "Floors Schematic"(w3688) -> ()
                    n1503 = property class="Bool (strict)"(reference=w3692, "DisabledEnum"=T7."Enabled" ("Disabled")) -> ()  [unwired: 1 in, 2 out]
                  }
                  frame 7 {
                    n1504 = local read "Floors Schematic"() -> (w3695:T4)
                    n1505 = Bundle By Name(cluster=w3695, "Call 7"=FALSE ("Call 12")) -> (w3693:T4)
                    n1506 = control-ref of="Call 7"() -> (w3697:refnum<vi>)
                    n1507 = local write "Floors Schematic"(w3693) -> ()
                    n1508 = property class="Bool (strict)"(reference=w3697, "DisabledEnum"=T7."Enabled" ("Disabled")) -> ()  [unwired: 1 in, 2 out]
                  }
                  frame 8 {
                    n1509 = local read "Floors Schematic"() -> (w3700:T4)
                    n1510 = Bundle By Name(cluster=w3700, "Call 8"=FALSE ("Call 12")) -> (w3698:T4)
                    n1511 = control-ref of="Call 8"() -> (w3702:refnum<vi>)
                    n1512 = local write "Floors Schematic"(w3698) -> ()
                    n1513 = property class="Bool (strict)"(reference=w3702, "DisabledEnum"=T7."Enabled" ("Disabled")) -> ()  [unwired: 1 in, 2 out]
                  }
                  frame 9 {
                    n1514 = local read "Floors Schematic"() -> (w3705:T4)
                    n1515 = Bundle By Name(cluster=w3705, "Call 9"=FALSE ("Call 12")) -> (w3703:T4)
                    n1516 = control-ref of="Call 9"() -> (w3707:refnum<vi>)
                    n1517 = local write "Floors Schematic"(w3703) -> ()
                    n1518 = property class="Bool (strict)"(reference=w3707, "DisabledEnum"=T7."Enabled" ("Disabled")) -> ()  [unwired: 1 in, 2 out]
                  }
                  frame 10 {
                    n1519 = local read "Floors Schematic"() -> (w3710:T4)
                    n1520 = Bundle By Name(cluster=w3710, "Call 10"=FALSE ("Call 12")) -> (w3708:T4)
                    n1521 = control-ref of="Call 10"() -> (w3712:refnum<vi>)
                    n1522 = local write "Floors Schematic"(w3708) -> ()
                    n1523 = property class="Bool (strict)"(reference=w3712, "DisabledEnum"=T7."Enabled" ("Disabled")) -> ()  [unwired: 1 in, 2 out]
                  }
                  frame 11 {
                    n1524 = local read "Floors Schematic"() -> (w3715:T4)
                    n1525 = Bundle By Name(cluster=w3715, "Call 11"=FALSE ("Call 12")) -> (w3713:T4)
                    n1526 = control-ref of="Call 11"() -> (w3717:refnum<vi>)
                    n1527 = local write "Floors Schematic"(w3713) -> ()
                    n1528 = property class="Bool (strict)"(reference=w3717, "DisabledEnum"=T7."Enabled" ("Disabled")) -> ()  [unwired: 1 in, 2 out]
                  }
                  frame 12 {
                    n1529 = local read "Floors Schematic"() -> (w3720:T4)
                    n1530 = Bundle By Name(cluster=w3720, "Call 12"=FALSE) -> (w3718:T4)
                    n1531 = control-ref of="Call 12"() -> (w3722:refnum<vi>)
                    n1532 = local write "Floors Schematic"(w3718) -> ()
                    n1533 = property class="Bool (strict)"(reference=w3722, "DisabledEnum"=T7."Enabled" ("Disabled")) -> ()  [unwired: 1 in, 2 out]
                  }
                }
                n1534 = case shown="12" w3582 {
                  tunnel: w3579 -> [_ _ _ _ _ _ _ _ _ _ _ _]
                  frame 1, Default {
                    n1535 = local read "Elevator Panel"() -> (w3595:T3)
                    n1536 = Wait (ms)(milliseconds to wait=u32 1) -> ()  [unwired: 1 out]
                    n1537 = Bundle By Name(cluster=w3595, "Floor 1"=FALSE ("Call 12")) -> (w3593:T3)
                    n1538 = control-ref of="Floor 1"() -> (w3597:refnum<vi>)
                    n1539 = local write "Elevator Panel"(w3593) -> ()
                    n1540 = property class="Bool (strict)"(reference=w3597, "DisabledEnum"=T7."Enabled" ("Disabled")) -> ()  [unwired: 1 in, 2 out]
                  }
                  frame 2 {
                    n1541 = local read "Elevator Panel"() -> (w3601:T3)
                    n1542 = Wait (ms)(milliseconds to wait=u32 1) -> ()  [unwired: 1 out]
                    n1543 = Bundle By Name(cluster=w3601, "Floor 2"=FALSE ("Call 12")) -> (w3599:T3)
                    n1544 = control-ref of="Floor 2"() -> (w3603:refnum<vi>)
                    n1545 = local write "Elevator Panel"(w3599) -> ()
                    n1546 = property class="Bool (strict)"(reference=w3603, "DisabledEnum"=T7."Enabled" ("Disabled")) -> ()  [unwired: 1 in, 2 out]
                  }
                  frame 3 {
                    n1547 = local read "Elevator Panel"() -> (w3607:T3)
                    n1548 = Wait (ms)(milliseconds to wait=u32 1) -> ()  [unwired: 1 out]
                    n1549 = Bundle By Name(cluster=w3607, "Floor 3"=FALSE ("Call 12")) -> (w3605:T3)
                    n1550 = control-ref of="Floor 3"() -> (w3609:refnum<vi>)
                    n1551 = local write "Elevator Panel"(w3605) -> ()
                    n1552 = property class="Bool (strict)"(reference=w3609, "DisabledEnum"=T7."Enabled" ("Disabled")) -> ()  [unwired: 1 in, 2 out]
                  }
                  frame 4 {
                    n1553 = Wait (ms)(milliseconds to wait=u32 1) -> ()  [unwired: 1 out]
                    n1554 = local read "Elevator Panel"() -> (w3613:T3)
                    n1555 = Bundle By Name(cluster=w3613, "Floor 4"=FALSE ("Call 12")) -> (w3611:T3)
                    n1556 = control-ref of="Floor 4"() -> (w3615:refnum<vi>)
                    n1557 = local write "Elevator Panel"(w3611) -> ()
                    n1558 = property class="Bool (strict)"(reference=w3615, "DisabledEnum"=T7."Enabled" ("Disabled")) -> ()  [unwired: 1 in, 2 out]
                  }
                  frame 5 {
                    n1559 = Wait (ms)(milliseconds to wait=u32 1) -> ()  [unwired: 1 out]
                    n1560 = local read "Elevator Panel"() -> (w3619:T3)
                    n1561 = Bundle By Name(cluster=w3619, "Floor 5"=FALSE ("Call 12")) -> (w3617:T3)
                    n1562 = control-ref of="Floor 5"() -> (w3621:refnum<vi>)
                    n1563 = local write "Elevator Panel"(w3617) -> ()
                    n1564 = property class="Bool (strict)"(reference=w3621, "DisabledEnum"=T7."Enabled" ("Disabled")) -> ()  [unwired: 1 in, 2 out]
                  }
                  frame 6 {
                    n1565 = local read "Elevator Panel"() -> (w3625:T3)
                    n1566 = Wait (ms)(milliseconds to wait=u32 1) -> ()  [unwired: 1 out]
                    n1567 = Bundle By Name(cluster=w3625, "Floor 6"=FALSE ("Call 12")) -> (w3623:T3)
                    n1568 = control-ref of="Floor 6"() -> (w3627:refnum<vi>)
                    n1569 = local write "Elevator Panel"(w3623) -> ()
                    n1570 = property class="Bool (strict)"(reference=w3627, "DisabledEnum"=T7."Enabled" ("Disabled")) -> ()  [unwired: 1 in, 2 out]
                  }
                  frame 7 {
                    n1571 = Wait (ms)(milliseconds to wait=u32 1) -> ()  [unwired: 1 out]
                    n1572 = local read "Elevator Panel"() -> (w3631:T3)
                    n1573 = Bundle By Name(cluster=w3631, "Floor 7"=FALSE ("Call 12")) -> (w3629:T3)
                    n1574 = control-ref of="Floor 7"() -> (w3633:refnum<vi>)
                    n1575 = local write "Elevator Panel"(w3629) -> ()
                    n1576 = property class="Bool (strict)"(reference=w3633, "DisabledEnum"=T7."Enabled" ("Disabled")) -> ()  [unwired: 1 in, 2 out]
                  }
                  frame 8 {
                    n1577 = Wait (ms)(milliseconds to wait=u32 1) -> ()  [unwired: 1 out]
                    n1578 = local read "Elevator Panel"() -> (w3637:T3)
                    n1579 = Bundle By Name(cluster=w3637, "Floor 8"=FALSE ("Call 12")) -> (w3635:T3)
                    n1580 = control-ref of="Floor 8"() -> (w3639:refnum<vi>)
                    n1581 = local write "Elevator Panel"(w3635) -> ()
                    n1582 = property class="Bool (strict)"(reference=w3639, "DisabledEnum"=T7."Enabled" ("Disabled")) -> ()  [unwired: 1 in, 2 out]
                  }
                  frame 9 {
                    n1583 = Wait (ms)(milliseconds to wait=u32 1) -> ()  [unwired: 1 out]
                    n1584 = local read "Elevator Panel"() -> (w3643:T3)
                    n1585 = Bundle By Name(cluster=w3643, "Floor 9"=FALSE ("Call 12")) -> (w3641:T3)
                    n1586 = control-ref of="Floor 9"() -> (w3645:refnum<vi>)
                    n1587 = local write "Elevator Panel"(w3641) -> ()
                    n1588 = property class="Bool (strict)"(reference=w3645, "DisabledEnum"=T7."Enabled" ("Disabled")) -> ()  [unwired: 1 in, 2 out]
                  }
                  frame 10 {
                    n1589 = Wait (ms)(milliseconds to wait=u32 1) -> ()  [unwired: 1 out]
                    n1590 = local read "Elevator Panel"() -> (w3649:T3)
                    n1591 = Bundle By Name(cluster=w3649, "Floor 10"=FALSE ("Call 12")) -> (w3647:T3)
                    n1592 = control-ref of="Floor 10"() -> (w3651:refnum<vi>)
                    n1593 = local write "Elevator Panel"(w3647) -> ()
                    n1594 = property class="Bool (strict)"(reference=w3651, "DisabledEnum"=T7."Enabled" ("Disabled")) -> ()  [unwired: 1 in, 2 out]
                  }
                  frame 11 {
                    n1595 = Wait (ms)(milliseconds to wait=u32 1) -> ()  [unwired: 1 out]
                    n1596 = local read "Elevator Panel"() -> (w3655:T3)
                    n1597 = Bundle By Name(cluster=w3655, "Floor 11"=FALSE ("Call 12")) -> (w3653:T3)
                    n1598 = control-ref of="Floor 11"() -> (w3657:refnum<vi>)
                    n1599 = local write "Elevator Panel"(w3653) -> ()
                    n1600 = property class="Bool (strict)"(reference=w3657, "DisabledEnum"=T7."Enabled" ("Disabled")) -> ()  [unwired: 1 in, 2 out]
                  }
                  frame 12 {
                    n1601 = local read "Elevator Panel"() -> (w3660:T3)
                    n1602 = Bundle By Name(cluster=w3660, "Floor 12"=FALSE ("Call 12")) -> (w3659:T3)
                    n1603 = control-ref of="Floor 12"() -> (w3662:refnum<vi>)
                    n1604 = local write "Elevator Panel"(w3659) -> ()
                    n1605 = property class="Bool (strict)"(reference=w3662, "DisabledEnum"=T7."Enabled" ("Disabled")) -> ()  [unwired: 1 in, 2 out]
                  }
                }
              }
            }
            n1606 = call <vilib>:"Release Semaphore.vi"("error in (no error)"=w3567, "semaphore"=w3568) -> ("error out"=w3570:errorcluster, "semaphore out"=w3569:T8)  [unwired: 4 in]
          }
        }
      }
      frame True {
      }
    }
    n1607 = Wait (ms)(milliseconds to wait=w3028) -> ()  [unwired: 1 out]
  }
  n1608 = call <vilib>:"Release Semaphore Reference.vi"("error in (no error)"=w6, "force destroy? (F)"=TRUE, "semaphore"=w7) -> ()  [unwired: 7 in, 2 out]
  n1609 = Release Queue(queue=w15, force destroy? (F)=TRUE, error in (no error)=w14) -> ()  [unwired: 3 out]
  n1610 = Release Queue(queue=w18, force destroy? (F)=TRUE, error in (no error)=w19) -> ()  [unwired: 3 out]
